vi "BatteryTestParsing.vi"() -> ()   [LabVIEW 2025]
panel:
  in  "Tab Control":enum32{"Page 1", "Page 2"}(tab)
  in  "charging 2":string="b'\\xe4\\xb3#\\xb5r\\x9c' bytearray(b'{\"topic\": \"/battery\", \"value\": 0.0}') {b'\\xe4\\xb3#\\xb5r\\x9c': [-31, 48611074]}\nb'\\xe4\\xb3#\\xb5r\\x9c' bytearray(b'{\"topic\": \"/battery\", \"value\": 0.2}') {b'\\xe4\\xb3#\\xb5r\\x9c': [-28, 48677187]}\nb'\\xe4\\xb3#\\xb5r\\x9c' bytearray(b'{\"topic\": \"/battery\", \"value\": 0.2}') {b'\\xe4\\xb3#\\xb5r\\x9c': [-31, 48743297]}\nb'\\xe4\\xb3#\\xb5r\\x9c' bytearray(b'{\"topic\": \"/battery\", \"value\": 0.7}') {b'\\xe4\\xb3#\\xb5r\\x9c': [-30, 48809408]}\nb'\\xe4\\xb3#\\xb5r\\x9c' bytearray(b'{\"topic\": \"/battery\", \"value\": 1.0}') {b'\\xe4\\xb3#\\xb5r\\x9c': [-40, 48875521]}\nb'\\xe4\\xb3#\\xb5r\\x9c' bytearray(b'{\"topic\": \"/battery\", \"value\": 1.1}') {b'\\xe4\\xb3#\\xb5r\\x9c': [-40, 48941632]}\nb'\\xe4\\xb3#\\xb5r\\x9c' bytearray(b'{\"topic\": \"/battery\", \"value\": 1.2}') {b'\\xe4\\xb3#\\xb5r\\x9c': [-40, 49007743]}\nb'\\xe4\\xb3#\\xb5r\\x9c' bytearray(b'{\"topic\": \"/battery\", \"value\": 1.4}') {b'\\xe4\\xb3#\\xb5r\\x9c': [-40, 49073858]}\nb'\\xe4\\xb3#\\xb5r\\x9c' bytearray(b'{\"topic\": \"/battery\", \"value\": 1.7}') {b'\\xe4\\xb3#\\xb5r\\x9c': [-40, 49139966]}\nb'\\xe4\\xb3#\\xb5r\\x9c' bytearray(b'{\"topic\": \"/battery\", \"value\": 2.0}') {b'\\xe4\\xb3#\\xb5r\\x9c': [-40, 49206079]}\nb'\\xe4\\xb3#\\xb5r\\x9c' bytearray(b'{\"topic\": \"/battery\", \"value\": 2.0}') {b'\\xe4\\xb3#\\xb5r\\x9c': [-40, 49272188]}\nb'\\xe4\\xb3#\\xb5r\\x9c' bytearray(b'{\"topic\": \"/battery\", \"value\": 2.0}') {b'\\xe4\\xb3#\\xb5r\\x9c': [-40, 49338302]}\nb'\\xe4\\xb3#\\xb5r\\x9c' bytearray(b'{\"topic\": \"/battery\", \"value\": 2.0}') {b'\\xe4\\xb3#\\xb5r\\x9c': [-36, 49404411]}\nb'\\xe4\\xb3#\\xb5r\\x9c' bytearray(b'{\"topic\": \"/battery\", \"value\": 2.0}') {b'\\xe4\\xb3#\\xb5r\\x9c': [-40, 49470522]}\nb'\\xe4\\xb3#\\xb5r\\x9c' bytearray(b'{\"topic\": \"/battery\", \"value\": 2.1}') {b'\\xe4\\xb3#\\xb5r\\x9c': [-40, 49536634]}\nb'\\xe4\\xb3#\\xb5r\\x9c' bytearray(b'{\"topic\": \"/battery\", \"value\": 2.1}') {b'\\xe4\\xb3#\\xb5r\\x9c': [-36, 49602745]}\nb'\\xe4\\xb3#\\xb5r\\x9c' bytearray(b'{\"topic\": \"/battery\", \"value\": 2.2}') {b'\\xe4\\xb3#\\xb5r\\x9c': [-36, 49668858]}\nb'\\xe4\\xb3#\\xb5r\\x9c' bytear}') {b'\\xe4\\xb3#\\xb5r\\x9c': [-36, 49734968]}\nb'\\xe4\\xb3#\\xb5r\\x9c' bytearray(b'{\"topic\": \"/battery\", \"value\": 2.3}') {b'\\xe4\\xb3#\\xb5r\\x9c': [-36, 49801080]}\nb'\\xe4\\xb3#\\xb5r\\x9c' bytearray(b'{\"topic\": \"/battery\", \"value\": 2.4}') {b'\\xe4\\xb3#\\xb5r\\x9c': [-39, 49867191]}\nb'\\xe4\\xb3#\\xb5r\\x9c' bytear': [-36, 50065525]}\nb'\\xe4\\xb3#\\xb5r\\x9c' bytearray(b'{\"topic\": \"/battery\", \"value\": 2.8}') {b'\\xe4\\xb3#\\xb5r\\x9c': [-36, 50131636]}\nb'\\xe4\\xb3#\\xb5r\\x9c' bytearray(b'{\"topic\": \"/battery\", \"value\": 2.8}') {b'\\xe4\\xb3#\\xb5r\\x9c': [-38, 50197750]}\nb'\\xe4\\xb3#\\xb5r\\x9c' bytearray(b'{\"topic\": \"/battery\", \"value\": 2.9}') {b'\\xe4\\xb3#\\xb5r\\x9c': [-36, 50263866]}\nb'\\xe4\\xb3#\\xb5r\\x9c' bytearray(b'{\"topic\": \"/battery\", \"value\": 2.9}') {b'\\xe4\\xb3#\\xb5r\\x9c': [-36, 50329983]}\nb'\\xe4\\xb3#\\xb5r\\x9c' bytearray(b'{\"topic\": \"/battery\", \"value\": 2.9}') {b'\\xe4\\xb3#\\xb5r\\x9c': [-36, 50396092]}\nb'\\xe4\\xb3#\\xb5r\\x9c' bytearray(b'{\"topic\": \"/battery\", \"value\": 3.0}') {b'\\xe4\\xb3#\\xb5r\\x9c': [-36, 50462203]}\nb'\\xe4\\xb3#\\xb5r\\x9c' bytearb'\\xe4\\xb3#\\xb5r\\x9c' bytearray(b'{\"topic\": \"/battery\", \"value\": 3.0}') {b'\\xe4\\xb3#\\xb5r\\x9c': [-35, 50792762]}\nb'\\xe4\\xb3#\\xb5r\\x9c' bytearray(b'{\"topic\": \"/battery\", \"value\": 2.9}') {b'\\xe4\\xb3#\\xb5r\\x9c': [-35, 50858871]}\nb'\\xe4\\xb3#\\xb5r\\x9c' bytearray(b'{\"topic\": \"/battery\", \"value\": 3.0}') {b'\\xe4\\xb3#\\xb5r\\x9c': [-35, 50924983]}\nb'\\xe4\\xb3#\\xb5r\\x9c' bytearray(b'{\"topic\": \"/battery\", \"value\": 3.0}') {b'\\xe4\\xb3#\\xb5r\\x9c': [-35, 50991096]}\nb'\\xe4\\xb3#\\xb5r\\x9c' bytearray(b'{\"topic\": \"/battery\", \"value\": 3.0}') {b'\\xe4\\xb3#\\xb5r\\x9c': [-35, 51057206]}\nb'\\xe4\\xb3#\\xb5r\\x9c' bytearray(b'{\"topic\": \"/battery\", \"value\": 3.0}') {b'\\xe4\\xb3#\\xb5r\\x9c': [-31, 51123317]}\nb'\\xe4\\xb3#\\xb5r\\x9c' bytearray(b'{\"topic\": \"/battery\", \"value\": 3.0}') {b'\\xe4\\xb3#\\xb5r\\x9c': [-31, 51189428]}\nb'\\xe4\\xb3#\\xb5r\\x9c' bytearray(b'{\"topic\": \"/battery\", \"value\": 3.0}') {b'\\xe4\\xb3#\\xb5r\\x9c': [-31, 51255540]}\nb'\\xe4\\xb3#\\xb5r\\x9c' bytearray(b'{\"topic\": \"/battery\", \"value\": 3.0}') {b'\\xe4\\xb3#\\xb5r\\x9c': [-30, 51321651]}\nb'\\xe4\\xb3#\\xb5r\\x9c' bytearray(b'{\"topic\": \"/battery\", \"value\": 3.0}') {b'\\xe4\\xb3#\\xb5r\\x9c': [-30, 51387763]}\nb'\\xe4\\xb3#\\xb5r\\x9c' bytearray(b'{\"topic\": \"/battery\", \"value\": 3.0}') {b'\\xe4\\xb3#\\xb5r\\x9c': [-31, 51453874]}\nb'\\xe4\\xb3#\\xb5r\\x9c' bytearray(b'{\"topic\": \"/battery\", \"value\": 3.0}') {b'\\xe4\\xb3#\\xb5r\\x9c': [-30, 51519986]}\nb'\\xe4\\xb3#\\xb5r\\x9c' bytearray(b'{\"topic\": \"/battery\", \"value\": 3.0}') {b'\\xe4\\xb3#\\xb5r\\x9c': [-30, 51586097]}\nb'\\xe4\\xb3#\\xb5r\\x9c' bytearray(b'{\"topic\": \"/battery\", \"value\": 3.1}') {b'\\xe4\\xb3#\\xb5r\\x9c': [-31, 51652210]}\nb'\\xe4\\xb3#\\xb5r\\x9c' bytearray(b'{\"topic\": \"/battery\", \"value\": 3.1}') {b'\\xe4\\xb3#\\xb5r\\x9c': [-31, 51718320]}\nb'\\xe4\\xb3#\\xb5r\\x9c' bytearray(b'{\"topic\": \"/battery\", \"value\": 3.2}') {b'\\xe4\\xb3#\\xb5r\\x9c': [-27, 51784433]}\nb'\\xe4\\xb3#\\xb5r\\x9c' bytearray(b'{\"topic\": \"/battery\", \"value\": 3.3}') {b'\\xe4\\xb3#\\xb5r\\x9c': [-26, 51850543]}\nb'\\xe4\\xb3#\\xb5r\\x9c' bytearray(b'{\"topic\": \"/battery\", \"value\": 3.5}') {b'\\xe4\\xb3#\\xb5r\\x9c': [-27, 51916654]}\nb'\\xe4\\xb3#\\xb5r\\x9c' bytearray(b'{\"topic\": \"/battery\", \"value\": 3.6}') {b'\\xe4\\xb3#\\xb5r\\x9c': [-25, 51982767]}\nb'\\xe4\\xb3#\\xb5r\\x9c' bytearray(b'{\"topic\": \"/battery\", \"value\": 3.7}') {b'\\xe4\\xb3#\\xb5r\\x9c': [-27, 52048877]}\nb'\\xe4\\xb3#\\xb5r\\x9c' bytearray(b'{\"topic\": \"/battery\", \"value\": 3.9}') {b'\\xe4\\xb3#\\xb5r\\x9c': [-25, 52114990]}\nb'\\xe4\\xb3#\\xb5r\\x9c' bytearray(b'{\"topic\": \"/battery\", \"value\": 4.0}') {b'\\xe4\\xb3#\\xb5r\\x9c': [-26, 52181100]}\nb'\\xe4\\xb3#\\xb5r\\x9c' bytearray(b'{\"topic\": \"/battery\", \"value\": 4.0}') {b'\\xe4\\xb3#\\xb5r\\x9c': [-25, 52247211]}\nb'\\xe4\\xb3#\\xb5r\\x9c' bytearray(b'{\"topic\": \"/battery\", \"value\": 4.0}') {b'\\xe4\\xb3#\\xb5r\\x9c': [-27, 52313322]}\nb'\\xe4\\xb3#\\xb5r\\x9c' bytearray(b'{\"topic\": \"/battery\", \"value\": 4.0}') {b'\\xe4\\xb3#\\xb5r\\x9c': [-27, 52379434]}\nb'\\xe4\\xb3#\\xb5r\\x9c' bytearray(b'{\"topic\": \"/battery\", \"value\": 4.0}') {b'\\xe4\\xb3#\\xb5r\\x9c': [-25, 52445546]}\nb'\\xe4\\xb3#\\xb5r\\x9c' bytearray(b'{\"topic\": \"/battery\", \"value\": 4.0}') {b'\\xe4\\xb3#\\xb5r\\x9c': [-26, 52511660]}\nb'\\xe4\\xb3#\\xb5r\\x9c' bytearray(b'{\"topic\": \"/battery\", \"value\": 4.0}') {b'\\xe4\\xb3#\\xb5r\\x9c': [-27, 52577769]}\nb'\\xe4\\xb3#\\xb5r\\x9c' bytearray(b'{\"topic\": \"/battery\", \"value\": 4.0}') {b'\\xe4\\xb3#\\xb5r\\x9c': [-27, 52643879]}\nb'\\xe4\\xb3#\\xb5r\\x9c' bytearray(b'{\"topic\": \"/battery\", \"value\": 4.0}') {b'\\xe4\\xb3#\\xb5r\\x9c': [-26, 52709991]}\nb'\\xe4\\xb3#\\xb5r\\x9c' bytearray(b'{\"topic\": \"/battery\", \"value\": 4.0}') {b'\\xe4\\xb3#\\xb5r\\x9c': [-25, 52776103]}\nb'\\xe4\\xb3#\\xb5r\\x9c' bytearray(b'{\"topic\": \"/battery\", \"value\": 4.0}') {b'\\xe4\\xb3#\\xb5r\\x9c': [-27, 52842213]}\nb'\\xe4\\xb3#\\xb5r\\x9c' bytearray(b'{\"topic\": \"/battery\", \"value\": 4.0}') {b'\\xe4\\xb3#\\xb5r\\x9c': [-27, 52908325]}\nb'\\xe4\\xb3#\\xb5r\\x9c' bytearray(b'{\"topic\": \"/battery\", \"value\": 4.0}') {b'\\xe4\\xb3#\\xb5r\\x9c': [-25, 52974436]}\nb'\\xe4\\xb3#\\xb5r\\x9c' bytearray(b'{\"topic\": \"/battery\", \"value\": 4.0}') {b'\\xe4\\xb3#\\xb5r\\x9c': [-27, 53040550]}\nb'\\xe4\\xb3#\\xb5r\\x9c' bytearray(b'{\"topic\": \"/battery\", \"value\": 4.0}') {b'\\xe4\\xb3#\\xb5r\\x9c': [-25, 53106660]}\nb'\\xe4\\xb3#\\xb5r\\x9c' bytearb'\\xe4\\xb3#\\xb5r\\x9c' bytearray(b'{\"topic\": \"/battery\", \"value\": 4.2}') {b'\\xe4\\xb3#\\xb5r\\x9c': [-25, 53238882]}\nb'\\xe4\\xb3#\\xb5r\\x9c' bytearray(b'{\"topic\": \"/battery\", \"value\": 4.3}') {b'\\xe4\\xb3#\\xb5r\\x9c': [-25, 53304993]}\nb'\\xe4\\xb3#\\xb5r\\x9c' bytearray(b'{\"topic\": \"/battery\", \"value\": 4.4}') {b'\\xe4\\xb3#\\xb5r\\x9c': [-25, 53371105]}\nb'\\xe4\\xb3#\\xb5r\\x9c' bytearpic\": \"/battery\", \"value\": 4.8}') {b'\\xe4\\xb3#\\xb5r\\x9c': [-27, 53635551]}\nb'\\xe4\\xb3#\\xb5r\\x9c' bytearray(b'{\"topic\": \"/battery\", \"value\": 4.9}') {b'\\xe4\\xb3#\\xb5r\\x9c': [-27, 53701662]}\nb'\\xe4\\xb3#\\xb5r\\x9c' bytearray(b'{\"topic\": \"/battery\", \"value\": 5.0}') {b'\\xe4\\xb3#\\xb5r\\x9c': [-25, 53767776]}\nb'\\xe4\\xb3#\\xb5r\\x9c' bytearray(b'{\"topic\": \"/battery\", \"value\": 5.0}') {b'\\xe4\\xb3#\\xb5r\\x9c': [-26, 53833885]}\nb'\\xe4\\xb3#\\xb5r\\x9c' bytearray(b'{\"topic\": \"/battery\", \"value\": 5.0}') {b'\\xe4\\xb3#\\xb5r\\x9c': [-27, 53899998]}\nb'\\xe4\\xb3#\\xb5r\\x9c' bytearray(b'{\"topic\": \"/battery\", \"value\": 5.0}') {b'\\xe4\\xb3#\\xb5r\\x9c': [-26, 53966107]}\nb'\\xe4\\xb3#\\xb5r\\x9c' bytearray(b'{\"topic\": \"/battery\", \"value\": 5.0}') {b'\\xe4\\xb3#\\xb5r\\x9c': [-25, 54032219]}\nb'\\xe4\\xb3#\\xb5r\\x9c' bytearray(b'{\"topic\": \"/battery\", \"value\": 5.0}') {b'\\xe4\\xb3#\\xb5r\\x9c': [-25, 54098330]}\nb'\\xe4\\xb3#\\xb5r\\x9c' bytearray(b'{\"topic\": \"/battery\", \"value\": 5.0}') {b'\\xe4\\xb3#\\xb5r\\x9c': [-27, 54164443]}\nb'\\xe4\\xb3#\\xb5r\\x9c' bytearray(b'{\"topic\": \"/battery\", \"value\": 5.0}') {b'\\xe4\\xb3#\\xb5r\\x9c': [-27, 54230553]}\nb'\\xe4\\xb3#\\xb5r\\x9c' bytearray(b'{\"topic\": \"/battery\", \"value\": 5.0}') {b'\\xe4\\xb3#\\xb5r\\x9c': [-27, 54296665]}\nb'\\xe4\\xb3#\\xb5r\\x9c' bytearray(b'{\"topic\": \"/battery\", \"value\": 5.0}') {b'\\xe4\\xb3#\\xb5r\\x9c': [-25, 54362776]}\nb'\\xe4\\xb3#\\xb5r\\x9c' bytearray(b'{\"topic\": \"/battery\", \"value\": 5.0}') {b'\\xe4\\xb3#\\xb5r\\x9c': [-27, 54428887]}\nb'\\xe4\\xb3#\\xb5r\\x9c' bytearray(b'{\"topic\": \"/battery\", \"value\": 5.0}') {b'\\xe4\\xb3#\\xb5r\\x9c': [-27, 54495000]}\nb'\\xe4\\xb3#\\xb5r\\x9c' bytearray(b'{\"topic\": \"/battery\", \"value\": 5.0}') {b'\\xe4\\xb3#\\xb5r\\x9c': [-25, 54561112]}\nb'\\xe4\\xb3#\\xb5r\\x9c' bytearray(b'{\"topic\": \"/battery\", \"value\": 5.0}') {b'\\xe4\\xb3#\\xb5r\\x9c': [-27, 54627233]}\nb'\\xe4\\xb3#\\xb5r\\x9c' bytearray(b'{\"topic\": \"/battery\", \"value\": 5.0}') {b'\\xe4\\xb3#\\xb5r\\x9c': [-27, 54693354]}\nb'\\xe4\\xb3#\\xb5r\\x9c' bytearray(b'{\"topic\": \"/battery\", \"value\": 5.0}') {b'\\xe4\\xb3#\\xb5r\\x9c': [-25, 54759468]}\nb'\\xe4\\xb3#\\xb5r\\x9c' bytearray(b'{\"topic\": \"/battery\", \"value\": 5.0}') {b'\\xe4\\xb3#\\xb5r\\x9c': [-25, 54825580]}\nb'\\xe4\\xb3#\\xb5r\\x9c' bytearray(b'{\"topic\": \"/battery\", \"value\": 5.0}') {b'\\xe4\\xb3#\\xb5r\\x9c': [-25, 54891687]}\nb'\\xe4\\xb3#\\xb5r\\x9c' bytearray(b'{\"topic\": \"/battery\", \"value\": 5.0}') {b'\\xe4\\xb3#\\xb5r\\x9c': [-26, 54957798]}\nb'\\xe4\\xb3#\\xb5r\\x9c' bytearray(b'{\"topic\": \"/battery\", \"value\": 5.0}') {b'\\xe4\\xb3#\\xb5r\\x9c': [-25, 55023910]}\nb'\\xe4\\xb3#\\xb5r\\x9c' bytearray(b'{\"topic\": \"/battery\", \"value\": 5.0}') {b'\\xe4\\xb3#\\xb5r\\x9c': [-27, 55090021]}\nb'\\xe4\\xb3#\\xb5r\\x9c' bytearray(b'{\"topic\": \"/battery\", \"value\": 5.0}') {b'\\xe4\\xb3#\\xb5r\\x9c': [-25, 55156133]}\nb'\\xe4\\xb3#\\xb5r\\x9c' bytearray(b'{\"topic\": \"/battery\", \"value\": 5.0}') {b'\\xe4\\xb3#\\xb5r\\x9c': [-27, 55222244]}\nb'\\xe4\\xb3#\\xb5r\\x9c' bytearray(b'{\"topic\": \"/battery\", \"value\": 5.1}') {b'\\xe4\\xb3#\\xb5r\\x9c': [-26, 55288355]}\nb'\\xe4\\xb3#\\xb5r\\x9c' bytearray(b'{\"topic\": \"/battery\", \"value\": 5.2}') {b'\\xe4\\xb3#\\xb5r\\x9c': [-27, 55354468]}\nb'\\xe4\\xb3#\\xb5r\\x9c' bytearray(b'{\"topic\": \"/battery\", \"value\": 5.2}') {b'\\xe4\\xb3#\\xb5r\\x9c': [-25, 55420578]}\nb'\\xe4\\xb3#\\xb5r\\x9c' bytearray(b'{\"topic\": \"/battery\", \"value\": 5.3}') {b'\\xe4\\xb3#\\xb5r\\x9c': [-25, 55486690]}\nb'\\xe4\\xb3#\\xb5r\\x9c' bytearray(b'{\"topic\": \"/battery\", \"value\": 5.4}') {b'\\xe4\\xb3#\\xb5r\\x9c': [-27, 55552801]}\nb'\\xe4\\xb3#\\xb5r\\x9c' bytearray(b'{\"topic\": \"/battery\", \"value\": 5.5}') {b'\\xe4\\xb3#\\xb5r\\x9c': [-25, 55618912]}\nb'\\xe4\\xb3#\\xb5r\\x9c' bytearray(b'{\"topic\": \"/battery\", \"value\": 5.6}') {b'\\xe4\\xb3#\\xb5r\\x9c': [-26, 55685025]}\nb'\\xe4\\xb3#\\xb5r\\x9c' bytearray(b'{\"topic\": \"/battery\", \"value\": 5.8}') {b'\\xe4\\xb3#\\xb5r\\x9c': [-25, 55751135]}\nb'\\xe4\\xb3#\\xb5r\\x9c' bytearray(b'{\"topic\": \"/battery\", \"value\": 5.9}') {b'\\xe4\\xb3#\\xb5r\\x9c': [-25, 55817246]}\nb'\\xe4\\xb3#\\xb5r\\x9c' bytearray(b'{\"topic\": \"/battery\", \"value\": 6.0}') {b'\\xe4\\xb3#\\xb5r\\x9c': [-27, 55883358]}\nb'\\xe4\\xb3#\\xb5r\\x9c' bytearray(b'{\"topic\": \"/battery\", \"value\": 6.0}') {b'\\xe4\\xb3#\\xb5r\\x9c': [-26, 55949470]}\nb'\\xe4\\xb3#\\xb5r\\x9c' bytearray(b'{\"topic\": \"/battery\", \"value\": 6.0}') {b'\\xe4\\xb3#\\xb5r\\x9c': [-27, 56015581]}\nb'\\xe4\\xb3#\\xb5r\\x9c' bytearray(b'{\"topic\": \"/battery\", \"value\": 6.1}') {b'\\xe4\\xb3#\\xb5r\\x9c': [-27, 56081693]}\nb'\\xe4\\xb3#\\xb5r\\x9c' bytearray(b'{\"topic\": \"/battery\", \"value\": 6.2}') {b'\\xe4\\xb3#\\xb5r\\x9c': [-25, 56147805]}\nb'\\xe4\\xb3#\\xb5r\\x9c' bytearray(b'{\"topic\": \"/battery\", \"value\": 6.3}') {b'\\xe4\\xb3#\\xb5r\\x9c': [-27, 56213915]}\nb'\\xe4\\xb3#\\xb5r\\x9c' bytearray(b'{\"topic\": \"/battery\", \"value\": 6.4}') {b'\\xe4\\xb3#\\xb5r\\x9c': [-28, 56280026]}\nb'\\xe4\\xb3#\\xb5r\\x9c' bytearray(b'{\"topic\": \"/battery\", \"value\": 6.5}') {b'\\xe4\\xb3#\\xb5r\\x9c': [-27, 56346138]}\nb'\\xe4\\xb3#\\xb5r\\x9c' bytearray(b'{\"topic\": \"/battery\", \"value\": 6.6}') {b'\\xe4\\xb3#\\xb5r\\x9c': [-26, 56412252]}\nb'\\xe4\\xb3#\\xb5r\\x9c' bytearray(b'{\"topic\": \"/battery\", \"value\": 6.7}') {b'\\xe4\\xb3#\\xb5r\\x9c': [-27, 56478360]}\nb'\\xe4\\xb3#\\xb5r\\x9c' bytearray(b'{\"topic\": \"/battery\", \"value\": 6.9}') {b'\\xe4\\xb3#\\xb5r\\x9c': [-27, 56544472]}\nb'\\xe4\\xb3#\\xb5r\\x9c' bytearray(b'{\"topic\": \"/battery\", \"value\": 7.0}') {b'\\xe4\\xb3#\\xb5r\\x9c': [-27, 56610583]}\nb'\\xe4\\xb3#\\xb5r\\x9c' bytearray(b'{\"topic\": \"/battery\", \"value\": 7.2}') {b'\\xe4\\xb3#\\xb5r\\x9c': [-25, 56676696]}\nb'\\xe4\\xb3#\\xb5r\\x9c' bytearray(b'{\"topic\": \"/battery\", \"value\": 7.3}') {b'\\xe4\\xb3#\\xb5r\\x9c': [-27, 56742810]}\nb'\\xe4\\xb3#\\xb5r\\x9c' bytearray(b'{\"topic\": \"/battery\", \"value\": 7.4}') {b'\\xe4\\xb3#\\xb5r\\x9c': [-25, 56808917]}\nb'\\xe4\\xb3#\\xb5r\\x9c' bytearray(b'{\"topic\": \"/battery\", \"value\": 7.6}') {b'\\xe4\\xb3#\\xb5r\\x9c': [-25, 56875029]}\nb'\\xe4\\xb3#\\xb5r\\x9c' bytearray(b'{\"topic\": \"/battery\", \"value\": 7.8}') {b'\\xe4\\xb3#\\xb5r\\x9c': [-25, 56941140]}\nb'\\xe4\\xb3#\\xb5r\\x9c' bytearray(b'{\"topic\": \"/battery\", \"value\": 8.0}') {b'\\xe4\\xb3#\\xb5r\\x9c': [-27, 57007252]}\nb'\\xe4\\xb3#\\xb5r\\x9c' bytearray(b'{\"topic\": \"/battery\", \"value\": 8.2}') {b'\\xe4\\xb3#\\xb5r\\x9c': [-26, 57073364]}\nb'\\xe4\\xb3#\\xb5r\\x9c' bytearray(b'{\"topic\": \"/battery\", \"value\": 8.4}') {b'\\xe4\\xb3#\\xb5r\\x9c': [-26, 57139474]}\nb'\\xe4\\xb3#\\xb5r\\x9c' bytearray(b'{\"topic\": \"/battery\", \"value\": 8.6}') {b'\\xe4\\xb3#\\xb5r\\x9c': [-25, 57205586]}\nb'\\xe4\\xb3#\\xb5r\\x9c' bytearray(b'{\"topic\": \"/battery\", \"value\": 8.9}') {b'\\xe4\\xb3#\\xb5r\\x9c': [-26, 57271697]}\nb'\\xe4\\xb3#\\xb5r\\x9c' bytearray(b'{\"topic\": \"/battery\", \"value\": 9.1}') {b'\\xe4\\xb3#\\xb5r\\x9c': [-25, 57337809]}\nb'\\xe4\\xb3#\\xb5r\\x9c' bytearray(b'{\"topic\": \"/battery\", \"value\": 9.3}') {b'\\xe4\\xb3#\\xb5r\\x9c': [-25, 57403920]}\nb'\\xe4\\xb3#\\xb5r\\x9c' bytearray(b'{\"topic\": \"/battery\", \"value\": 9.6}') {b'\\xe4\\xb3#\\xb5r\\x9c': [-26, 57470032]}\nb'\\xe4\\xb3#\\xb5r\\x9c' bytearray(b'{\"topic\": \"/battery\", \"value\": 9.8}') {b'\\xe4\\xb3#\\xb5r\\x9c': [-25, 57536143]}\nb'\\xe4\\xb3#\\xb5r\\x9c' bytearray(b'{\"topic\": \"/battery\", \"value\": 10.1}') {b'\\xe4\\xb3#\\xb5r\\x9c': [-27, 57602254]}\nb'\\xe4\\xb3#\\xb5r\\x9c' bytearray(b'{\"topic\": \"/battery\", \"value\": 10.4}') {b'\\xe4\\xb3#\\xb5r\\x9c': [-26, 57668366]}\nb'\\xe4\\xb3#\\xb5r\\x9c' bytearray(b'{\"topic\": \"/battery\", \"value\": 10.7}') {b'\\xe4\\xb3#\\xb5r\\x9c': [-26, 57734478]}\nb'\\xe4\\xb3#\\xb5r\\x9c' bytearray(b'{\"topic\": \"/battery\", \"value\": 11.0}') {b'\\xe4\\xb3#\\xb5r\\x9c': [-27, 57800590]}\nb'\\xe4\\xb3#\\xb5r\\x9c' byteb'\\xe4\\xb3#\\xb5r\\x9c' bytearray(b'{\"topic\": \"/battery\", \"value\": 13.0}') {b'\\xe4\\xb3#\\xb5r\\x9c': [-26, 58197260]}\nb'\\xe4\\xb3#\\xb5r\\x9c' bytearray(b'{\"topic\": \"/battery\", \"value\": 13.4}') {b'\\xe4\\xb3#\\xb5r\\x9c': [-25, 58263372]}\nb'\\xe4\\xb3#\\xb5r\\x9c' bytearray(b'{\"topic\": \"/battery\", \"value\": 13.7}') {b'\\xe4\\xb3#\\xb5r\\x9c': [-26, 58329480]}\nb'\\xe4\\xb3#\\xb5r\\x9c' bytearray(b'{\"topic\": \"/battery\", \"value\": 14.1}') {b'\\xe4\\xb3#\\xb5r\\x9c': [-26, 58395591]}\nb'\\xe4\\xb3#\\xb5r\\x9c' bytearray(b'{\"topic\": \"/battery\", \"value\": 14.5}') {b'\\xe4\\xb3#\\xb5r\\x9c': [-26, 58461702]}\nb'\\xe4\\xb3#\\xb5r\\x9c' byteb'\\xe4\\xb3#\\xb5r\\x9c' bytearray(b'{\"topic\": \"/battery\", \"value\": 15.3}') {b'\\xe4\\xb3#\\xb5r\\x9c': [-26, 58593925]}\nb'\\xe4\\xb3#\\xb5r\\x9c' bytearray(b'{\"topic\": \"/battery\", \"value\": 15.7}') {b'\\xe4\\xb3#\\xb5r\\x9c': [-26, 58660043]}\nb'\\xe4\\xb3#\\xb5r\\x9c' bytearray(b'{\"topic\": \"/battery\", \"value\": 16.1}') {b'\\xe4\\xb3#\\xb5r\\x9c': [-26, 58726158]}\nb'\\xe4\\xb3#\\xb5r\\x9c' bytearray(b'{\"topic\": \"/battery\", \"value\": 16.5}') {b'\\xe4\\xb3#\\xb5r\\x9c': [-26, 58792269]}\nb'\\xe4\\xb3#\\xb5r\\x9c' bytearray(b'{\"topic\": \"/battery\", \"value\": 17.0}') {b'\\xe4\\xb3#\\xb5r\\x9c': [-25, 58858382]}\nb'\\xe4\\xb3#\\xb5r\\x9c' bytearray(b'{\"topic\": \"/battery\", \"value\": 17.4}') {b'\\xe4\\xb3#\\xb5r\\x9c': [-25, 58924492]}\nb'\\xe4\\xb3#\\xb5r\\x9c' bytearray(b'{\"topic\": \"/battery\", \"value\": 17.8}') {b'\\xe4\\xb3#\\xb5r\\x9c': [-25, 58990604]}\nb'\\xe4\\xb3#\\xb5r\\x9c' bytearray(b'{\"topic\": \"/battery\", \"value\": 18.3}') {b'\\xe4\\xb3#\\xb5r\\x9c': [-25, 59056715]}\nb'\\xe4\\xb3#\\xb5r\\x9c' bytearray(b'{\"topic\": \"/battery\", \"value\": 18.7}') {b'\\xe4\\xb3#\\xb5r\\x9c': [-24, 59122826]}\nb'\\xe4\\xb3#\\xb5r\\x9c' bytearray(b'{\"topic\": \"/battery\", \"value\": 19.2}') {b'\\xe4\\xb3#\\xb5r\\x9c': [-25, 59188939]}\nb'\\xe4\\xb3#\\xb5r\\x9c' bytearray(b'{\"topic\": \"/battery\", \"value\": 19.6}') {b'\\xe4\\xb3#\\xb5r\\x9c': [-26, 59255051]}\nb'\\xe4\\xb3#\\xb5r\\x9c' bytearray(b'{\"topic\": \"/battery\", \"value\": 20.1}') {b'\\xe4\\xb3#\\xb5r\\x9c': [-26, 59321161]}\nb'\\xe4\\xb3#\\xb5r\\x9c' bytearray(b'{\"topic\": \"/battery\", \"value\": 20.6}') {b'\\xe4\\xb3#\\xb5r\\x9c': [-25, 59387272]}\nb'\\xe4\\xb3#\\xb5r\\x9c' bytearray(b'{\"topic\": \"/battery\", \"value\": 21.0}') {b'\\xe4\\xb3#\\xb5r\\x9c': [-25, 59453383]}\nb'\\xe4\\xb3#\\xb5r\\x9c' bytearray(b'{\"topic\": \"/battery\", \"value\": 21.5}') {b'\\xe4\\xb3#\\xb5r\\x9c': [-26, 59519495]}\nb'\\xe4\\xb3#\\xb5r\\x9c' bytearray(b'{\"topic\": \"/battery\", \"value\": 22.0}') {b'\\xe4\\xb3#\\xb5r\\x9c': [-25, 59585608]}\nb'\\xe4\\xb3#\\xb5r\\x9c' bytearray(b'{\"topic\": \"/battery\", \"value\": 22.5}') {b'\\xe4\\xb3#\\xb5r\\x9c': [-26, 59651718]}\nb'\\xe4\\xb3#\\xb5r\\x9c' bytearray(b'{\"topic\": \"/battery\", \"value\": 23.0}') {b'\\xe4\\xb3#\\xb5r\\x9c': [-26, 59717829]}\nb'\\xe4\\xb3#\\xb5r\\x9c' bytearray(b'{\"topic\": \"/battery\", \"value\": 23.5}') {b'\\xe4\\xb3#\\xb5r\\x9c': [-26, 59783941]}\nb'\\xe4\\xb3#\\xb5r\\x9c' bytearray(b'{\"topic\": \"/battery\", \"value\": 24.1}') {b'\\xe4\\xb3#\\xb5r\\x9c': [-25, 59850052]}\nb'\\xe4\\xb3#\\xb5r\\x9c' bytearray(b'{\"topic\": \"/battery\", \"value\": 24.6}') {b'\\xe4\\xb3#\\xb5r\\x9c': [-26, 59916164]}\nb'\\xe4\\xb3#\\xb5r\\x9c' bytearray(b'{\"topic\": \"/battery\", \"value\": 25.2}') {b'\\xe4\\xb3#\\xb5r\\x9c': [-25, 59982275]}\nb'\\xe4\\xb3#\\xb5r\\x9c' bytearray(b'{\"topic\": \"/battery\", \"value\": 25.7}') {b'\\xe4\\xb3#\\xb5r\\x9c': [-26, 60048387]}\nb'\\xe4\\xb3#\\xb5r\\x9c' bytearray(b'{\"topic\": \"/battery\", \"value\": 26.3}') {b'\\xe4\\xb3#\\xb5r\\x9c': [-25, 60114498]}\nb'\\xe4\\xb3#\\xb5r\\x9c' bytearray(b'{\"topic\": \"/battery\", \"value\": 26.8}') {b'\\xe4\\xb3#\\xb5r\\x9c': [-25, 60180609]}\nb'\\xe4\\xb3#\\xb5r\\x9c' bytearray(b'{\"topic\": \"/battery\", \"value\": 27.4}') {b'\\xe4\\xb3#\\xb5r\\x9c': [-26, 60246720]}\nb'\\xe4\\xb3#\\xb5r\\x9c' bytearray(b'{\"topic\": \"/battery\", \"value\": 28.0}') {b'\\xe4\\xb3#\\xb5r\\x9c': [-25, 60312838]}\nb'\\xe4\\xb3#\\xb5r\\x9c' bytearray(b'{\"topic\": \"/battery\", \"value\": 28.6}') {b'\\xe4\\xb3#\\xb5r\\x9c': [-24, 60378954]}\nb'\\xe4\\xb3#\\xb5r\\x9c' bytearray(b'{\"topic\": \"/battery\", \"value\": 29.2}') {b'\\xe4\\xb3#\\xb5r\\x9c': [-25, 60445064]}\nb'\\xe4\\xb3#\\xb5r\\x9c' bytearray(b'{\"topic\": \"/battery\", \"value\": 29.8}') {b'\\xe4\\xb3#\\xb5r\\x9c': [-26, 60511176]}\nb'\\xe4\\xb3#\\xb5r\\x9c' bytearray(b'{\"topic\": \"/battery\", \"value\": 30.4}') {b'\\xe4\\xb3#\\xb5r\\x9c': [-25, 60577287]}\nb'\\xe4\\xb3#\\xb5r\\x9c' bytearray(b'{\"topic\": \"/battery\", \"value\": 31.0}') {b'\\xe4\\xb3#\\xb5r\\x9c': [-26, 60643399]}\nb'\\xe4\\xb3#\\xb5r\\x9c' bytearray(b'{\"topic\": \"/battery\", \"value\": 31.7}') {b'\\xe4\\xb3#\\xb5r\\x9c': [-25, 60709515]}\nb'\\xe4\\xb3#\\xb5r\\x9c' bytearray(b'{\"topic\": \"/battery\", \"value\": 32.3}') {b'\\xe4\\xb3#\\xb5r\\x9c': [-24, 60775621]}\nb'\\xe4\\xb3#\\xb5r\\x9c' bytearray(b'{\"topic\": \"/battery\", \"value\": 33.0}') {b'\\xe4\\xb3#\\xb5r\\x9c': [-26, 60841734]}\nb'\\xe4\\xb3#\\xb5r\\x9c' bytearray(b'{\"topic\": \"/battery\", \"value\": 33.6}') {b'\\xe4\\xb3#\\xb5r\\x9c': [-26, 60907845]}\nb'\\xe4\\xb3#\\xb5r\\x9c' bytearray(b'{\"topic\": \"/battery\", \"value\": 34.3}') {b'\\xe4\\xb3#\\xb5r\\x9c': [-25, 60973957]}\nb'\\xe4\\xb3#\\xb5r\\x9c' bytearray(b'{\"topic\": \"/battery\", \"value\": 35.0}') {b'\\xe4\\xb3#\\xb5r\\x9c': [-26, 61040068]}\nb'\\xe4\\xb3#\\xb5r\\x9c' bytearray(b'{\"topic\": \"/battery\", \"value\": 35.6}') {b'\\xe4\\xb3#\\xb5r\\x9c': [-26, 61106181]}\nb'\\xe4\\xb3#\\xb5r\\x9c' bytearray(b'{\"topic\": \"/battery\", \"value\": 36.3}') {b'\\xe4\\xb3#\\xb5r\\x9c': [-25, 61172295]}\nb'\\xe4\\xb3#\\xb5r\\x9c' bytearray(b'{\"topic\": \"/battery\", \"value\": 37.0}') {b'\\xe4\\xb3#\\xb5r\\x9c': [-26, 61238408]}\nb'\\xe4\\xb3#\\xb5r\\x9c' bytearray(b'{\"topic\": \"/battery\", \"value\": 37.7}') {b'\\xe4\\xb3#\\xb5r\\x9c': [-25, 61304522]}\nb'\\xe4\\xb3#\\xb5r\\x9c' bytearray(b'{\"topic\": \"/battery\", \"value\": 38.4}') {b'\\xe4\\xb3#\\xb5r\\x9c': [-26, 61370635]}\nb'\\xe4\\xb3#\\xb5r\\x9c' bytearray(b'{\"topic\": \"/battery\", \"value\": 39.1}') {b'\\xe4\\xb3#\\xb5r\\x9c': [-26, 61436745]}\nb'\\xe4\\xb3#\\xb5r\\x9c' bytearray(b'{\"topic\": \"/battery\", \"value\": 39.8}') {b'\\xe4\\xb3#\\xb5r\\x9c': [-25, 61502857]}\nb'\\xe4\\xb3#\\xb5r\\x9c' bytearray(b'{\"topic\": \"/battery\", \"value\": 40.5}') {b'\\xe4\\xb3#\\xb5r\\x9c': [-26, 61568968]}\nb'\\xe4\\xb3#\\xb5r\\x9c' bytearray(b'{\"topic\": \"/battery\", \"value\": 41.3}') {b'\\xe4\\xb3#\\xb5r\\x9c': [-24, 61635079]}\nb'\\xe4\\xb3#\\xb5r\\x9c' bytearray(b'{\"topic\": \"/battery\", \"value\": 42.0}') {b'\\xe4\\xb3#\\xb5r\\x9c': [-26, 61701191]}\nb'\\xe4\\xb3#\\xb5r\\x9c' bytearray(b'{\"topic\": \"/battery\", \"value\": 42.7}') {b'\\xe4\\xb3#\\xb5r\\x9c': [-26, 61767302]}\nb'\\xe4\\xb3#\\xb5r\\x9c' bytearray(b'{\"topic\": \"/battery\", \"value\": 43.4}') {b'\\xe4\\xb3#\\xb5r\\x9c': [-25, 61833414]}\nb'\\xe4\\xb3#\\xb5r\\x9c' bytearray(b'{\"topic\": \"/battery\", \"value\": 44.2}') {b'\\xe4\\xb3#\\xb5r\\x9c': [-26, 61899525]}\nb'\\xe4\\xb3#\\xb5r\\x9c' bytearray(b'{\"topic\": \"/battery\", \"value\": 44.9}') {b'\\xe4\\xb3#\\xb5r\\x9c': [-25, 61965638]}\nb'\\xe4\\xb3#\\xb5r\\x9c' bytearray(b'{\"topic\": \"/battery\", \"value\": 45.6}') {b'\\xe4\\xb3#\\xb5r\\x9c': [-26, 62031748]}\nb'\\xe4\\xb3#\\xb5r\\x9c' bytearray(b'{\"topic\": \"/battery\", \"value\": 46.3}') {b'\\xe4\\xb3#\\xb5r\\x9c': [-26, 62097859]}\nb'\\xe4\\xb3#\\xb5r\\x9c' bytearray(b'{\"topic\": \"/battery\", \"value\": 47.0}') {b'\\xe4\\xb3#\\xb5r\\x9c': [-26, 62163971]}\nb'\\xe4\\xb3#\\xb5r\\x9c' bytearray(b'{\"topic\": \"/battery\", \"value\": 47.7}') {b'\\xe4\\xb3#\\xb5r\\x9c': [-25, 62230082]}\nb'\\xe4\\xb3#\\xb5r\\x9c' bytearray(b'{\"topic\": \"/battery\", \"value\": 48.5}') {b'\\xe4\\xb3#\\xb5r\\x9c': [-24, 62296194]}\nb'\\xe4\\xb3#\\xb5r\\x9c' bytearray(b'{\"topic\": \"/battery\", \"value\": 49.2}') {b'\\xe4\\xb3#\\xb5r\\x9c': [-26, 62362305]}\nb'\\xe4\\xb3#\\xb5r\\x9c' bytearray(b'{\"topic\": \"/battery\", \"value\": 49.9}') {b'\\xe4\\xb3#\\xb5r\\x9c': [-26, 62428416]}\nb'\\xe4\\xb3#\\xb5r\\x9c' bytearray(b'{\"topic\": \"/battery\", \"value\": 50.6}') {b'\\xe4\\xb3#\\xb5r\\x9c': [-25, 62494528]}\nb'\\xe4\\xb3#\\xb5r\\x9c' bytearray(b'{\"topic\": \"/battery\", \"value\": 51.3}') {b'\\xe4\\xb3#\\xb5r\\x9c': [-25, 62560640]}\nb'\\xe4\\xb3#\\xb5r\\x9c' bytearray(b'{\"topic\": \"/battery\", \"value\": 52.0}') {b'\\xe4\\xb3#\\xb5r\\x9c': [-26, 62626751]}\nb'\\xe4\\xb3#\\xb5r\\x9c' bytearray(b'{\"topic\": \"/battery\", \"value\": 52.7}') {b'\\xe4\\xb3#\\xb5r\\x9c': [-25, 62692862]}\nb'\\xe4\\xb3#\\xb5r\\x9c' bytearray(b'{\"topic\": \"/battery\", \"value\": 53.4}') {b'\\xe4\\xb3#\\xb5r\\x9c': [-25, 62758973]}\nb'\\xe4\\xb3#\\xb5r\\x9c' bytearray(b'{\"topic\": \"/battery\", \"value\": 54.1}') {b'\\xe4\\xb3#\\xb5r\\x9c': [-26, 62825085]}\nb'\\xe4\\xb3#\\xb5r\\x9c' bytearray(b'{\"topic\": \"/battery\", \"value\": 54.8}') {b'\\xe4\\xb3#\\xb5r\\x9c': [-26, 62891196]}\nb'\\xe4\\xb3#\\xb5r\\x9c' bytearray(b'{\"topic\": \"/battery\", \"value\": 55.5}') {b'\\xe4\\xb3#\\xb5r\\x9c': [-26, 62957312]}\nb'\\xe4\\xb3#\\xb5r\\x9c' bytearray(b'{\"topic\": \"/battery\", \"value\": 56.2}') {b'\\xe4\\xb3#\\xb5r\\x9c': [-19, 63023419]}\nb'\\xe4\\xb3#\\xb5r\\x9c' bytearray(b'{\"topic\": \"/battery\", \"value\": 56.9}') {b'\\xe4\\xb3#\\xb5r\\x9c': [-20, 63089530]}\nb'\\xe4\\xb3#\\xb5r\\x9c' bytearray(b'{\"topic\": \"/battery\", \"value\": 57.6}') {b'\\xe4\\xb3#\\xb5r\\x9c': [-20, 63155642]}\nb'\\xe4\\xb3#\\xb5r\\x9c' bytearray(b'{\"topic\": \"/battery\", \"value\": 58.3}') {b'\\xe4\\xb3#\\xb5r\\x9c': [-20, 63221755]}\nb'\\xe4\\xb3#\\xb5r\\x9c' bytearray(b'{\"topic\": \"/battery\", \"value\": 59.0}') {b'\\xe4\\xb3#\\xb5r\\x9c': [-20, 63287867]}\nb'\\xe4\\xb3#\\xb5r\\x9c' bytearray(b'{\"topic\": \"/battery\", \"value\": 59.6}') {b'\\xe4\\xb3#\\xb5r\\x9c': [-18, 63353976]}\nb'\\xe4\\xb3#\\xb5r\\x9c' bytearray(b'{\"topic\": \"/battery\", \"value\": 60.3}') {b'\\xe4\\xb3#\\xb5r\\x9c': [-18, 63420088]}\nb'\\xe4\\xb3#\\xb5r\\x9c' bytearray(b'{\"topic\": \"/battery\", \"value\": 61.0}') {b'\\xe4\\xb3#\\xb5r\\x9c': [-19, 63486199]}\nb'\\xe4\\xb3#\\xb5r\\x9c' bytearray(b'{\"topic\": \"/battery\", \"value\": 61.7}') {b'\\xe4\\xb3#\\xb5r\\x9c': [-18, 63552311]}\nb'\\xe4\\xb3#\\xb5r\\x9c' bytearray(b'{\"topic\": \"/battery\", \"value\": 62.4}') {b'\\xe4\\xb3#\\xb5r\\x9c': [-18, 63618422]}\nb'\\xe4\\xb3#\\xb5r\\x9c' bytearray(b'{\"topic\": \"/battery\", \"value\": 63.1}') {b'\\xe4\\xb3#\\xb5r\\x9c': [-19, 63684533]}\nb'\\xe4\\xb3#\\xb5r\\x9c' bytearray(b'{\"topic\": \"/battery\", \"value\": 63.8}') {b'\\xe4\\xb3#\\xb5r\\x9c': [-19, 63750646]}\nb'\\xe4\\xb3#\\xb5r\\x9c' bytearray(b'{\"topic\": \"/battery\", \"value\": 64.5}') {b'\\xe4\\xb3#\\xb5r\\x9c': [-18, 63816756]}\nb'\\xe4\\xb3#\\xb5r\\x9c' bytearray(b'{\"topic\": \"/battery\", \"value\": 65.2}') {b'\\xe4\\xb3#\\xb5r\\x9c': [-19, 63882867]}\nb'\\xe4\\xb3#\\xb5r\\x9c' bytearray(b'{\"topic\": \"/battery\", \"value\": 65.9}') {b'\\xe4\\xb3#\\xb5r\\x9c': [-22, 63948978]}\nb'\\xe4\\xb3#\\xb5r\\x9c' bytearray(b'{\"topic\": \"/battery\", \"value\": 66.5}') {b'\\xe4\\xb3#\\xb5r\\x9c': [-21, 64015090]}\nb'\\xe4\\xb3#\\xb5r\\x9c' bytearray(b'{\"topic\": \"/battery\", \"value\": 67.2}') {b'\\xe4\\xb3#\\xb5r\\x9c': [-21, 64081205]}\nb'\\xe4\\xb3#\\xb5r\\x9c' bytearray(b'{\"topic\": \"/battery\", \"value\": 67.9}') {b'\\xe4\\xb3#\\xb5r\\x9c': [-20, 64147314]}\nb'\\xe4\\xb3#\\xb5r\\x9c' bytearray(b'{\"topic\": \"/battery\", \"value\": 68.6}') {b'\\xe4\\xb3#\\xb5r\\x9c': [-20, 64213424]}\nb'\\xe4\\xb3#\\xb5r\\x9c' bytearray(b'{\"topic\": \"/battery\", \"value\": 69.3}') {b'\\xe4\\xb3#\\xb5r\\x9c': [-20, 64279536]}\nb'\\xe4\\xb3#\\xb5r\\x9c' bytearray(b'{\"topic\": \"/battery\", \"value\": 70.0}') {b'\\xe4\\xb3#\\xb5r\\x9c': [-20, 64345648]}\nb'\\xe4\\xb3#\\xb5r\\x9c' bytearray(b'{\"topic\": \"/battery\", \"value\": 70.7}') {b'\\xe4\\xb3#\\xb5r\\x9c': [-20, 64411762]}\nb'\\xe4\\xb3#\\xb5r\\x9c' bytearray(b'{\"topic\": \"/battery\", \"value\": 71.4}') {b'\\xe4\\xb3#\\xb5r\\x9c': [-20, 64477871]}\nb'\\xe4\\xb3#\\xb5r\\x9c' bytearray(b'{\"topic\": \"/battery\", \"value\": 72.0}') {b'\\xe4\\xb3#\\xb5r\\x9c': [-20, 64543981]}\nb'\\xe4\\xb3#\\xb5r\\x9c' bytearray(b'{\"topic\": \"/battery\", \"value\": 72.7}') {b'\\xe4\\xb3#\\xb5r\\x9c': [-20, 64610093]}\nb'\\xe4\\xb3#\\xb5r\\x9c' bytearray(b'{\"topic\": \"/battery\", \"value\": 73.3}') {b'\\xe4\\xb3#\\xb5r\\x9c': [-20, 64676204]}\nb'\\xe4\\xb3#\\xb5r\\x9c' bytearray(b'{\"topic\": \"/battery\", \"value\": 74.0}') {b'\\xe4\\xb3#\\xb5r\\x9c': [-20, 64742316]}\nb'\\xe4\\xb3#\\xb5r\\x9c' bytearray(b'{\"topic\": \"/battery\", \"value\": 74.6}') {b'\\xe4\\xb3#\\xb5r\\x9c': [-20, 64808430]}\nb'\\xe4\\xb3#\\xb5r\\x9c' bytearray(b'{\"topic\": \"/battery\", \"value\": 75.2}') {b'\\xe4\\xb3#\\xb5r\\x9c': [-20, 64874538]}\nb'\\xe4\\xb3#\\xb5r\\x9c' byteb3#\\xb5r\\x9c' bytearray(b'{\"topic\": \"/battery\", \"value\": 79.9}') {b'\\xe4\\xb3#\\xb5r\\x9c': [-20, 65403429]}\nb'\\xe4\\xb3#\\xb5r\\x9c' bytearray(b'{\"topic\": \"/battery\", \"value\": 80.4}') {b'\\xe4\\xb3#\\xb5r\\x9c': [-20, 65469541]}\nb'\\xe4\\xb3#\\xb5r\\x9c' bytearray(b'{\"topic\": \"/battery\", \"value\": 81.0}') {b'\\xe4\\xb3#\\xb5r\\x9c': [-20, 65535653]}\nb'\\xe4\\xb3#\\xb5r\\x9c' byte\", \"value\": 81.5}') {b'\\xe4\\xb3#\\xb5r\\x9c': [-20, 65601763]}\nb'\\xe4\\xb3#\\xb5r\\x9c' bytearray(b'{\"topic\": \"/battery\", \"value\": 82.1}') {b'\\xe4\\xb3#\\xb5r\\x9c': [-20, 65667875]}\nb'\\xe4\\xb3#\\xb5r\\x9c' bytearray(b'{\"topic\": \"/battery\", \"value\": 82.6}') {b'\\xe4\\xb3#\\xb5r\\x9c': [-20, 65733988]}\nb'\\xe4\\xb3#\\xb5r\\x9c' bytearray(b'{\"topic\": \"/battery\", \"value\": 83.1}') {b'\\xe4\\xb3#\\xb5r\\x9c': [-20, 65800098]}\nb'\\xe4\\xb3#\\xb5r\\x9c' bytearray(b'{\"topic\": \"/battery\", \"value\": 83.7}') {b'\\xe4\\xb3#\\xb5r\\x9c': [-20, 65866209]}\nb'\\xe4\\xb3#\\xb5r\\x9c' bytearray(b'{\"topic\": \"/battery\", \"value\": 84.2}') {b'\\xe4\\xb3#\\xb5r\\x9c': [-20, 65932321]}\nb'\\xe4\\xb3#\\xb5r\\x9c' bytearray(b'{\"topic\": \"/battery\", \"value\": 84.7}') {b'\\xe4\\xb3#\\xb5r\\x9c': [-20, 65998434]}\nb'\\xe4\\xb3#\\xb5r\\x9c' bytearray(b'{\"topic\": \"/battery\", \"value\": 85.2}') {b'\\xe4\\xb3#\\xb5r\\x9c': [-20, 66064543]}\nb'\\xe4\\xb3#\\xb5r\\x9c' bytearray(b'{\"topic\": \"/battery\", \"value\": 85.8}') {b'\\xe4\\xb3#\\xb5r\\x9c': [-20, 66130655]}\nb'\\xe4\\xb3#\\xb5r\\x9c' bytearray(b'{\"topic\": \"/battery\", \"value\": 86.3}') {b'\\xe4\\xb3#\\xb5r\\x9c': [-20, 66196766]}\nb'\\xe4\\xb3#\\xb5r\\x9c' bytearray(b'{\"topic\": \"/battery\", \"value\": 86.8}') {b'\\xe4\\xb3#\\xb5r\\x9c': [-20, 66262877]}\nb'\\xe4\\xb3#\\xb5r\\x9c' bytearray(b'{\"topic\": \"/battery\", \"value\": 87.3}') {b'\\xe4\\xb3#\\xb5r\\x9c': [-20, 66328990]}\nb'\\xe4\\xb3#\\xb5r\\x9c' bytearray(b'{\"topic\": \"/battery\", \"value\": 87.9}') {b'\\xe4\\xb3#\\xb5r\\x9c': [-20, 66395100]}\nb'\\xe4\\xb3#\\xb5r\\x9c' bytearray(b'{\"topic\": \"/battery\", \"value\": 88.4}') {b'\\xe4\\xb3#\\xb5r\\x9c': [-20, 66461212]}\nb'\\xe4\\xb3#\\xb5r\\x9c' bytearray(b'{\"topic\": \"/battery\", \"value\": 88.9}') {b'\\xe4\\xb3#\\xb5r\\x9c': [-20, 66527323]}\nb'\\xe4\\xb3#\\xb5r\\x9c' bytearray(b'{\"topic\": \"/battery\", \"value\": 89.5}') {b'\\xe4\\xb3#\\xb5r\\x9c': [-20, 66593434]}\nb'\\xe4\\xb3#\\xb5r\\x9c' bytearray(b'{\"topic\": \"/battery\", \"value\": 90.0}') {b'\\xe4\\xb3#\\xb5r\\x9c': [-20, 66659546]}\nb'\\xe4\\xb3#\\xb5r\\x9c' bytearray(b'{\"topic\": \"/battery\", \"value\": 90.5}') {b'\\xe4\\xb3#\\xb5r\\x9c': [-20, 66725657]}\nb'\\xe4\\xb3#\\xb5r\\x9c' bytearray(b'{\"topic\": \"/battery\", \"value\": 91.0}') {b'\\xe4\\xb3#\\xb5r\\x9c': [-20, 66791769]}\nb'\\xe4\\xb3#\\xb5r\\x9c' bytearray(b'{\"topic\": \"/battery\", \"value\": 91.4}') {b'\\xe4\\xb3#\\xb5r\\x9c': [-20, 66857880]}\nb'\\xe4\\xb3#\\xb5r\\x9c' bytearray(b'{\"topic\": \"/battery\", \"value\": 91.9}') {b'\\xe4\\xb3#\\xb5r\\x9c': [-20, 66923991]}\nb'\\xe4\\xb3#\\xb5r\\x9c' bytearray(b'{\"topic\": \"/battery\", \"value\": 92.3}') {b'\\xe4\\xb3#\\xb5r\\x9c': [-20, 66990107]}\nb'\\xe4\\xb3#\\xb5r\\x9c' bytearray(b'{\"topic\": \"/battery\", \"value\": 92.8}') {b'\\xe4\\xb3#\\xb5r\\x9c': [-20, 67056214]}\nb'\\xe4\\xb3#\\xb5r\\x9c' bytearray(b'{\"topic\": \"/battery\", \"value\": 93.2}') {b'\\xe4\\xb3#\\xb5r\\x9c': [-20, 67122326]}\nb'\\xe4\\xb3#\\xb5r\\x9c' bytearray(b'{\"topic\": \"/battery\", \"value\": 93.5}') {b'\\xe4\\xb3#\\xb5r\\x9c': [-20, 67188437]}\nb'\\xe4\\xb3#\\xb5r\\x9c' bytearray(b'{\"topic\": \"/battery\", \"value\": 93.9}') {b'\\xe4\\xb3#\\xb5r\\x9c': [-20, 67254548]}\nb'\\xe4\\xb3#\\xb5r\\x9c' bytearray(b'{\"topic\": \"/battery\", \"value\": 94.3}') {b'\\xe4\\xb3#\\xb5r\\x9c': [-20, 67320660]}\nb'\\xe4\\xb3#\\xb5r\\x9c' bytearray(b'{\"topic\": \"/battery\", \"value\": 94.6}') {b'\\xe4\\xb3#\\xb5r\\x9c': [-20, 67386771]}\nb'\\xe4\\xb3#\\xb5r\\x9c' bytearray(b'{\"topic\": \"/battery\", \"value\": 94.9}') {b'\\xe4\\xb3#\\xb5r\\x9c': [-20, 67452885]}\nb'\\xe4\\xb3#\\xb5r\\x9c' bytearray(b'{\"topic\": \"/battery\", \"value\": 95.3}') {b'\\xe4\\xb3#\\xb5r\\x9c': [-20, 67518994]}\nb'\\xe4\\xb3#\\xb5r\\x9c' bytearray(b'{\"topic\": \"/battery\", \"value\": 95.6}') {b'\\xe4\\xb3#\\xb5r\\x9c': [-20, 67585105]}\nb'\\xe4\\xb3#\\xb5r\\x9c' bytearray(b'{\"topic\": \"/battery\", \"value\": 95.9}') {b'\\xe4\\xb3#\\xb5r\\x9c': [-20, 67651217]}\nb'\\xe4\\xb3#\\xb5r\\x9c' bytearray(b'{\"topic\": \"/battery\", \"value\": 96.1}') {b'\\xe4\\xb3#\\xb5r\\x9c': [-20, 67717328]}\nb'\\xe4\\xb3#\\xb5r\\x9c' bytearray(b'{\"topic\": \"/battery\", \"value\": 96.3}') {b'\\xe4\\xb3#\\xb5r\\x9c': [-20, 67783439]}\nb'\\xe4\\xb3#\\xb5r\\x9c' bytearray(b'{\"topic\": \"/battery\", \"value\": 96.5}') {b'\\xe4\\xb3#\\xb5r\\x9c': [-20, 67849551]}\nb'\\xe4\\xb3#\\xb5r\\x9c' bytearray(b'{\"topic\": \"/battery\", \"value\": 96.7}') {b'\\xe4\\xb3#\\xb5r\\x9c': [-20, 67915662]}\nb'\\xe4\\xb3#\\xb5r\\x9c' bytearray(b'{\"topic\": \"/battery\", \"value\": 96.9}') {b'\\xe4\\xb3#\\xb5r\\x9c': [-20, 67981774]}\nb'\\xe4\\xb3#\\xb5r\\x9c' bytearray(b'{\"topic\": \"/battery\", \"value\": 97.0}') {b'\\xe4\\xb3#\\xb5r\\x9c': [-20, 68047885]}\nb'\\xe4\\xb3#\\xb5r\\x9c' bytearray(b'{\"topic\": \"/battery\", \"value\": 97.1}') {b'\\xe4\\xb3#\\xb5r\\x9c': [-20, 68113997]}\nb'\\xe4\\xb3#\\xb5r\\x9c' bytearray(b'{\"topic\": \"/battery\", \"value\": 97.3}') {b'\\xe4\\xb3#\\xb5r\\x9c': [-20, 68180108]}\nb'\\xe4\\xb3#\\xb5r\\x9c' bytearray(b'{\"topic\": \"/battery\", \"value\": 97.4}') {b'\\xe4\\xb3#\\xb5r\\x9c': [-20, 68246221]}\nb'\\xe4\\xb3#\\xb5r\\x9c' bytearray(b'{\"topic\": \"/battery\", \"value\": 97.5}') {b'\\xe4\\xb3#\\xb5r\\x9c': [-20, 68312331]}\nb'\\xe4\\xb3#\\xb5r\\x9c' bytearray(b'{\"topic\": \"/battery\", \"value\": 97.6}') {b'\\xe4\\xb3#\\xb5r\\x9c': [-20, 68378442]}\nb'\\xe4\\xb3#\\xb5r\\x9c' bytearray(b'{\"topic\": \"/battery\", \"value\": 97.7}') {b'\\xe4\\xb3#\\xb5r\\x9c': [-20, 68444553]}\nb'\\xe4\\xb3#\\xb5r\\x9c' bytearray(b'{\"topic\": \"/battery\", \"value\": 97.8}') {b'\\xe4\\xb3#\\xb5r\\x9c': [-20, 68510665]}\nb'\\xe4\\xb3#\\xb5r\\x9c' bytearray(b'{\"topic\": \"/battery\", \"value\": 98.0}') {b'\\xe4\\xb3#\\xb5r\\x9c': [-20, 68576776]}\nb'\\xe4\\xb3#\\xb5r\\x9c' bytearray(b'{\"topic\": \"/battery\", \"value\": 98.0}') {b'\\xe4\\xb3#\\xb5r\\x9c': [-20, 68642887]}\nb'\\xe4\\xb3#\\xb5r\\x9c' bytearray(b'{\"topic\": \"/battery\", \"value\": 98.0}') {b'\\xe4\\xb3#\\xb5r\\x9c': [-20, 68709000]}\nb'\\xe4\\xb3#\\xb5r\\x9c' bytearray(b'{\"topic\": \"/battery\", \"value\": 98.0}') {b'\\xe4\\xb3#\\xb5r\\x9c': [-20, 68775110]}\nb'\\xe4\\xb3#\\xb5r\\x9c' bytearray(b'{\"topic\": \"/battery\", \"value\": 98.0}') {b'\\xe4\\xb3#\\xb5r\\x9c': [-20, 68841222]}\nb'\\xe4\\xb3#\\xb5r\\x9c' bytearray(b'{\"topic\": \"/battery\", \"value\": 98.0}') {b'\\xe4\\xb3#\\xb5r\\x9c': [-20, 68907333]}\nb'\\xe4\\xb3#\\xb5r\\x9c' bytearray(b'{\"topic\": \"/battery\", \"value\": 98.0}') {b'\\xe4\\xb3#\\xb5r\\x9c': [-20, 68973445]}\nb'\\xe4\\xb3#\\xb5r\\x9c' bytearray(b'{\"topic\": \"/battery\", \"value\": 98.0}') {b'\\xe4\\xb3#\\xb5r\\x9c': [-20, 69039556]}\nb'\\xe4\\xb3#\\xb5r\\x9c' bytearray(b'{\"topic\": \"/battery\", \"value\": 98.0}') {b'\\xe4\\xb3#\\xb5r\\x9c': [-20, 69105671]}\nb'\\xe4\\xb3#\\xb5r\\x9c' bytearray(b'{\"topic\": \"/battery\", \"value\": 98.0}') {b'\\xe4\\xb3#\\xb5r\\x9c': [-20, 69171781]}\nb'\\xe4\\xb3#\\xb5r\\x9c' bytearray(b'{\"topic\": \"/battery\", \"value\": 98.0}') {b'\\xe4\\xb3#\\xb5r\\x9c': [-20, 69237890]}\nb'\\xe4\\xb3#\\xb5r\\x9c' bytearray(b'{\"topic\": \"/battery\", \"value\": 98.0}') {b'\\xe4\\xb3#\\xb5r\\x9c': [-20, 69304001]}\nb'\\xe4\\xb3#\\xb5r\\x9c' bytearray(b'{\"topic\": \"/battery\", \"value\": 98.0}') {b'\\xe4\\xb3#\\xb5r\\x9c': [-21, 69370115]}\nb'\\xe4\\xb3#\\xb5r\\x9c' bytearray(b'{\"topic\": \"/battery\", \"value\": 98.0}') {b'\\xe4\\xb3#\\xb5r\\x9c': [-20, 69436224]}\nb'\\xe4\\xb3#\\xb5r\\x9c' bytearray(b'{\"topic\": \"/battery\", \"value\": 98.0}') {b'\\xe4\\xb3#\\xb5r\\x9c': [-20, 69502335]}\nb'\\xe4\\xb3#\\xb5r\\x9c' bytearray(b'{\"topic\": \"/battery\", \"value\": 98.0}') {b'\\xe4\\xb3#\\xb5r\\x9c': [-20, 69568447]}\nb'\\xe4\\xb3#\\xb5r\\x9c' bytearray(b'{\"topic\": \"/battery\", \"value\": 98.0}') {b'\\xe4\\xb3#\\xb5r\\x9c': [-20, 69634559]}\nb'\\xe4\\xb3#\\xb5r\\x9c' bytearray(b'{\"topic\": \"/battery\", \"value\": 98.0}') {b'\\xe4\\xb3#\\xb5r\\x9c': [-20, 69700672]}\nb'\\xe4\\xb3#\\xb5r\\x9c' bytearray(b'{\"topic\": \"/battery\", \"value\": 98.0}') {b'\\xe4\\xb3#\\xb5r\\x9c': [-20, 69766781]}\nb'\\xe4\\xb3#\\xb5r\\x9c' bytearray(b'{\"topic\": \"/battery\", \"value\": 98.0}') {b'\\xe4\\xb3#\\xb5r\\x9c': [-20, 69832892]}\nb'\\xe4\\xb3#\\xb5r\\x9c' bytearray(b'{\"topic\": \"/battery\", \"value\": 98.0}') {b'\\xe4\\xb3#\\xb5r\\x9c': [-20, 69899004]}\nb'\\xe4\\xb3#\\xb5r\\x9c' bytearray(b'{\"topic\": \"/battery\", \"value\": 98.0}') {b'\\xe4\\xb3#\\xb5r\\x9c': [-21, 69965115]}\n"
  out "XY Graph 2":T1(graph)=[{"XY Graph"=[{"X"=1.0816326530612244, "Y"=3.7}, {"X"=1.13708320861678, "Y"=3.9}, {"X"=1.1554470975056688, "Y"=4.0}, {"X"=1.1738112641723355, "Y"=4.0}, {"X"=1.19217570861678, "Y"=4.0}, {"X"=1.2105398752834466, "Y"=4.0}, {"X"=1.228904319727891, "Y"=4.0}, {"X"=1.2472684863945578, "Y"=4.0}, {"X"=1.2656326530612243, "Y"=4.0}, {"X"=1.2839970975056687, "Y"=4.0}, {"X"=1.3023612641723354, "Y"=4.0}, {"X"=1.3207257086167798, "Y"=4.0}, {"X"=1.3390898752834466, "Y"=4.0}, {"X"=1.3574540419501133, "Y"=4.1}, {"X"=1.3758184863945577, "Y"=4.2}, {"X"=1.3941826530612245, "Y"=4.3}, {"X"=1.4125470975056689, "Y"=4.4}, {"X"=1.4309112641723356, "Y"=4.5}, {"X"=1.44927570861678, "Y"=4.6}, {"X"=1.4676398752834465, "Y"=4.7}, {"X"=1.4860040419501133, "Y"=4.8}, {"X"=1.5043684863945577, "Y"=5.0}, {"X"=1.5227329308390023, "Y"=5.0}, {"X"=1.5410970975056688, "Y"=5.0}, {"X"=1.5594612641723353, "Y"=5.0}, {"X"=1.57782570861678, "Y"=5.0}, {"X"=1.5961898752834465, "Y"=5.0}, {"X"=1.614554597505669, "Y"=5.0}, {"X"=1.63291820861678, "Y"=5.0}, {"X"=1.6512834863945578, "Y"=5.0}, {"X"=1.6696473752834466, "Y"=5.0}, {"X"=1.6880112641723355, "Y"=5.0}, {"X"=1.7063754308390022, "Y"=5.0}, {"X"=1.7247395975056687, "Y"=5.0}, {"X"=1.7431040419501134, "Y"=5.0}, {"X"=1.7614682086167799, "Y"=5.0}, {"X"=1.8165612641723357, "Y"=5.0}, {"X"=1.8621659863945577, "Y"=5.0}, {"X"=1.880529319727891, "Y"=5.0}, {"X"=1.8988934863945577, "Y"=5.1}, {"X"=1.9172576530612244, "Y"=5.2}, {"X"=1.935621819727891, "Y"=5.3}, {"X"=1.9539876530612243, "Y"=5.4}, {"X"=1.9723504308390023, "Y"=5.5}, {"X"=1.990714597505669, "Y"=5.6}, {"X"=2.0090790419501134, "Y"=5.7}, {"X"=2.0274432086167797, "Y"=5.8}, {"X"=2.04580820861678, "Y"=6.0}, {"X"=2.064174041950113, "Y"=6.0}, {"X"=2.082539319727891, "Y"=6.0}, {"X"=2.1009032086167796, "Y"=6.0}, {"X"=2.1192673752834468, "Y"=6.1}, {"X"=2.137632375283447, "Y"=6.2}, {"X"=2.155995986394558, "Y"=6.3}, {"X"=2.174360153061224, "Y"=6.4}, {"X"=2.1927245975056686, "Y"=6.6}, {"X"=2.2110887641723354, "Y"=6.7}, {"X"=2.22945320861678, "Y"=6.8}, {"X"=2.2478187641723357, "Y"=7.0}, {"X"=2.2661848752834466, "Y"=7.1}, {"X"=2.2845515419501132, "Y"=7.3}, {"X"=2.3029184863945575, "Y"=7.4}, {"X"=2.3212826530612243, "Y"=7.6}, {"X"=2.3396470975056687, "Y"=7.8}, {"X"=2.358011264172335, "Y"=7.9}, {"X"=2.3763765419501133, "Y"=8.2}, {"X"=2.3947398752834466, "Y"=8.4}, {"X"=2.4131040419501133, "Y"=8.6}, {"X"=2.4314684863945577, "Y"=8.8}, {"X"=2.449832930839002, "Y"=9.1}, {"X"=2.468197097505669, "Y"=9.3}, {"X"=2.4865612641723356, "Y"=9.6}, {"X"=2.5049273752834464, "Y"=9.8}, {"X"=2.5232926530612243, "Y"=10.1}, {"X"=2.5416568197278915, "Y"=10.4}, {"X"=2.560021541950113, "Y"=10.7}, {"X"=2.5783854308390026, "Y"=11.0}, {"X"=2.5967498752834466, "Y"=11.4}, {"X"=2.6151140419501133, "Y"=11.7}, {"X"=2.63347820861678, "Y"=12.0}, {"X"=2.6518426530612245, "Y"=12.4}, {"X"=2.670206819727891, "Y"=12.7}, {"X"=2.6885709863945575, "Y"=13.1}, {"X"=2.7069354308390023, "Y"=13.5}, {"X"=2.7252995975056686, "Y"=13.9}, {"X"=2.7436640419501135, "Y"=14.2}, {"X"=2.7803923752834465, "Y"=14.6}, {"X"=2.798756819727891, "Y"=15.5}, {"X"=2.8722137641723355, "Y"=15.9}, {"X"=2.89057820861678, "Y"=17.6}, {"X"=2.9089423752834467, "Y"=18.1}, {"X"=2.9273068197278906, "Y"=18.6}, {"X"=2.9456712641723355, "Y"=19.0}, {"X"=2.9640351530612246, "Y"=19.5}, {"X"=2.982399597505669, "Y"=20.0}, {"X"=3.0007637641723353, "Y"=20.4}, {"X"=3.0191279308390024, "Y"=20.9}, {"X"=3.037493486394558, "Y"=21.4}, {"X"=3.0558565419501136, "Y"=21.9}, {"X"=3.0742209863945575, "Y"=22.4}, {"X"=3.0925854308390024, "Y"=22.9}, {"X"=3.1109498752834464, "Y"=23.5}, {"X"=3.129313764172336, "Y"=24.0}, {"X"=3.1476826530612243, "Y"=24.5}, {"X"=3.1660476530612245, "Y"=25.1}, {"X"=3.1844120975056693, "Y"=25.7}, {"X"=3.2027765419501133, "Y"=26.2}, {"X"=3.2211407086167796, "Y"=26.8}, {"X"=3.2395048752834468, "Y"=27.4}, {"X"=3.257869041950113, "Y"=28.0}, {"X"=3.276233486394558, "Y"=28.6}, {"X"=3.294597653061224, "Y"=29.2}, {"X"=3.312962097505668, "Y"=29.8}, {"X"=3.3313262641723353, "Y"=30.4}, {"X"=3.3496904308390016, "Y"=31.1}, {"X"=3.368055153061224, "Y"=31.7}, {"X"=3.386419041950113, "Y"=32.3}, {"X"=3.4047834863945585, "Y"=33.0}, {"X"=3.423147653061224, "Y"=33.7}, {"X"=3.441511819727891, "Y"=34.3}, {"X"=3.459876264172335, "Y"=35.0}, {"X"=3.47824070861678, "Y"=35.7}, {"X"=3.496604875283447, "Y"=36.4}, {"X"=3.5149690419501134, "Y"=37.1}, {"X"=3.5333334863945574, "Y"=37.8}, {"X"=3.5516976530612245, "Y"=38.5}, {"X"=3.570061819727891, "Y"=39.2}, {"X"=3.5884262641723357, "Y"=39.9}, {"X"=3.606790430839002, "Y"=40.6}, {"X"=3.625155430839002, "Y"=41.4}, {"X"=3.643519041950113, "Y"=42.1}, {"X"=3.6618840419501133, "Y"=42.8}, {"X"=3.955711541950113, "Y"=54.4}, {"X"=3.974075986394558, "Y"=55.1}, {"X"=3.992440430839002, "Y"=55.8}, {"X"=4.010804597505668, "Y"=56.5}, {"X"=4.0291687641723355, "Y"=57.2}, {"X"=4.047532930839002, "Y"=57.9}, {"X"=4.065897375283447, "Y"=58.6}, {"X"=4.084261541950113, "Y"=59.3}, {"X"=4.10262570861678, "Y"=60.0}, {"X"=4.120990153061224, "Y"=60.7}, {"X"=4.139355153061224, "Y"=61.3}, {"X"=4.157719597505669, "Y"=62.0}, {"X"=4.176082930839002, "Y"=62.8}, {"X"=4.194447097505669, "Y"=63.5}, {"X"=4.2128115419501135, "Y"=64.2}, {"X"=4.23117570861678, "Y"=64.9}, {"X"=4.249540430839002, "Y"=65.6}, {"X"=4.267904319727891, "Y"=66.3}, {"X"=4.286268764172336, "Y"=67.0}, {"X"=4.30463320861678, "Y"=67.7}, {"X"=4.322997097505668, "Y"=68.4}, {"X"=4.341361541950113, "Y"=69.1}, {"X"=4.35972570861678, "Y"=69.8}, {"X"=4.378089875283447, "Y"=70.5}, {"X"=4.396454319727891, "Y"=71.1}, {"X"=4.414818486394557, "Y"=71.8}, {"X"=4.433182930839002, "Y"=72.5}, {"X"=4.451547653061224, "Y"=73.1}, {"X"=4.469911264172335, "Y"=73.8}, {"X"=4.48827570861678, "Y"=74.4}, {"X"=4.506640153061224, "Y"=75.0}, {"X"=4.525004319727891, "Y"=75.6}, {"X"=4.543369041950113, "Y"=76.2}, {"X"=4.561732653061225, "Y"=76.8}, {"X"=4.580097653061225, "Y"=77.4}, {"X"=4.598461264172335, "Y"=78.0}, {"X"=4.61682570861678, "Y"=78.6}, {"X"=4.635189875283447, "Y"=79.1}, {"X"=4.653554041950113, "Y"=79.7}, {"X"=4.671918486394558, "Y"=80.3}, {"X"=4.6902834863945575, "Y"=80.8}, {"X"=4.708647375283447, "Y"=81.4}, {"X"=4.727011819727891, "Y"=81.9}, {"X"=4.745375430839002, "Y"=82.5}, {"X"=4.763739875283447, "Y"=83.0}, {"X"=4.782104597505669, "Y"=83.6}, {"X"=4.800468486394557, "Y"=84.1}, {"X"=4.8188332086167796, "Y"=84.6}, {"X"=4.837196819727891, "Y"=85.2}, {"X"=4.855561264172335, "Y"=85.7}, {"X"=4.873925708616779, "Y"=86.2}, {"X"=4.892289597505669, "Y"=86.7}, {"X"=4.910655986394557, "Y"=87.3}, {"X"=4.929021541950113, "Y"=87.8}, {"X"=4.947385430839002, "Y"=88.3}, {"X"=4.965749875283446, "Y"=88.9}, {"X"=4.984113764172336, "Y"=89.4}, {"X"=5.002478764172335, "Y"=90.0}, {"X"=5.020842375283447, "Y"=90.5}, {"X"=5.039206819727891, "Y"=91.0}, {"X"=5.057570986394558, "Y"=91.4}, {"X"=5.075935430839002, "Y"=91.9}, {"X"=5.094300153061225, "Y"=92.3}, {"X"=5.112664319727891, "Y"=92.7}, {"X"=5.13102820861678, "Y"=93.1}, {"X"=5.149392375283447, "Y"=93.5}, {"X"=5.167756541950114, "Y"=93.9}, {"X"=5.186121541950113, "Y"=94.3}, {"X"=5.204485430839003, "Y"=94.6}, {"X"=5.222849319727891, "Y"=94.9}, {"X"=5.241213764172336, "Y"=95.2}, {"X"=5.2595779308390025, "Y"=95.5}, {"X"=5.2779423752834465, "Y"=95.8}, {"X"=5.296316819727891, "Y"=96.1}, {"X"=5.314682930839002, "Y"=96.3}, {"X"=5.351410430839002, "Y"=96.5}, {"X"=5.369774875283446, "Y"=96.9}, {"X"=5.38813959750567, "Y"=97.0}, {"X"=5.406503764172336, "Y"=97.1}, {"X"=5.424867653061225, "Y"=97.3}, {"X"=5.443231819727891, "Y"=97.4}, {"X"=5.461595986394558, "Y"=97.5}, {"X"=5.479960430839002, "Y"=97.6}, {"X"=5.498324875283447, "Y"=97.8}, {"X"=5.516689041950114, "Y"=97.9}, {"X"=5.53505320861678, "Y"=98.0}, {"X"=5.553417375283447, "Y"=98.0}, {"X"=5.571781819727891, "Y"=98.0}, {"X"=5.590145986394557, "Y"=98.0}, {"X"=5.608510153061224, "Y"=98.0}, {"X"=5.626874597505669, "Y"=98.0}, {"X"=5.645239319727891, "Y"=98.0}, {"X"=5.663603208616781, "Y"=98.0}, {"X"=5.681967375283448, "Y"=98.0}, {"X"=5.700331819727891, "Y"=98.0}, {"X"=5.7186959863945575, "Y"=98.0}, {"X"=5.737060153061225, "Y"=98.0}, {"X"=5.755424319727892, "Y"=98.0}, {"X"=5.773788764172336, "Y"=98.0}, {"X"=5.792152930839002, "Y"=98.0}, {"X"=5.810517375283447, "Y"=98.0}, {"X"=5.828881541950114, "Y"=98.0}, {"X"=5.84724570861678, "Y"=98.0}, {"X"=5.865610430839002, "Y"=98.0}, {"X"=5.8839743197278915, "Y"=98.0}, {"X"=5.902338486394559, "Y"=98.0}, {"X"=5.920702930839002, "Y"=98.0}, {"X"=5.939067097505669, "Y"=98.0}, {"X"=5.957431541950114, "Y"=98.0}, {"X"=5.975795986394559, "Y"=98.0}]}, {"XY Graph"=[{"X"=0.018364722222222223, "Y"=0.2}, {"X"=0.036728611111111115, "Y"=0.2}, {"X"=0.055092777777777775, "Y"=0.7}, {"X"=0.0734575, "Y"=1.0}, {"X"=0.09182166666666666, "Y"=1.1}, {"X"=0.11018583333333333, "Y"=1.2}, {"X"=0.12855111111111112, "Y"=1.4}, {"X"=0.14691444444444446, "Y"=1.7}, {"X"=0.16527916666666667, "Y"=2.0}, {"X"=0.18364277777777777, "Y"=2.0}, {"X"=0.20200777777777776, "Y"=2.0}, {"X"=0.22037138888888888, "Y"=2.0}, {"X"=0.23873555555555553, "Y"=2.0}, {"X"=0.2571, "Y"=2.1}, {"X"=0.2754641666666667, "Y"=2.1}, {"X"=0.2938288888888889, "Y"=2.2}, {"X"=0.3305572222222223, "Y"=2.3}, {"X"=0.3489213888888889, "Y"=2.4}, {"X"=0.4223783333333333, "Y"=2.8}, {"X"=0.4407433333333333, "Y"=2.8}, {"X"=0.4591088888888889, "Y"=2.9}, {"X"=0.47747472222222226, "Y"=2.9}, {"X"=0.4958383333333333, "Y"=2.9}, {"X"=0.5142025, "Y"=3.0}, {"X"=0.6060244444444444, "Y"=3.0}, {"X"=0.6243880555555557, "Y"=2.9}, {"X"=0.6427525000000001, "Y"=3.0}, {"X"=0.6611172222222221, "Y"=3.0}, {"X"=0.6794811111111111, "Y"=3.0}, {"X"=0.6978452777777778, "Y"=3.0}, {"X"=0.7162094444444445, "Y"=3.0}, {"X"=0.7345738888888889, "Y"=3.0}, {"X"=0.7529380555555556, "Y"=3.0}, {"X"=0.7713024999999999, "Y"=3.0}, {"X"=0.7896666666666667, "Y"=3.0}, {"X"=0.808031111111111, "Y"=3.0}, {"X"=0.8263952777777778, "Y"=3.0}, {"X"=0.8447600000000001, "Y"=3.1}, {"X"=0.8631238888888889, "Y"=3.1}, {"X"=0.8814886111111111, "Y"=3.2}, {"X"=0.8998524999999999, "Y"=3.3}, {"X"=0.9182166666666666, "Y"=3.5}, {"X"=0.936581388888889, "Y"=3.6}, {"X"=0.9549452777777777, "Y"=3.7}, {"X"=0.97331, "Y"=3.9}, {"X"=0.9916738888888889, "Y"=4.0}, {"X"=1.0100380555555557, "Y"=4.0}, {"X"=1.0284022222222222, "Y"=4.0}, {"X"=1.0467666666666668, "Y"=4.0}, {"X"=1.0651311111111113, "Y"=4.0}, {"X"=1.083496111111111, "Y"=4.0}, {"X"=1.1018597222222224, "Y"=4.0}, {"X"=1.120223611111111, "Y"=4.0}, {"X"=1.1385880555555556, "Y"=4.0}, {"X"=1.1569525, "Y"=4.0}, {"X"=1.175316388888889, "Y"=4.0}, {"X"=1.1936808333333333, "Y"=4.0}, {"X"=1.212045, "Y"=4.0}, {"X"=1.2304099999999998, "Y"=4.0}, {"X"=1.2487738888888888, "Y"=4.0}, {"X"=1.2855022222222223, "Y"=4.2}, {"X"=1.3038663888888888, "Y"=4.3}, {"X"=1.3222308333333332, "Y"=4.4}, {"X"=1.3956880555555555, "Y"=4.8}, {"X"=1.414052222222222, "Y"=4.9}, {"X"=1.4324172222222225, "Y"=5.0}, {"X"=1.4507808333333332, "Y"=5.0}, {"X"=1.4691455555555557, "Y"=5.0}, {"X"=1.4875091666666667, "Y"=5.0}, {"X"=1.505873611111111, "Y"=5.0}, {"X"=1.5242377777777778, "Y"=5.0}, {"X"=1.5426024999999999, "Y"=5.0}, {"X"=1.560966388888889, "Y"=5.0}, {"X"=1.5793308333333334, "Y"=5.0}, {"X"=1.597695, "Y"=5.0}, {"X"=1.6160591666666666, "Y"=5.0}, {"X"=1.6344238888888891, "Y"=5.0}, {"X"=1.6527883333333333, "Y"=5.0}, {"X"=1.6711552777777776, "Y"=5.0}, {"X"=1.6895222222222221, "Y"=5.0}, {"X"=1.7078872222222223, "Y"=5.0}, {"X"=1.7262516666666667, "Y"=5.0}, {"X"=1.7446147222222224, "Y"=5.0}, {"X"=1.7629788888888889, "Y"=5.0}, {"X"=1.7813433333333333, "Y"=5.0}, {"X"=1.7997075, "Y"=5.0}, {"X"=1.8180719444444444, "Y"=5.0}, {"X"=1.8364361111111112, "Y"=5.0}, {"X"=1.8548002777777777, "Y"=5.1}, {"X"=1.873165, "Y"=5.2}, {"X"=1.8915288888888888, "Y"=5.2}, {"X"=1.9098933333333332, "Y"=5.3}, {"X"=1.9282575, "Y"=5.4}, {"X"=1.9466216666666665, "Y"=5.5}, {"X"=1.964986388888889, "Y"=5.6}, {"X"=1.9833502777777776, "Y"=5.8}, {"X"=2.001714444444444, "Y"=5.9}, {"X"=2.0200788888888885, "Y"=6.0}, {"X"=2.038443333333333, "Y"=6.0}, {"X"=2.0568074999999997, "Y"=6.0}, {"X"=2.0751719444444445, "Y"=6.1}, {"X"=2.093536388888889, "Y"=6.2}, {"X"=2.1119002777777776, "Y"=6.3}, {"X"=2.1302644444444443, "Y"=6.4}, {"X"=2.1486288888888887, "Y"=6.5}, {"X"=2.166993888888889, "Y"=6.6}, {"X"=2.185357222222222, "Y"=6.7}, {"X"=2.2037216666666666, "Y"=6.9}, {"X"=2.2220858333333333, "Y"=7.0}, {"X"=2.2404505555555554, "Y"=7.2}, {"X"=2.2588155555555556, "Y"=7.3}, {"X"=2.277178611111111, "Y"=7.4}, {"X"=2.2955430555555556, "Y"=7.6}, {"X"=2.3139072222222223, "Y"=7.8}, {"X"=2.3322716666666663, "Y"=8.0}, {"X"=2.3506361111111116, "Y"=8.2}, {"X"=2.3689999999999998, "Y"=8.4}, {"X"=2.3873644444444446, "Y"=8.6}, {"X"=2.405728611111111, "Y"=8.9}, {"X"=2.4240930555555553, "Y"=9.1}, {"X"=2.442457222222222, "Y"=9.3}, {"X"=2.460821666666667, "Y"=9.6}, {"X"=2.479185833333333, "Y"=9.8}, {"X"=2.49755, "Y"=10.1}, {"X"=2.515914444444444, "Y"=10.4}, {"X"=2.534278888888889, "Y"=10.7}, {"X"=2.5526433333333336, "Y"=11.0}, {"X"=2.6628294444444447, "Y"=13.0}, {"X"=2.681193888888889, "Y"=13.4}, {"X"=2.699557222222223, "Y"=13.7}, {"X"=2.7179213888888887, "Y"=14.1}, {"X"=2.7362855555555554, "Y"=14.5}, {"X"=2.773014166666667, "Y"=15.3}, {"X"=2.7913802777777774, "Y"=15.7}, {"X"=2.8097455555555557, "Y"=16.1}, {"X"=2.828109722222222, "Y"=16.5}, {"X"=2.846474444444445, "Y"=17.0}, {"X"=2.864838333333333, "Y"=17.4}, {"X"=2.883202777777778, "Y"=17.8}, {"X"=2.9015669444444443, "Y"=18.3}, {"X"=2.919931111111111, "Y"=18.7}, {"X"=2.9382958333333336, "Y"=19.2}, {"X"=2.956660277777778, "Y"=19.6}, {"X"=2.9750241666666666, "Y"=20.1}, {"X"=2.9933883333333338, "Y"=20.6}, {"X"=3.0117524999999996, "Y"=21.0}, {"X"=3.0301169444444445, "Y"=21.5}, {"X"=3.0484816666666665, "Y"=22.0}, {"X"=3.0668455555555556, "Y"=22.5}, {"X"=3.0852097222222223, "Y"=23.0}, {"X"=3.1035741666666667, "Y"=23.5}, {"X"=3.121938333333333, "Y"=24.1}, {"X"=3.140302777777778, "Y"=24.6}, {"X"=3.158666944444444, "Y"=25.2}, {"X"=3.177031388888889, "Y"=25.7}, {"X"=3.1953955555555558, "Y"=26.3}, {"X"=3.213759722222222, "Y"=26.8}, {"X"=3.232123888888889, "Y"=27.4}, {"X"=3.2504899999999997, "Y"=28.0}, {"X"=3.268855555555555, "Y"=28.6}, {"X"=3.2872194444444447, "Y"=29.2}, {"X"=3.305583888888889, "Y"=29.8}, {"X"=3.3239480555555554, "Y"=30.4}, {"X"=3.3423125000000002, "Y"=31.0}, {"X"=3.3606780555555558, "Y"=31.7}, {"X"=3.3790408333333337, "Y"=32.3}, {"X"=3.397405555555556, "Y"=33.0}, {"X"=3.4157697222222225, "Y"=33.6}, {"X"=3.4341341666666665, "Y"=34.3}, {"X"=3.4524983333333332, "Y"=35.0}, {"X"=3.4708630555555553, "Y"=35.6}, {"X"=3.4892280555555555, "Y"=36.3}, {"X"=3.507592777777778, "Y"=37.0}, {"X"=3.5259577777777777, "Y"=37.7}, {"X"=3.5443225, "Y"=38.4}, {"X"=3.5626863888888893, "Y"=39.1}, {"X"=3.5810508333333333, "Y"=39.8}, {"X"=3.599415, "Y"=40.5}, {"X"=3.6177791666666663, "Y"=41.3}, {"X"=3.636143611111111, "Y"=42.0}, {"X"=3.654507777777778, "Y"=42.7}, {"X"=3.6728722222222223, "Y"=43.4}, {"X"=3.6912363888888886, "Y"=44.2}, {"X"=3.709601111111111, "Y"=44.9}, {"X"=3.727965, "Y"=45.6}, {"X"=3.746329166666667, "Y"=46.3}, {"X"=3.7646936111111113, "Y"=47.0}, {"X"=3.7830577777777776, "Y"=47.7}, {"X"=3.8014222222222225, "Y"=48.5}, {"X"=3.8197863888888888, "Y"=49.2}, {"X"=3.838150555555556, "Y"=49.9}, {"X"=3.856515, "Y"=50.6}, {"X"=3.8748794444444448, "Y"=51.3}, {"X"=3.893243611111111, "Y"=52.0}, {"X"=3.911607777777778, "Y"=52.7}, {"X"=3.9299719444444445, "Y"=53.4}, {"X"=3.948336388888889, "Y"=54.1}, {"X"=3.9667005555555552, "Y"=54.8}, {"X"=3.9850661111111108, "Y"=55.5}, {"X"=4.003429166666667, "Y"=56.2}, {"X"=4.021793333333333, "Y"=56.9}, {"X"=4.040157777777777, "Y"=57.6}, {"X"=4.0585225000000005, "Y"=58.3}, {"X"=4.076886944444444, "Y"=59.0}, {"X"=4.095250555555555, "Y"=59.6}, {"X"=4.113614999999999, "Y"=60.3}, {"X"=4.1319791666666665, "Y"=61.0}, {"X"=4.1503436111111105, "Y"=61.7}, {"X"=4.168707777777778, "Y"=62.4}, {"X"=4.187071944444445, "Y"=63.1}, {"X"=4.2054366666666665, "Y"=63.8}, {"X"=4.223800555555555, "Y"=64.5}, {"X"=4.242164722222222, "Y"=65.2}, {"X"=4.260528888888889, "Y"=65.9}, {"X"=4.2788933333333325, "Y"=66.5}, {"X"=4.29725861111111, "Y"=67.2}, {"X"=4.315622222222222, "Y"=67.9}, {"X"=4.333986111111112, "Y"=68.6}, {"X"=4.370715000000001, "Y"=70.0}, {"X"=4.389080000000001, "Y"=70.7}, {"X"=4.407443611111111, "Y"=71.4}, {"X"=4.4258075, "Y"=72.0}, {"X"=4.444171944444445, "Y"=72.7}, {"X"=4.462536111111111, "Y"=73.3}, {"X"=4.480900555555555, "Y"=74.0}, {"X"=4.499265555555556, "Y"=74.6}, {"X"=4.517628888888889, "Y"=75.2}, {"X"=4.664543055555556, "Y"=79.9}, {"X"=4.6829075, "Y"=80.4}, {"X"=4.701271944444445, "Y"=81.0}, {"X"=4.738000277777777, "Y"=82.1}, {"X"=4.756365000000001, "Y"=82.6}, {"X"=4.774728888888889, "Y"=83.1}, {"X"=4.7930930555555555, "Y"=83.7}, {"X"=4.8114575, "Y"=84.2}, {"X"=4.829822222222222, "Y"=84.7}, {"X"=4.848185833333334, "Y"=85.2}, {"X"=4.866550277777777, "Y"=85.8}, {"X"=4.884914444444444, "Y"=86.3}, {"X"=4.90327861111111, "Y"=86.8}, {"X"=4.921643333333334, "Y"=87.3}, {"X"=4.940007222222222, "Y"=87.9}, {"X"=4.958371666666666, "Y"=88.4}, {"X"=4.976735833333334, "Y"=88.9}, {"X"=4.9951, "Y"=89.5}, {"X"=5.013464444444446, "Y"=90.0}, {"X"=5.031828611111111, "Y"=90.5}, {"X"=5.050193055555555, "Y"=91.0}, {"X"=5.068557222222222, "Y"=91.4}, {"X"=5.0869213888888885, "Y"=91.9}, {"X"=5.105286944444444, "Y"=92.3}, {"X"=5.12365, "Y"=92.8}, {"X"=5.142014444444444, "Y"=93.2}, {"X"=5.160378611111112, "Y"=93.5}, {"X"=5.178742777777777, "Y"=93.9}, {"X"=5.197107222222223, "Y"=94.3}, {"X"=5.215471388888889, "Y"=94.6}, {"X"=5.233836388888889, "Y"=94.9}, {"X"=5.252199999999999, "Y"=95.3}, {"X"=5.270564166666666, "Y"=95.6}, {"X"=5.288928611111111, "Y"=95.9}, {"X"=5.307292777777778, "Y"=96.1}, {"X"=5.325656944444445, "Y"=96.3}, {"X"=5.344021388888889, "Y"=96.5}, {"X"=5.362385555555556, "Y"=96.7}, {"X"=5.380750000000001, "Y"=96.9}, {"X"=5.399114166666667, "Y"=97.0}, {"X"=5.41747861111111, "Y"=97.1}, {"X"=5.435842777777777, "Y"=97.3}, {"X"=5.4542075, "Y"=97.4}, {"X"=5.472571388888889, "Y"=97.5}, {"X"=5.490935555555555, "Y"=97.6}, {"X"=5.509299722222222, "Y"=97.7}, {"X"=5.527664166666667, "Y"=97.8}, {"X"=5.546028333333334, "Y"=98.0}, {"X"=5.564392499999999, "Y"=98.0}, {"X"=5.582757222222223, "Y"=98.0}, {"X"=5.601121111111111, "Y"=98.0}, {"X"=5.619485555555556, "Y"=98.0}, {"X"=5.637849722222222, "Y"=98.0}, {"X"=5.6562141666666665, "Y"=98.0}, {"X"=5.674578333333333, "Y"=98.0}, {"X"=5.692943611111111, "Y"=98.0}, {"X"=5.7113075, "Y"=98.0}, {"X"=5.729671111111111, "Y"=98.0}, {"X"=5.7480352777777775, "Y"=98.0}, {"X"=5.766400277777778, "Y"=98.0}, {"X"=5.7847638888888895, "Y"=98.0}, {"X"=5.803128055555556, "Y"=98.0}, {"X"=5.821492500000001, "Y"=98.0}, {"X"=5.839856944444445, "Y"=98.0}, {"X"=5.858221666666667, "Y"=98.0}, {"X"=5.876585277777777, "Y"=98.0}, {"X"=5.894949444444444, "Y"=98.0}, {"X"=5.913313888888889, "Y"=98.0}]}]
  in  "charging 1":string="1  b'\\xe4\\xb3#\\xb5r\\x9c' bytearray(b'{\"topic\": \"/battery\", \"value\": 3.7}') {b'\\xe4\\xb3#\\xb5r\\x9c': [-19, 133509]}\n1  b'\\xe4\\xb3#\\xb5r\\x9c' bytearray(b'{\"topic\": \"/battery\", \"value\": 3.9}') {b'\\xe4\\xb3#\\xb5r\\x9c': [-19, 199622]}\n1  b'\\xe4\\xb3#\\xb5r\\x9c' bytearray(b'{\"topic\": \"/battery\", \"value\": 4.0}') {b'\\xe4\\xb3#\\xb5r\\x9c': [-21, 265732]}\n1  b'\\xe4\\xb3#\\xb5r\\x9c' bytearray(b'{\"topic\": \"/battery\", \"value\": 4.0}') {b'\\xe4\\xb3#\\xb5r\\x9c': [-20, 331843]}\n1  b'\\xe4\\xb3#\\xb5r\\x9c' bytearray(b'{\"topic\": \"/battery\", \"value\": 4.0}') {b'\\xe4\\xb3#\\xb5r\\x9c': [-21, 397955]}\n1  b'\\xe4\\xb3#\\xb5r\\x9c' bytearray(b'{\"topic\": \"/battery\", \"value\": 4.0}') {b'\\xe4\\xb3#\\xb5r\\x9c': [-23, 464066]}\n1  b'\\xe4\\xb3#\\xb5r\\x9c' bytearray(b'{\"topic\": \"/battery\", \"value\": 4.0}') {b'\\xe4\\xb3#\\xb5r\\x9c': [-21, 530178]}\n1  b'\\xe4\\xb3#\\xb5r\\x9c' bytearray(b'{\"topic\": \"/battery\", \"value\": 4.0}') {b'\\xe4\\xb3#\\xb5r\\x9c': [-21, 596289]}\n1  b'\\xe4\\xb3#\\xb5r\\x9c' bytearray(b'{\"topic\": \"/battery\", \"value\": 4.0}') {b'\\xe4\\xb3#\\xb5r\\x9c': [-22, 662400]}\n1  b'\\xe4\\xb3#\\xb5r\\x9c' bytearray(b'{\"topic\": \"/battery\", \"value\": 4.0}') {b'\\xe4\\xb3#\\xb5r\\x9c': [-22, 728512]}\n1  b'\\xe4\\xb3#\\xb5r\\x9c' bytearray(b'{\"topic\": \"/battery\", \"value\": 4.0}') {b'\\xe4\\xb3#\\xb5r\\x9c': [-24, 794623]}\n1  b'\\xe4\\xb3#\\xb5r\\x9c' bytearray(b'{\"topic\": \"/battery\", \"value\": 4.0}') {b'\\xe4\\xb3#\\xb5r\\x9c': [-19, 860735]}\n1  b'\\xe4\\xb3#\\xb5r\\x9c' bytearray(b'{\"topic\": \"/battery\", \"value\": 4.0}') {b'\\xe4\\xb3#\\xb5r\\x9c': [-28, 926846]}\n1  b'\\xe4\\xb3#\\xb5r\\x9c' bytearray(b'{\"topic\": \"/battery\", \"value\": 4.1}') {b'\\xe4\\xb3#\\xb5r\\x9c': [-26, 992957]}\n1  b'\\xe4\\xb3#\\xb5r\\x9c' bytearray(b'{\"topic\": \"/battery\", \"value\": 4.2}') {b'\\xe4\\xb3#\\xb5r\\x9c': [-23, 1059069]}\n1  b'\\xe4\\xb3#\\xb5r\\x9c' bytearray(b'{\"topic\": \"/battery\", \"value\": 4.3}') {b'\\xe4\\xb3#\\xb5r\\x9c': [-27, 1125180]}\n1  b'\\xe4\\xb3#\\xb5r\\x9c' bytearray(b'{\"topic\": \"/battery\", \"value\": 4.4}') {b'\\xe4\\xb3#\\xb5r\\x9c': [-24, 1191292]}\n1  b'\\xe4\\xb3#\\xb5r\\x9c' bytearray(b'{\"topic\": \"/battery\", \"value\": 4.5}') {b'\\xe4\\xb3#\\xb5r\\x9c': [-26, 1257403]}\n1  b'\\xe4\\xb3#\\xb5r\\x9c' bytearray(b'{\"topic\": \"/battery\", \"value\": 4.6}') {b'\\xe4\\xb3#\\xb5r\\x9c': [-29, 1323515]}\n1  b'\\xe4\\xb3#\\xb5r\\x9c' bytearray(b'{\"topic\": \"/battery\", \"value\": 4.7}') {b'\\xe4\\xb3#\\xb5r\\x9c': [-23, 1389626]}\n1  b'\\xe4\\xb3#\\xb5r\\x9c' bytearray(b'{\"topic\": \"/battery\", \"value\": 4.8}') {b'\\xe4\\xb3#\\xb5r\\x9c': [-24, 1455737]}\n1  b'\\xe4\\xb3#\\xb5r\\x9c' bytearray(b'{\"topic\": \"/battery\", \"value\": 5.0}') {b'\\xe4\\xb3#\\xb5r\\x9c': [-24, 1521849]}\n1  b'\\xe4\\xb3#\\xb5r\\x9c' bytearray(b'{\"topic\": \"/battery\", \"value\": 5.0}') {b'\\xe4\\xb3#\\xb5r\\x9c': [-27, 1587961]}\n1  b'\\xe4\\xb3#\\xb5r\\x9c' bytearray(b'{\"topic\": \"/battery\", \"value\": 5.0}') {b'\\xe4\\xb3#\\xb5r\\x9c': [-23, 1654072]}\n1  b'\\xe4\\xb3#\\xb5r\\x9c' bytearray(b'{\"topic\": \"/battery\", \"value\": 5.0}') {b'\\xe4\\xb3#\\xb5r\\x9c': [-24, 1720183]}\n1  b'\\xe4\\xb3#\\xb5r\\x9c' bytearray(b'{\"topic\": \"/battery\", \"value\": 5.0}') {b'\\xe4\\xb3#\\xb5r\\x9c': [-23, 1786295]}\n1  b'\\xe4\\xb3#\\xb5r\\x9c' bytearray(b'{\"topic\": \"/battery\", \"value\": 5.0}') {b'\\xe4\\xb3#\\xb5r\\x9c': [-25, 1852406]}\n1  b'\\xe4\\xb3#\\xb5r\\x9c' bytearray(b'{\"topic\": \"/battery\", \"value\": 5.0}') {b'\\xe4\\xb3#\\xb5r\\x9c': [-25, 1918519]}\n1  b'\\xe4\\xb3#\\xb5r\\x9c' bytearray(b'{\"topic\": \"/battery\", \"value\": 5.0}') {b'\\xe4\\xb3#\\xb5r\\x9c': [-31, 1984628]}\n1  b'\\xe4\\xb3#\\xb5r\\x9c' bytearray(b'{\"topic\": \"/battery\", \"value\": 5.0}') {b'\\xe4\\xb3#\\xb5r\\x9c': [-27, 2050743]}\n1  b'\\xe4\\xb3#\\xb5r\\x9c' bytearray(b'{\"topic\": \"/battery\", \"value\": 5.0}') {b'\\xe4\\xb3#\\xb5r\\x9c': [-28, 2116853]}\n1  b'\\xe4\\xb3#\\xb5r\\x9c' bytearray(b'{\"topic\": \"/battery\", \"value\": 5.0}') {b'\\xe4\\xb3#\\xb5r\\x9c': [-29, 2182963]}\n1  b'\\xe4\\xb3#\\xb5r\\x9c' bytearray(b'{\"topic\": \"/battery\", \"value\": 5.0}') {b'\\xe4\\xb3#\\xb5r\\x9c': [-29, 2249074]}\n1  b'\\xe4\\xb3#\\xb5r\\x9c' bytearray(b'{\"topic\": \"/battery\", \"value\": 5.0}') {b'\\xe4\\xb3#\\xb5r\\x9c': [-21, 2315185]}\n1  b'\\xe4\\xb3#\\xb5r\\x9c' bytearray(b'{\"topic\": \"/battery\", \"value\": 5.0}') {b'\\xe4\\xb3#\\xb5r\\x9c': [-14, 2381297]}\n1  b'\\xe4\\xb3#\\xb5r\\x9c' bytearray(b'{\"topic\": \"/battery\", \"value\": 5.0}') {b'\\xe4\\xb3#\\xb5r\\x9c': [-14, 2447408]}\n1  b’\\xe4\\xb3#\\xb\n b'\\xe4\\xb3#\\xb5r\\x9c' bytearray(b'{\"topic\": \"/battery\", \"value\": 5.0}') {b'\\xe4\\xb3#\\xb5r\\x9c': [-15, 2645743]}\nb'\\xe4\\xb3#\\xb5r\\x9c' bytearray(b'{\"topic\": \"/battery\", \"value\": 5.0}') {b'\\xe4\\xb3#\\xb5r\\x9c': [-22, 2809920], b'd\\xe83\\x86\\x8e\\xc8': [-30, 2747079]}\n1  b'\\xe4\\xb3#\\xb5r\\x9c' bytearray(b'{\"topic\": \"/battery\", \"value\": 5.0}') {b'\\xe4\\xb3#\\xb5r\\x9c': [-23, 2876028], b'd\\xe83\\x86\\x8e\\xc8': [-30, 2747079]}\n1  b'\\xe4\\xb3#\\xb5r\\x9c' bytearray(b'{\"topic\": \"/battery\", \"value\": 5.1}') {b'\\xe4\\xb3#\\xb5r\\x9c': [-26, 2942139], b'd\\xe83\\x86\\x8e\\xc8': [-30, 2747079]}\n1  b'\\xe4\\xb3#\\xb5r\\x9c' bytearray(b'{\"topic\": \"/battery\", \"value\": 5.2}') {b'\\xe4\\xb3#\\xb5r\\x9c': [-23, 3008250], b'd\\xe83\\x86\\x8e\\xc8': [-30, 2747079]}\n1  b'\\xe4\\xb3#\\xb5r\\x9c' bytearray(b'{\"topic\": \"/battery\", \"value\": 5.3}') {b'\\xe4\\xb3#\\xb5r\\x9c': [-24, 3074361], b'd\\xe83\\x86\\x8e\\xc8': [-30, 2747079]}\n1  b'\\xe4\\xb3#\\xb5r\\x9c' bytearray(b'{\"topic\": \"/battery\", \"value\": 5.4}') {b'\\xe4\\xb3#\\xb5r\\x9c': [-25, 3140478], b'd\\xe83\\x86\\x8e\\xc8': [-30, 2747079]}\n1  b'\\xe4\\xb3#\\xb5r\\x9c' bytearray(b'{\"topic\": \"/battery\", \"value\": 5.5}') {b'\\xe4\\xb3#\\xb5r\\x9c': [-23, 3206584], b'd\\xe83\\x86\\x8e\\xc8': [-30, 2747079]}\n1  b'\\xe4\\xb3#\\xb5r\\x9c' bytearray(b'{\"topic\": \"/battery\", \"value\": 5.6}') {b'\\xe4\\xb3#\\xb5r\\x9c': [-24, 3272695], b'd\\xe83\\x86\\x8e\\xc8': [-30, 2747079]}\n1  b'\\xe4\\xb3#\\xb5r\\x9c' bytearray(b'{\"topic\": \"/battery\", \"value\": 5.7}') {b'\\xe4\\xb3#\\xb5r\\x9c': [-23, 3338807], b'd\\xe83\\x86\\x8e\\xc8': [-30, 2747079]}\n1  b'\\xe4\\xb3#\\xb5r\\x9c' bytearray(b'{\"topic\": \"/battery\", \"value\": 5.8}') {b'\\xe4\\xb3#\\xb5r\\x9c': [-25, 3404918], b'd\\xe83\\x86\\x8e\\xc8': [-30, 2747079]}\n1  b'\\xe4\\xb3#\\xb5r\\x9c' bytearray(b'{\"topic\": \"/battery\", \"value\": 6.0}') {b'\\xe4\\xb3#\\xb5r\\x9c': [-26, 3471032], b'd\\xe83\\x86\\x8e\\xc8': [-30, 2747079]}\n1  b'\\xe4\\xb3#\\xb5r\\x9c' bytearray(b'{\"topic\": \"/battery\", \"value\": 6.0}') {b'\\xe4\\xb3#\\xb5r\\x9c': [-24, 3537149], b'd\\xe83\\x86\\x8e\\xc8': [-30, 2747079]}\n1  b'\\xe4\\xb3#\\xb5r\\x9c' bytearray(b'{\"topic\": \"/battery\", \"value\": 6.0}') {b'\\xe4\\xb3#\\xb5r\\x9c': [-25, 3603264], b'd\\xe83\\x86\\x8e\\xc8': [-30, 2747079]}\n1  b'\\xe4\\xb3#\\xb5r\\x9c' bytearray(b'{\"topic\": \"/battery\", \"value\": 6.0}') {b'\\xe4\\xb3#\\xb5r\\x9c': [-25, 3669374], b'd\\xe83\\x86\\x8e\\xc8': [-30, 2747079]}\n1  b'\\xe4\\xb3#\\xb5r\\x9c' bytearray(b'{\"topic\": \"/battery\", \"value\": 6.1}') {b'\\xe4\\xb3#\\xb5r\\x9c': [-22, 3735485], b'd\\xe83\\x86\\x8e\\xc8': [-30, 2747079]}\n1  b'\\xe4\\xb3#\\xb5r\\x9c' bytearray(b'{\"topic\": \"/battery\", \"value\": 6.2}') {b'\\xe4\\xb3#\\xb5r\\x9c': [-24, 3801599], b'd\\xe83\\x86\\x8e\\xc8': [-30, 2747079]}\n1  b'\\xe4\\xb3#\\xb5r\\x9c' bytearray(b'{\"topic\": \"/battery\", \"value\": 6.3}') {b'\\xe4\\xb3#\\xb5r\\x9c': [-28, 3867708], b'd\\xe83\\x86\\x8e\\xc8': [-30, 2747079]}\n1  b'\\xe4\\xb3#\\xb5r\\x9c' bytearray(b'{\"topic\": \"/battery\", \"value\": 6.4}') {b'\\xe4\\xb3#\\xb5r\\x9c': [-23, 3933819], b'd\\xe83\\x86\\x8e\\xc8': [-30, 2747079]}\n1  b'\\xe4\\xb3#\\xb5r\\x9c' bytearray(b'{\"topic\": \"/battery\", \"value\": 6.6}') {b'\\xe4\\xb3#\\xb5r\\x9c': [-23, 3999931], b'd\\xe83\\x86\\x8e\\xc8': [-30, 2747079]}\n1  b'\\xe4\\xb3#\\xb5r\\x9c' bytearray(b'{\"topic\": \"/battery\", \"value\": 6.7}') {b'\\xe4\\xb3#\\xb5r\\x9c': [-24, 4066042], b'd\\xe83\\x86\\x8e\\xc8': [-30, 2747079]}\n1  b'\\xe4\\xb3#\\xb5r\\x9c' bytearray(b'{\"topic\": \"/battery\", \"value\": 6.8}') {b'\\xe4\\xb3#\\xb5r\\x9c': [-25, 4132154], b'd\\xe83\\x86\\x8e\\xc8': [-30, 2747079]}\n1  b'\\xe4\\xb3#\\xb5r\\x9c' bytearray(b'{\"topic\": \"/battery\", \"value\": 7.0}') {b'\\xe4\\xb3#\\xb5r\\x9c': [-25, 4198270], b'd\\xe83\\x86\\x8e\\xc8': [-30, 2747079]}\n1  b'\\xe4\\xb3#\\xb5r\\x9c' bytearray(b'{\"topic\": \"/battery\", \"value\": 7.1}') {b'\\xe4\\xb3#\\xb5r\\x9c': [-25, 4264388], b'd\\xe83\\x86\\x8e\\xc8': [-30, 2747079]}\n1  b'\\xe4\\xb3#\\xb5r\\x9c' bytearray(b'{\"topic\": \"/battery\", \"value\": 7.3}') {b'\\xe4\\xb3#\\xb5r\\x9c': [-25, 4330508], b'd\\xe83\\x86\\x8e\\xc8': [-30, 2747079]}\n1  b'\\xe4\\xb3#\\xb5r\\x9c' bytearray(b'{\"topic\": \"/battery\", \"value\": 7.4}') {b'\\xe4\\xb3#\\xb5r\\x9c': [-25, 4396629], b'd\\xe83\\x86\\x8e\\xc8': [-30, 2747079]}\n1  b'\\xe4\\xb3#\\xb5r\\x9c' bytearray(b'{\"topic\": \"/battery\", \"value\": 7.6}') {b'\\xe4\\xb3#\\xb5r\\x9c': [-16, 4462740], b'd\\xe83\\x86\\x8e\\xc8': [-30, 2747079]}\n1  b'\\xe4\\xb3#\\xb5r\\x9c' bytearray(b'{\"topic\": \"/battery\", \"value\": 7.8}') {b'\\xe4\\xb3#\\xb5r\\x9c': [-19, 4528852], b'd\\xe83\\x86\\x8e\\xc8': [-30, 2747079]}\n1  b'\\xe4\\xb3#\\xb5r\\x9c' bytearray(b'{\"topic\": \"/battery\", \"value\": 7.9}') {b'\\xe4\\xb3#\\xb5r\\x9c': [-18, 4594963], b'd\\xe83\\x86\\x8e\\xc8': [-30, 2747079]}\n1  b'\\xe4\\xb3#\\xb5r\\x9c' bytearray(b'{\"topic\": \"/battery\", \"value\": 8.2}') {b'\\xe4\\xb3#\\xb5r\\x9c': [-16, 4661078], b'd\\xe83\\x86\\x8e\\xc8': [-30, 2747079]}\n1  b'\\xe4\\xb3#\\xb5r\\x9c' bytearray(b'{\"topic\": \"/battery\", \"value\": 8.4}') {b'\\xe4\\xb3#\\xb5r\\x9c': [-15, 4727186], b'd\\xe83\\x86\\x8e\\xc8': [-30, 2747079]}\n1  b'\\xe4\\xb3#\\xb5r\\x9c' bytearray(b'{\"topic\": \"/battery\", \"value\": 8.6}') {b'\\xe4\\xb3#\\xb5r\\x9c': [-16, 4793297], b'd\\xe83\\x86\\x8e\\xc8': [-30, 2747079]}\n1  b'\\xe4\\xb3#\\xb5r\\x9c' bytearray(b'{\"topic\": \"/battery\", \"value\": 8.8}') {b'\\xe4\\xb3#\\xb5r\\x9c': [-16, 4859409], b'd\\xe83\\x86\\x8e\\xc8': [-30, 2747079]}\n1  b'\\xe4\\xb3#\\xb5r\\x9c' bytearray(b'{\"topic\": \"/battery\", \"value\": 9.1}') {b'\\xe4\\xb3#\\xb5r\\x9c': [-19, 4925521], b'd\\xe83\\x86\\x8e\\xc8': [-30, 2747079]}\n1  b'\\xe4\\xb3#\\xb5r\\x9c' bytearray(b'{\"topic\": \"/battery\", \"value\": 9.3}') {b'\\xe4\\xb3#\\xb5r\\x9c': [-18, 4991632], b'd\\xe83\\x86\\x8e\\xc8': [-30, 2747079]}\n1  b'\\xe4\\xb3#\\xb5r\\x9c' bytearray(b'{\"topic\": \"/battery\", \"value\": 9.6}') {b'\\xe4\\xb3#\\xb5r\\x9c': [-17, 5057743], b'd\\xe83\\x86\\x8e\\xc8': [-30, 2747079]}\n1  b'\\xe4\\xb3#\\xb5r\\x9c' bytearray(b'{\"topic\": \"/battery\", \"value\": 9.8}') {b'\\xe4\\xb3#\\xb5r\\x9c': [-17, 5123861], b'd\\xe83\\x86\\x8e\\xc8': [-30, 2747079]}\n1  b'\\xe4\\xb3#\\xb5r\\x9c' bytearray(b'{\"topic\": \"/battery\", \"value\": 10.1}') {b'\\xe4\\xb3#\\xb5r\\x9c': [-16, 5189976], b'd\\xe83\\x86\\x8e\\xc8': [-30, 2747079]}\n1  b'\\xe4\\xb3#\\xb5r\\x9c' bytearray(b'{\"topic\": \"/battery\", \"value\": 10.4}') {b'\\xe4\\xb3#\\xb5r\\x9c': [-16, 5256087], b'd\\xe83\\x86\\x8e\\xc8': [-30, 2747079]}\n1  b'\\xe4\\xb3#\\xb5r\\x9c' bytearray(b'{\"topic\": \"/battery\", \"value\": 10.7}') {b'\\xe4\\xb3#\\xb5r\\x9c': [-18, 5322200], b'd\\xe83\\x86\\x8e\\xc8': [-30, 2747079]}\n1  b'\\xe4\\xb3#\\xb5r\\x9c' bytearray(b'{\"topic\": \"/battery\", \"value\": 11.0}') {b'\\xe4\\xb3#\\xb5r\\x9c': [-17, 5388310], b'd\\xe83\\x86\\x8e\\xc8': [-30, 2747079]}\n1  b'\\xe4\\xb3#\\xb5r\\x9c' bytearray(b'{\"topic\": \"/battery\", \"value\": 11.4}') {b'\\xe4\\xb3#\\xb5r\\x9c': [-17, 5454422], b'd\\xe83\\x86\\x8e\\xc8': [-30, 2747079]}\n1  b'\\xe4\\xb3#\\xb5r\\x9c' bytearray(b'{\"topic\": \"/battery\", \"value\": 11.7}') {b'\\xe4\\xb3#\\xb5r\\x9c': [-18, 5520533], b'd\\xe83\\x86\\x8e\\xc8': [-30, 2747079]}\n1  b'\\xe4\\xb3#\\xb5r\\x9c' bytearray(b'{\"topic\": \"/battery\", \"value\": 12.0}') {b'\\xe4\\xb3#\\xb5r\\x9c': [-17, 5586644], b'd\\xe83\\x86\\x8e\\xc8': [-30, 2747079]}\n1  b'\\xe4\\xb3#\\xb5r\\x9c' bytearray(b'{\"topic\": \"/battery\", \"value\": 12.4}') {b'\\xe4\\xb3#\\xb5r\\x9c': [-17, 5652756], b'd\\xe83\\x86\\x8e\\xc8': [-30, 2747079]}\n1  b'\\xe4\\xb3#\\xb5r\\x9c' bytearray(b'{\"topic\": \"/battery\", \"value\": 12.7}') {b'\\xe4\\xb3#\\xb5r\\x9c': [-18, 5718867], b'd\\xe83\\x86\\x8e\\xc8': [-30, 2747079]}\n1  b'\\xe4\\xb3#\\xb5r\\x9c' bytearray(b'{\"topic\": \"/battery\", \"value\": 13.1}') {b'\\xe4\\xb3#\\xb5r\\x9c': [-17, 5784978], b'd\\xe83\\x86\\x8e\\xc8': [-30, 2747079]}\n1  b'\\xe4\\xb3#\\xb5r\\x9c' bytearray(b'{\"topic\": \"/battery\", \"value\": 13.5}') {b'\\xe4\\xb3#\\xb5r\\x9c': [-18, 5851090], b'd\\xe83\\x86\\x8e\\xc8': [-30, 2747079]}\n1  b'\\xe4\\xb3#\\xb5r\\x9c' bytearray(b'{\"topic\": \"/battery\", \"value\": 13.9}') {b'\\xe4\\xb3#\\xb5r\\x9c': [-17, 5917201], b'd\\xe83\\x86\\x8e\\xc8': [-30, 2747079]}\n1  b'\\xe4\\xb3#\\xb5r\\x9c' bytearray(b'{\"topic\": \"/battery\", \"value\": 14.2}') {b'\\xe4\\xb3#\\xb5r\\x9c': [-17, 5983313], b'd\\xe83\\x86\\x8e\\xc8': [-30, 2747079]}\n1  b'\\xe4\\xb3#\\xb5r\\x9c' bytearray(b'{\"topic\": \"/battery\", \"value\": 14.6}') {b'\\xe4\\xb3#\\xb5r\\x9c': 1  b'\\xe4\\xb3#\\xb5r\\x9c' bytearray(b'{\"topic\": \"/battery\", \"value\": 15.1}') {b'\\xe4\\xb3#\\xb5r\\x9c': [-17, 6115535], b'd\\xe83\\x86\\x8e\\xc8': [-30, 2747079]}\n1  b'\\xe4\\xb3#\\xb5r\\x9c' bytearray(b'{\"topic\": \"/battery\", \"value\": 15.5}') {b'\\xe4\\xb3#\\xb5r\\x9c': [-18, 6181647], b'd\\xe83\\x86\\x8e\\xc8': [-30, 2747079]}\n1  b'\\xe4\\xb3#\\xb5r\\x9c' bytearray(b'{\"topic\": \"/battery\", \"value\": 15.9}') {b'\\xe4\\xb3#\\xb5r\\x9c': ue\": 17.2}') {b'\\xe4\\xb3#\\xb5r\\x9c': [-18, 6446092], b'd\\xe83\\x86\\x8e\\xc8': [-30, 2747079]}\n1  b'\\xe4\\xb3#\\xb5r\\x9c' bytearray(b'{\"topic\": \"/battery\", \"value\": 17.6}') {b'\\xe4\\xb3#\\xb5r\\x9c': [-24, 6512204], b'd\\xe83\\x86\\x8e\\xc8': [-30, 2747079]}\n1  b'\\xe4\\xb3#\\xb5r\\x9c' bytearray(b'{\"topic\": \"/battery\", \"value\": 18.1}') {b'\\xe4\\xb3#\\xb5r\\x9c': [-24, 6578315], b'd\\xe83\\x86\\x8e\\xc8': [-30, 2747079]}\n1  b'\\xe4\\xb3#\\xb5r\\x9c' bytearray(b'{\"topic\": \"/battery\", \"value\": 18.6}') {b'\\xe4\\xb3#\\xb5r\\x9c': [-23, 6644427], b'd\\xe83\\x86\\x8e\\xc8': [-30, 2747079]}\n1  b'\\xe4\\xb3#\\xb5r\\x9c' bytearray(b'{\"topic\": \"/battery\", \"value\": 19.0}') {b'\\xe4\\xb3#\\xb5r\\x9c': [-21, 6710539], b'd\\xe83\\x86\\x8e\\xc8': [-30, 2747079]}\n1  b'\\xe4\\xb3#\\xb5r\\x9c' bytearray(b'{\"topic\": \"/battery\", \"value\": 19.5}') {b'\\xe4\\xb3#\\xb5r\\x9c': [-21, 6776649], b'd\\xe83\\x86\\x8e\\xc8': [-30, 2747079]}\n1  b'\\xe4\\xb3#\\xb5r\\x9c' bytearray(b'{\"topic\": \"/battery\", \"value\": 20.0}') {b'\\xe4\\xb3#\\xb5r\\x9c': [-22, 6842761], b'd\\xe83\\x86\\x8e\\xc8': [-30, 2747079]}\n1  b'\\xe4\\xb3#\\xb5r\\x9c' bytearray(b'{\"topic\": \"/battery\", \"value\": 20.4}') {b'\\xe4\\xb3#\\xb5r\\x9c': [-22, 6908872], b'd\\xe83\\x86\\x8e\\xc8': [-30, 2747079]}\n1  b'\\xe4\\xb3#\\xb5r\\x9c' bytearray(b'{\"topic\": \"/battery\", \"value\": 20.9}') {b'\\xe4\\xb3#\\xb5r\\x9c': [-21, 6974983], b'd\\xe83\\x86\\x8e\\xc8': [-30, 2747079]}\n1  b'\\xe4\\xb3#\\xb5r\\x9c' bytearray(b'{\"topic\": \"/battery\", \"value\": 21.4}') {b'\\xe4\\xb3#\\xb5r\\x9c': [-21, 7041099], b'd\\xe83\\x86\\x8e\\xc8': [-30, 2747079]}\n1  b'\\xe4\\xb3#\\xb5r\\x9c' bytearray(b'{\"topic\": \"/battery\", \"value\": 21.9}') {b'\\xe4\\xb3#\\xb5r\\x9c': [-21, 7107206], b'd\\xe83\\x86\\x8e\\xc8': [-30, 2747079]}\n1  b'\\xe4\\xb3#\\xb5r\\x9c' bytearray(b'{\"topic\": \"/battery\", \"value\": 22.4}') {b'\\xe4\\xb3#\\xb5r\\x9c': [-21, 7173318], b'd\\xe83\\x86\\x8e\\xc8': [-30, 2747079]}\n1  b'\\xe4\\xb3#\\xb5r\\x9c' bytearray(b'{\"topic\": \"/battery\", \"value\": 22.9}') {b'\\xe4\\xb3#\\xb5r\\x9c': [-22, 7239430], b'd\\xe83\\x86\\x8e\\xc8': [-30, 2747079]}\n1  b'\\xe4\\xb3#\\xb5r\\x9c' bytearray(b'{\"topic\": \"/battery\", \"value\": 23.5}') {b'\\xe4\\xb3#\\xb5r\\x9c': [-22, 7305542], b'd\\xe83\\x86\\x8e\\xc8': [-30, 2747079]}\n1  b'\\xe4\\xb3#\\xb5r\\x9c' bytearray(b'{\"topic\": \"/battery\", \"value\": 24.0}') {b'\\xe4\\xb3#\\xb5r\\x9c': [-23, 7371652], b'd\\xe83\\x86\\x8e\\xc8': [-30, 2747079]}\n1  b'\\xe4\\xb3#\\xb5r\\x9c' bytearray(b'{\"topic\": \"/battery\", \"value\": 24.5}') {b'\\xe4\\xb3#\\xb5r\\x9c': [-22, 7437780], b'd\\xe83\\x86\\x8e\\xc8': [-30, 2747079]}\n1  b'\\xe4\\xb3#\\xb5r\\x9c' bytearray(b'{\"topic\": \"/battery\", \"value\": 25.1}') {b'\\xe4\\xb3#\\xb5r\\x9c': [-24, 7503894], b'd\\xe83\\x86\\x8e\\xc8': [-30, 2747079]}\n1  b'\\xe4\\xb3#\\xb5r\\x9c' bytearray(b'{\"topic\": \"/battery\", \"value\": 25.7}') {b'\\xe4\\xb3#\\xb5r\\x9c': [-22, 7570006], b'd\\xe83\\x86\\x8e\\xc8': [-30, 2747079]}\n1  b'\\xe4\\xb3#\\xb5r\\x9c' bytearray(b'{\"topic\": \"/battery\", \"value\": 26.2}') {b'\\xe4\\xb3#\\xb5r\\x9c': [-23, 7636118], b'd\\xe83\\x86\\x8e\\xc8': [-30, 2747079]}\n1  b'\\xe4\\xb3#\\xb5r\\x9c' bytearray(b'{\"topic\": \"/battery\", \"value\": 26.8}') {b'\\xe4\\xb3#\\xb5r\\x9c': [-22, 7702229], b'd\\xe83\\x86\\x8e\\xc8': [-30, 2747079]}\n1  b'\\xe4\\xb3#\\xb5r\\x9c' bytearray(b'{\"topic\": \"/battery\", \"value\": 27.4}') {b'\\xe4\\xb3#\\xb5r\\x9c': [-25, 7768340], b'd\\xe83\\x86\\x8e\\xc8': [-30, 2747079]}\n1  b'\\xe4\\xb3#\\xb5r\\x9c' bytearray(b'{\"topic\": \"/battery\", \"value\": 28.0}') {b'\\xe4\\xb3#\\xb5r\\x9c': [-23, 7834451], b'd\\xe83\\x86\\x8e\\xc8': [-30, 2747079]}\n1  b'\\xe4\\xb3#\\xb5r\\x9c' bytearray(b'{\"topic\": \"/battery\", \"value\": 28.6}') {b'\\xe4\\xb3#\\xb5r\\x9c': [-23, 7900563], b'd\\xe83\\x86\\x8e\\xc8': [-30, 2747079]}\n1  b'\\xe4\\xb3#\\xb5r\\x9c' bytearray(b'{\"topic\": \"/battery\", \"value\": 29.2}') {b'\\xe4\\xb3#\\xb5r\\x9c': [-22, 7966674], b'd\\xe83\\x86\\x8e\\xc8': [-30, 2747079]}\n1  b'\\xe4\\xb3#\\xb5r\\x9c' bytearray(b'{\"topic\": \"/battery\", \"value\": 29.8}') {b'\\xe4\\xb3#\\xb5r\\x9c': [-24, 8032786], b'd\\xe83\\x86\\x8e\\xc8': [-30, 2747079]}\n1  b'\\xe4\\xb3#\\xb5r\\x9c' bytearray(b'{\"topic\": \"/battery\", \"value\": 30.4}') {b'\\xe4\\xb3#\\xb5r\\x9c': [-23, 8098897], b'd\\xe83\\x86\\x8e\\xc8': [-30, 2747079]}\n1  b'\\xe4\\xb3#\\xb5r\\x9c' bytearray(b'{\"topic\": \"/battery\", \"value\": 31.1}') {b'\\xe4\\xb3#\\xb5r\\x9c': [-26, 8165008], b'd\\xe83\\x86\\x8e\\xc8': [-30, 2747079]}\n1  b'\\xe4\\xb3#\\xb5r\\x9c' bytearray(b'{\"topic\": \"/battery\", \"value\": 31.7}') {b'\\xe4\\xb3#\\xb5r\\x9c': [-24, 8231121], b'd\\xe83\\x86\\x8e\\xc8': [-30, 2747079]}\n1  b'\\xe4\\xb3#\\xb5r\\x9c' bytearray(b'{\"topic\": \"/battery\", \"value\": 32.3}') {b'\\xe4\\xb3#\\xb5r\\x9c': [-23, 8297231], b'd\\xe83\\x86\\x8e\\xc8': [-30, 2747079]}\n1  b'\\xe4\\xb3#\\xb5r\\x9c' bytearray(b'{\"topic\": \"/battery\", \"value\": 33.0}') {b'\\xe4\\xb3#\\xb5r\\x9c': [-22, 8363343], b'd\\xe83\\x86\\x8e\\xc8': [-30, 2747079]}\n1  b'\\xe4\\xb3#\\xb5r\\x9c' bytearray(b'{\"topic\": \"/battery\", \"value\": 33.7}') {b'\\xe4\\xb3#\\xb5r\\x9c': [-23, 8429454], b'd\\xe83\\x86\\x8e\\xc8': [-30, 2747079]}\n1  b'\\xe4\\xb3#\\xb5r\\x9c' bytearray(b'{\"topic\": \"/battery\", \"value\": 34.3}') {b'\\xe4\\xb3#\\xb5r\\x9c': [-22, 8495565], b'd\\xe83\\x86\\x8e\\xc8': [-30, 2747079]}\n1  b'\\xe4\\xb3#\\xb5r\\x9c' bytearray(b'{\"topic\": \"/battery\", \"value\": 35.0}') {b'\\xe4\\xb3#\\xb5r\\x9c': [-22, 8561677], b'd\\xe83\\x86\\x8e\\xc8': [-30, 2747079]}\n1  b'\\xe4\\xb3#\\xb5r\\x9c' bytearray(b'{\"topic\": \"/battery\", \"value\": 35.7}') {b'\\xe4\\xb3#\\xb5r\\x9c': [-24, 8627789], b'd\\xe83\\x86\\x8e\\xc8': [-30, 2747079]}\n1  b'\\xe4\\xb3#\\xb5r\\x9c' bytearray(b'{\"topic\": \"/battery\", \"value\": 36.4}') {b'\\xe4\\xb3#\\xb5r\\x9c': [-23, 8693900], b'd\\xe83\\x86\\x8e\\xc8': [-30, 2747079]}\n1  b'\\xe4\\xb3#\\xb5r\\x9c' bytearray(b'{\"topic\": \"/battery\", \"value\": 37.1}') {b'\\xe4\\xb3#\\xb5r\\x9c': [-23, 8760011], b'd\\xe83\\x86\\x8e\\xc8': [-30, 2747079]}\n1  b'\\xe4\\xb3#\\xb5r\\x9c' bytearray(b'{\"topic\": \"/battery\", \"value\": 37.8}') {b'\\xe4\\xb3#\\xb5r\\x9c': [-23, 8826123], b'd\\xe83\\x86\\x8e\\xc8': [-30, 2747079]}\n1  b'\\xe4\\xb3#\\xb5r\\x9c' bytearray(b'{\"topic\": \"/battery\", \"value\": 38.5}') {b'\\xe4\\xb3#\\xb5r\\x9c': [-23, 8892234], b'd\\xe83\\x86\\x8e\\xc8': [-30, 2747079]}\n1  b'\\xe4\\xb3#\\xb5r\\x9c' bytearray(b'{\"topic\": \"/battery\", \"value\": 39.2}') {b'\\xe4\\xb3#\\xb5r\\x9c': [-23, 8958345], b'd\\xe83\\x86\\x8e\\xc8': [-30, 2747079]}\n1  b'\\xe4\\xb3#\\xb5r\\x9c' bytearray(b'{\"topic\": \"/battery\", \"value\": 39.9}') {b'\\xe4\\xb3#\\xb5r\\x9c': [-23, 9024457], b'd\\xe83\\x86\\x8e\\xc8': [-30, 2747079]}\n1  b'\\xe4\\xb3#\\xb5r\\x9c' bytearray(b'{\"topic\": \"/battery\", \"value\": 40.6}') {b'\\xe4\\xb3#\\xb5r\\x9c': [-23, 9090568], b'd\\xe83\\x86\\x8e\\xc8': [-30, 2747079]}\n1  b'\\xe4\\xb3#\\xb5r\\x9c' bytearray(b'{\"topic\": \"/battery\", \"value\": 41.4}') {b'\\xe4\\xb3#\\xb5r\\x9c': [-23, 9156682], b'd\\xe83\\x86\\x8e\\xc8': [-30, 2747079]}\n1  b'\\xe4\\xb3#\\xb5r\\x9c' bytearray(b'{\"topic\": \"/battery\", \"value\": 42.1}') {b'\\xe4\\xb3#\\xb5r\\x9c': [-23, 9222791], b'd\\xe83\\x86\\x8e\\xc8': [-30, 2747079]}\n1  b'\\xe4\\xb3#\\xb5r\\x9c' bytearray(b'{\"topic\": \"/battery\", \"value\": 42.8}') {b'\\xe4\\xb3#\\xb5r\\x9c': [-23, 9288905], b'd\\xe83\\x86\\x8e\\xc8': [-30, 2747079]}\n1  b'\\xe4\\xb3#\\xb5r\\x9c' bytearray(b'{\"topic\": \"/battery\", \"value\": 43.6}') {b'\\xe4\\xb3#\\xb5r\\x9c': \\xb5r\\x9c' bytearray(b'{\"topic\": \"/battery\", \"value\": 53.7}') {b'\\xe4\\xb3#\\xb5r\\x9c': [-23, 10280573], b'd\\xe83\\x86\\x8e\\xc8': [-30, 2747079]}\n1  b'\\xe4\\xb3#\\xb5r\\x9c' bytearray(b'{\"topic\": \"/battery\", \"value\": 54.4}') {b'\\xe4\\xb3#\\xb5r\\x9c': [-23, 10346684], b'd\\xe83\\x86\\x8e\\xc8': [-30, 2747079]}\n1  b'\\xe4\\xb3#\\xb5r\\x9c' bytearray(b'{\"topic\": \"/battery\", \"value\": 55.1}') {b'\\xe4\\xb3#\\xb5r\\x9c': [-23, 10412796], b'd\\xe83\\x86\\x8e\\xc8': [-30, 2747079]}\n1  b'\\xe4\\xb3#\\xb5r\\x9c' bytearray(b'{\"topic\": \"/battery\", \"value\": 55.8}') {b'\\xe4\\xb3#\\xb5r\\x9c': [-22, 10478908], b'd\\xe83\\x86\\x8e\\xc8': [-30, 2747079]}\n1  b'\\xe4\\xb3#\\xb5r\\x9c' bytearray(b'{\"topic\": \"/battery\", \"value\": 56.5}') {b'\\xe4\\xb3#\\xb5r\\x9c': [-23, 10545019], b'd\\xe83\\x86\\x8e\\xc8': [-30, 2747079]}\n1  b'\\xe4\\xb3#\\xb5r\\x9c' bytearray(b'{\"topic\": \"/battery\", \"value\": 57.2}') {b'\\xe4\\xb3#\\xb5r\\x9c': [-23, 10611130], b'd\\xe83\\x86\\x8e\\xc8': [-30, 2747079]}\n1  b'\\xe4\\xb3#\\xb5r\\x9c' bytearray(b'{\"topic\": \"/battery\", \"value\": 57.9}') {b'\\xe4\\xb3#\\xb5r\\x9c': [-23, 10677241], b'd\\xe83\\x86\\x8e\\xc8': [-30, 2747079]}\n1  b'\\xe4\\xb3#\\xb5r\\x9c' bytearray(b'{\"topic\": \"/battery\", \"value\": 58.6}') {b'\\xe4\\xb3#\\xb5r\\x9c': [-23, 10743353], b'd\\xe83\\x86\\x8e\\xc8': [-30, 2747079]}\n1  b'\\xe4\\xb3#\\xb5r\\x9c' bytearray(b'{\"topic\": \"/battery\", \"value\": 59.3}') {b'\\xe4\\xb3#\\xb5r\\x9c': [-23, 10809464], b'd\\xe83\\x86\\x8e\\xc8': [-30, 2747079]}\n1  b'\\xe4\\xb3#\\xb5r\\x9c' bytearray(b'{\"topic\": \"/battery\", \"value\": 60.0}') {b'\\xe4\\xb3#\\xb5r\\x9c': [-23, 10875575], b'd\\xe83\\x86\\x8e\\xc8': [-30, 2747079]}\n1  b'\\xe4\\xb3#\\xb5r\\x9c' bytearray(b'{\"topic\": \"/battery\", \"value\": 60.7}') {b'\\xe4\\xb3#\\xb5r\\x9c': [-23, 10941687], b'd\\xe83\\x86\\x8e\\xc8': [-30, 2747079]}\n1  b'\\xe4\\xb3#\\xb5r\\x9c' bytearray(b'{\"topic\": \"/battery\", \"value\": 61.3}') {b'\\xe4\\xb3#\\xb5r\\x9c': [-22, 11007801], b'd\\xe83\\x86\\x8e\\xc8': [-30, 2747079]}\n1  b'\\xe4\\xb3#\\xb5r\\x9c' bytearray(b'{\"topic\": \"/battery\", \"value\": 62.0}') {b'\\xe4\\xb3#\\xb5r\\x9c': [-23, 11073913], b'd\\xe83\\x86\\x8e\\xc8': [-30, 2747079]}\n1  b'\\xe4\\xb3#\\xb5r\\x9c' bytearray(b'{\"topic\": \"/battery\", \"value\": 62.8}') {b'\\xe4\\xb3#\\xb5r\\x9c': [-23, 11140021], b'd\\xe83\\x86\\x8e\\xc8': [-30, 2747079]}\n1  b'\\xe4\\xb3#\\xb5r\\x9c' bytearray(b'{\"topic\": \"/battery\", \"value\": 63.5}') {b'\\xe4\\xb3#\\xb5r\\x9c': [-22, 11206132], b'd\\xe83\\x86\\x8e\\xc8': [-30, 2747079]}\n1  b'\\xe4\\xb3#\\xb5r\\x9c' bytearray(b'{\"topic\": \"/battery\", \"value\": 64.2}') {b'\\xe4\\xb3#\\xb5r\\x9c': [-23, 11272244], b'd\\xe83\\x86\\x8e\\xc8': [-30, 2747079]}\n1  b'\\xe4\\xb3#\\xb5r\\x9c' bytearray(b'{\"topic\": \"/battery\", \"value\": 64.9}') {b'\\xe4\\xb3#\\xb5r\\x9c': [-23, 11338355], b'd\\xe83\\x86\\x8e\\xc8': [-30, 2747079]}\n1  b'\\xe4\\xb3#\\xb5r\\x9c' bytearray(b'{\"topic\": \"/battery\", \"value\": 65.6}') {b'\\xe4\\xb3#\\xb5r\\x9c': [-23, 11404468], b'd\\xe83\\x86\\x8e\\xc8': [-30, 2747079]}\n1  b'\\xe4\\xb3#\\xb5r\\x9c' bytearray(b'{\"topic\": \"/battery\", \"value\": 66.3}') {b'\\xe4\\xb3#\\xb5r\\x9c': [-23, 11470578], b'd\\xe83\\x86\\x8e\\xc8': [-30, 2747079]}\n1  b'\\xe4\\xb3#\\xb5r\\x9c' bytearray(b'{\"topic\": \"/battery\", \"value\": 67.0}') {b'\\xe4\\xb3#\\xb5r\\x9c': [-23, 11536690], b'd\\xe83\\x86\\x8e\\xc8': [-30, 2747079]}\n1  b'\\xe4\\xb3#\\xb5r\\x9c' bytearray(b'{\"topic\": \"/battery\", \"value\": 67.7}') {b'\\xe4\\xb3#\\xb5r\\x9c': [-23, 11602802], b'd\\xe83\\x86\\x8e\\xc8': [-30, 2747079]}\n1  b'\\xe4\\xb3#\\xb5r\\x9c' bytearray(b'{\"topic\": \"/battery\", \"value\": 68.4}') {b'\\xe4\\xb3#\\xb5r\\x9c': [-23, 11668912], b'd\\xe83\\x86\\x8e\\xc8': [-30, 2747079]}\n1  b'\\xe4\\xb3#\\xb5r\\x9c' bytearray(b'{\"topic\": \"/battery\", \"value\": 69.1}') {b'\\xe4\\xb3#\\xb5r\\x9c': [-23, 11735024], b'd\\xe83\\x86\\x8e\\xc8': [-30, 2747079]}\n1  b'\\xe4\\xb3#\\xb5r\\x9c' bytearray(b'{\"topic\": \"/battery\", \"value\": 69.8}') {b'\\xe4\\xb3#\\xb5r\\x9c': [-23, 11801135], b'd\\xe83\\x86\\x8e\\xc8': [-30, 2747079]}\n1  b'\\xe4\\xb3#\\xb5r\\x9c' bytearray(b'{\"topic\": \"/battery\", \"value\": 70.5}') {b'\\xe4\\xb3#\\xb5r\\x9c': [-23, 11867246], b'd\\xe83\\x86\\x8e\\xc8': [-30, 2747079]}\n1  b'\\xe4\\xb3#\\xb5r\\x9c' bytearray(b'{\"topic\": \"/battery\", \"value\": 71.1}') {b'\\xe4\\xb3#\\xb5r\\x9c': [-23, 11933358], b'd\\xe83\\x86\\x8e\\xc8': [-30, 2747079]}\n1  b'\\xe4\\xb3#\\xb5r\\x9c' bytearray(b'{\"topic\": \"/battery\", \"value\": 71.8}') {b'\\xe4\\xb3#\\xb5r\\x9c': [-23, 11999469], b'd\\xe83\\x86\\x8e\\xc8': [-30, 2747079]}\n1  b'\\xe4\\xb3#\\xb5r\\x9c' bytearray(b'{\"topic\": \"/battery\", \"value\": 72.5}') {b'\\xe4\\xb3#\\xb5r\\x9c': [-22, 12065581], b'd\\xe83\\x86\\x8e\\xc8': [-30, 2747079]}\n1  b'\\xe4\\xb3#\\xb5r\\x9c' bytearray(b'{\"topic\": \"/battery\", \"value\": 73.1}') {b'\\xe4\\xb3#\\xb5r\\x9c': [-23, 12131694], b'd\\xe83\\x86\\x8e\\xc8': [-30, 2747079]}\n1  b'\\xe4\\xb3#\\xb5r\\x9c' bytearray(b'{\"topic\": \"/battery\", \"value\": 73.8}') {b'\\xe4\\xb3#\\xb5r\\x9c': [-23, 12197803], b'd\\xe83\\x86\\x8e\\xc8': [-30, 2747079]}\n1  b'\\xe4\\xb3#\\xb5r\\x9c' bytearray(b'{\"topic\": \"/battery\", \"value\": 74.4}') {b'\\xe4\\xb3#\\xb5r\\x9c': [-23, 12263915], b'd\\xe83\\x86\\x8e\\xc8': [-30, 2747079]}\n1  b'\\xe4\\xb3#\\xb5r\\x9c' bytearray(b'{\"topic\": \"/battery\", \"value\": 75.0}') {b'\\xe4\\xb3#\\xb5r\\x9c': [-23, 12330027], b'd\\xe83\\x86\\x8e\\xc8': [-30, 2747079]}\n1  b'\\xe4\\xb3#\\xb5r\\x9c' bytearray(b'{\"topic\": \"/battery\", \"value\": 75.6}') {b'\\xe4\\xb3#\\xb5r\\x9c': [-22, 12396138], b'd\\xe83\\x86\\x8e\\xc8': [-30, 2747079]}\n1  b'\\xe4\\xb3#\\xb5r\\x9c' bytearray(b'{\"topic\": \"/battery\", \"value\": 76.2}') {b'\\xe4\\xb3#\\xb5r\\x9c': [-22, 12462251], b'd\\xe83\\x86\\x8e\\xc8': [-30, 2747079]}\n1  b'\\xe4\\xb3#\\xb5r\\x9c' bytearray(b'{\"topic\": \"/battery\", \"value\": 76.8}') {b'\\xe4\\xb3#\\xb5r\\x9c': [-23, 12528360], b'd\\xe83\\x86\\x8e\\xc8': [-30, 2747079]}\n1  b'\\xe4\\xb3#\\xb5r\\x9c' bytearray(b'{\"topic\": \"/battery\", \"value\": 77.4}') {b'\\xe4\\xb3#\\xb5r\\x9c': [-23, 12594474], b'd\\xe83\\x86\\x8e\\xc8': [-30, 2747079]}\n1  b'\\xe4\\xb3#\\xb5r\\x9c' bytearray(b'{\"topic\": \"/battery\", \"value\": 78.0}') {b'\\xe4\\xb3#\\xb5r\\x9c': [-23, 12660583], b'd\\xe83\\x86\\x8e\\xc8': [-30, 2747079]}\n1  b'\\xe4\\xb3#\\xb5r\\x9c' bytearray(b'{\"topic\": \"/battery\", \"value\": 78.6}') {b'\\xe4\\xb3#\\xb5r\\x9c': [-23, 12726695], b'd\\xe83\\x86\\x8e\\xc8': [-30, 2747079]}\n1  b'\\xe4\\xb3#\\xb5r\\x9c' bytearray(b'{\"topic\": \"/battery\", \"value\": 79.1}') {b'\\xe4\\xb3#\\xb5r\\x9c': [-23, 12792806], b'd\\xe83\\x86\\x8e\\xc8': [-30, 2747079]}\n1  b'\\xe4\\xb3#\\xb5r\\x9c' bytearray(b'{\"topic\": \"/battery\", \"value\": 79.7}') {b'\\xe4\\xb3#\\xb5r\\x9c': [-23, 12858917], b'd\\xe83\\x86\\x8e\\xc8': [-30, 2747079]}\n1  b'\\xe4\\xb3#\\xb5r\\x9c' bytearray(b'{\"topic\": \"/battery\", \"value\": 80.3}') {b'\\xe4\\xb3#\\xb5r\\x9c': [-23, 12925029], b'd\\xe83\\x86\\x8e\\xc8': [-30, 2747079]}\n1  b'\\xe4\\xb3#\\xb5r\\x9c' bytearray(b'{\"topic\": \"/battery\", \"value\": 80.8}') {b'\\xe4\\xb3#\\xb5r\\x9c': [-23, 12991143], b'd\\xe83\\x86\\x8e\\xc8': [-30, 2747079]}\n1  b'\\xe4\\xb3#\\xb5r\\x9c' bytearray(b'{\"topic\": \"/battery\", \"value\": 81.4}') {b'\\xe4\\xb3#\\xb5r\\x9c': [-23, 13057253], b'd\\xe83\\x86\\x8e\\xc8': [-30, 2747079]}\n1  b'\\xe4\\xb3#\\xb5r\\x9c' bytearray(b'{\"topic\": \"/battery\", \"value\": 81.9}') {b'\\xe4\\xb3#\\xb5r\\x9c': [-23, 13123365], b'd\\xe83\\x86\\x8e\\xc8': [-30, 2747079]}\n1  b'\\xe4\\xb3#\\xb5r\\x9c' bytearray(b'{\"topic\": \"/battery\", \"value\": 82.5}') {b'\\xe4\\xb3#\\xb5r\\x9c': [-23, 13189474], b'd\\xe83\\x86\\x8e\\xc8': [-30, 2747079]}\n1  b'\\xe4\\xb3#\\xb5r\\x9c' bytearray(b'{\"topic\": \"/battery\", \"value\": 83.0}') {b'\\xe4\\xb3#\\xb5r\\x9c': [-23, 13255586], b'd\\xe83\\x86\\x8e\\xc8': [-30, 2747079]}\n1  b'\\xe4\\xb3#\\xb5r\\x9c' bytearray(b'{\"topic\": \"/battery\", \"value\": 83.6}') {b'\\xe4\\xb3#\\xb5r\\x9c': [-23, 13321699], b'd\\xe83\\x86\\x8e\\xc8': [-30, 2747079]}\n1  b'\\xe4\\xb3#\\xb5r\\x9c' bytearray(b'{\"topic\": \"/battery\", \"value\": 84.1}') {b'\\xe4\\xb3#\\xb5r\\x9c': [-23, 13387809], b'd\\xe83\\x86\\x8e\\xc8': [-30, 2747079]}\n1  b'\\xe4\\xb3#\\xb5r\\x9c' bytearray(b'{\"topic\": \"/battery\", \"value\": 84.6}') {b'\\xe4\\xb3#\\xb5r\\x9c': [-23, 13453922], b'd\\xe83\\x86\\x8e\\xc8': [-30, 2747079]}\n1  b'\\xe4\\xb3#\\xb5r\\x9c' bytearray(b'{\"topic\": \"/battery\", \"value\": 85.2}') {b'\\xe4\\xb3#\\xb5r\\x9c': [-23, 13520031], b'd\\xe83\\x86\\x8e\\xc8': [-30, 2747079]}\n1  b'\\xe4\\xb3#\\xb5r\\x9c' bytearray(b'{\"topic\": \"/battery\", \"value\": 85.7}') {b'\\xe4\\xb3#\\xb5r\\x9c': [-23, 13586143], b'd\\xe83\\x86\\x8e\\xc8': [-30, 2747079]}\n1  b'\\xe4\\xb3#\\xb5r\\x9c' bytearray(b'{\"topic\": \"/battery\", \"value\": 86.2}') {b'\\xe4\\xb3#\\xb5r\\x9c': [-23, 13652255], b'd\\xe83\\x86\\x8e\\xc8': [-30, 2747079]}\n1  b'\\xe4\\xb3#\\xb5r\\x9c' bytearray(b'{\"topic\": \"/battery\", \"value\": 86.7}') {b'\\xe4\\xb3#\\xb5r\\x9c': [-23, 13718365], b'd\\xe83\\x86\\x8e\\xc8': [-30, 2747079]}\n1  b'\\xe4\\xb3#\\xb5r\\x9c' bytearray(b'{\"topic\": \"/battery\", \"value\": 87.3}') {b'\\xe4\\xb3#\\xb5r\\x9c': [-23, 13784484], b'd\\xe83\\x86\\x8e\\xc8': [-30, 2747079]}\n1  b'\\xe4\\xb3#\\xb5r\\x9c' bytearray(b'{\"topic\": \"/battery\", \"value\": 87.8}') {b'\\xe4\\xb3#\\xb5r\\x9c': [-22, 13850600], b'd\\xe83\\x86\\x8e\\xc8': [-30, 2747079]}\n1  b'\\xe4\\xb3#\\xb5r\\x9c' bytearray(b'{\"topic\": \"/battery\", \"value\": 88.3}') {b'\\xe4\\xb3#\\xb5r\\x9c': [-22, 13916710], b'd\\xe83\\x86\\x8e\\xc8': [-30, 2747079]}\n1  b'\\xe4\\xb3#\\xb5r\\x9c' bytearray(b'{\"topic\": \"/battery\", \"value\": 88.9}') {b'\\xe4\\xb3#\\xb5r\\x9c': [-24, 13982822], b'd\\xe83\\x86\\x8e\\xc8': [-30, 2747079]}\n1  b'\\xe4\\xb3#\\xb5r\\x9c' bytearray(b'{\"topic\": \"/battery\", \"value\": 89.4}') {b'\\xe4\\xb3#\\xb5r\\x9c': [-23, 14048932], b'd\\xe83\\x86\\x8e\\xc8': [-30, 2747079]}\n1  b'\\xe4\\xb3#\\xb5r\\x9c' bytearray(b'{\"topic\": \"/battery\", \"value\": 90.0}') {b'\\xe4\\xb3#\\xb5r\\x9c': [-22, 14115046], b'd\\xe83\\x86\\x8e\\xc8': [-30, 2747079]}\n1  b'\\xe4\\xb3#\\xb5r\\x9c' bytearray(b'{\"topic\": \"/battery\", \"value\": 90.5}') {b'\\xe4\\xb3#\\xb5r\\x9c': [-22, 14181155], b'd\\xe83\\x86\\x8e\\xc8': [-30, 2747079]}\n1  b'\\xe4\\xb3#\\xb5r\\x9c' bytearray(b'{\"topic\": \"/battery\", \"value\": 91.0}') {b'\\xe4\\xb3#\\xb5r\\x9c': [-23, 14247267], b'd\\xe83\\x86\\x8e\\xc8': [-30, 2747079]}\n1  b'\\xe4\\xb3#\\xb5r\\x9c' bytearray(b'{\"topic\": \"/battery\", \"value\": 91.4}') {b'\\xe4\\xb3#\\xb5r\\x9c': [-23, 14313378], b'd\\xe83\\x86\\x8e\\xc8': [-30, 2747079]}\n1  b'\\xe4\\xb3#\\xb5r\\x9c' bytearray(b'{\"topic\": \"/battery\", \"value\": 91.9}') {b'\\xe4\\xb3#\\xb5r\\x9c': [-23, 14379490], b'd\\xe83\\x86\\x8e\\xc8': [-30, 2747079]}\n1  b'\\xe4\\xb3#\\xb5r\\x9c' bytearray(b'{\"topic\": \"/battery\", \"value\": 92.3}') {b'\\xe4\\xb3#\\xb5r\\x9c': [-22, 14445603], b'd\\xe83\\x86\\x8e\\xc8': [-30, 2747079]}\n1  b'\\xe4\\xb3#\\xb5r\\x9c' bytearray(b'{\"topic\": \"/battery\", \"value\": 92.7}') {b'\\xe4\\xb3#\\xb5r\\x9c': [-22, 14511714], b'd\\xe83\\x86\\x8e\\xc8': [-30, 2747079]}\n1  b'\\xe4\\xb3#\\xb5r\\x9c' bytearray(b'{\"topic\": \"/battery\", \"value\": 93.1}') {b'\\xe4\\xb3#\\xb5r\\x9c': [-22, 14577824], b'd\\xe83\\x86\\x8e\\xc8': [-30, 2747079]}\n1  b'\\xe4\\xb3#\\xb5r\\x9c' bytearray(b'{\"topic\": \"/battery\", \"value\": 93.5}') {b'\\xe4\\xb3#\\xb5r\\x9c': [-23, 14643935], b'd\\xe83\\x86\\x8e\\xc8': [-30, 2747079]}\n1  b'\\xe4\\xb3#\\xb5r\\x9c' bytearray(b'{\"topic\": \"/battery\", \"value\": 93.9}') {b'\\xe4\\xb3#\\xb5r\\x9c': [-22, 14710046], b'd\\xe83\\x86\\x8e\\xc8': [-30, 2747079]}\n1  b'\\xe4\\xb3#\\xb5r\\x9c' bytearray(b'{\"topic\": \"/battery\", \"value\": 94.3}') {b'\\xe4\\xb3#\\xb5r\\x9c': [-23, 14776160], b'd\\xe83\\x86\\x8e\\xc8': [-30, 2747079]}\n1  b'\\xe4\\xb3#\\xb5r\\x9c' bytearray(b'{\"topic\": \"/battery\", \"value\": 94.6}') {b'\\xe4\\xb3#\\xb5r\\x9c': [-22, 14842270], b'd\\xe83\\x86\\x8e\\xc8': [-30, 2747079]}\n1  b'\\xe4\\xb3#\\xb5r\\x9c' bytearray(b'{\"topic\": \"/battery\", \"value\": 94.9}') {b'\\xe4\\xb3#\\xb5r\\x9c': [-23, 14908380], b'd\\xe83\\x86\\x8e\\xc8': [-30, 2747079]}\n1  b'\\xe4\\xb3#\\xb5r\\x9c' bytearray(b'{\"topic\": \"/battery\", \"value\": 95.2}') {b'\\xe4\\xb3#\\xb5r\\x9c': [-22, 14974492], b'd\\xe83\\x86\\x8e\\xc8': [-30, 2747079]}\n1  b'\\xe4\\xb3#\\xb5r\\x9c' bytearray(b'{\"topic\": \"/battery\", \"value\": 95.5}') {b'\\xe4\\xb3#\\xb5r\\x9c': [-23, 15040603], b'd\\xe83\\x86\\x8e\\xc8': [-30, 2747079]}\n1  b'\\xe4\\xb3#\\xb5r\\x9c' bytearray(b'{\"topic\": \"/battery\", \"value\": 95.8}') {b'\\xe4\\xb3#\\xb5r\\x9c': [-23, 15106715], b'd\\xe83\\x86\\x8e\\xc8': [-30, 2747079]}\n1  b'\\xe4\\xb3#\\xb5r\\x9c' bytearray(b'{\"topic\": \"/battery\", \"value\": 96.1}') {b'\\xe4\\xb3#\\xb5r\\x9c': [-23, 15172863], b'd\\xe83\\x86\\x8e\\xc8': [-30, 2747079]}\n1  b'\\xe4\\xb3#\\xb5r\\x9c' bytearray(b'{\"topic\": \"/battery\", \"value\": 96.3}') {b'\\xe4\\xb3#\\xb5r\\x9c': [-23, 15238981], b'd\\xe83\\x86\\x8e\\xc8': [-30, 2747079]}\n1  b'\\xe4\\xb3#\\xb5r\\x9c' bytearray(b'{\"topic\": \"/battery\", \"value\": 96.5}') {b'\\xe4\\xb3#\\xb5r\\x9c':1  b'\\xe4\\xb3#\\xb5r\\x9c' bytearray(b'{\"topic\": \"/battery\", \"value\": 96.7}') {b'\\xe4\\xb3#\\xb5r\\x9c': [-23, 15371200], b'd\\xe83\\x86\\x8e\\xc8': [-30, 2747079]}\n1  b'\\xe4\\xb3#\\xb5r\\x9c' bytearray(b'{\"topic\": \"/battery\", \"value\": 96.9}') {b'\\xe4\\xb3#\\xb5r\\x9c': [-22, 15437312], b'd\\xe83\\x86\\x8e\\xc8': [-30, 2747079]}\n1  b'\\xe4\\xb3#\\xb5r\\x9c' bytearray(b'{\"topic\": \"/battery\", \"value\": 97.0}') {b'\\xe4\\xb3#\\xb5r\\x9c': [-23, 15503425], b'd\\xe83\\x86\\x8e\\xc8': [-30, 2747079]}\n1  b'\\xe4\\xb3#\\xb5r\\x9c' bytearray(b'{\"topic\": \"/battery\", \"value\": 97.1}') {b'\\xe4\\xb3#\\xb5r\\x9c': [-23, 15569536], b'd\\xe83\\x86\\x8e\\xc8': [-30, 2747079]}\n1  b'\\xe4\\xb3#\\xb5r\\x9c' bytearray(b'{\"topic\": \"/battery\", \"value\": 97.3}') {b'\\xe4\\xb3#\\xb5r\\x9c': [-23, 15635646], b'd\\xe83\\x86\\x8e\\xc8': [-30, 2747079]}\n1  b'\\xe4\\xb3#\\xb5r\\x9c' bytearray(b'{\"topic\": \"/battery\", \"value\": 97.4}') {b'\\xe4\\xb3#\\xb5r\\x9c': [-23, 15701757], b'd\\xe83\\x86\\x8e\\xc8': [-30, 2747079]}\n1  b'\\xe4\\xb3#\\xb5r\\x9c' bytearray(b'{\"topic\": \"/battery\", \"value\": 97.5}') {b'\\xe4\\xb3#\\xb5r\\x9c': [-23, 15767868], b'd\\xe83\\x86\\x8e\\xc8': [-30, 2747079]}\n1  b'\\xe4\\xb3#\\xb5r\\x9c' bytearray(b'{\"topic\": \"/battery\", \"value\": 97.6}') {b'\\xe4\\xb3#\\xb5r\\x9c': [-22, 15833980], b'd\\xe83\\x86\\x8e\\xc8': [-30, 2747079]}\n1  b'\\xe4\\xb3#\\xb5r\\x9c' bytearray(b'{\"topic\": \"/battery\", \"value\": 97.8}') {b'\\xe4\\xb3#\\xb5r\\x9c': [-23, 15900092], b'd\\xe83\\x86\\x8e\\xc8': [-30, 2747079]}\n1  b'\\xe4\\xb3#\\xb5r\\x9c' bytearray(b'{\"topic\": \"/battery\", \"value\": 97.9}') {b'\\xe4\\xb3#\\xb5r\\x9c': [-23, 15966203], b'd\\xe83\\x86\\x8e\\xc8': [-30, 2747079]}\n1  b'\\xe4\\xb3#\\xb5r\\x9c' bytearray(b'{\"topic\": \"/battery\", \"value\": 98.0}') {b'\\xe4\\xb3#\\xb5r\\x9c': [-23, 16032314], b'd\\xe83\\x86\\x8e\\xc8': [-30, 2747079]}\n1  b'\\xe4\\xb3#\\xb5r\\x9c' bytearray(b'{\"topic\": \"/battery\", \"value\": 98.0}') {b'\\xe4\\xb3#\\xb5r\\x9c': [-23, 16098425], b'd\\xe83\\x86\\x8e\\xc8': [-30, 2747079]}\n1  b'\\xe4\\xb3#\\xb5r\\x9c' bytearray(b'{\"topic\": \"/battery\", \"value\": 98.0}') {b'\\xe4\\xb3#\\xb5r\\x9c': [-23, 16164537], b'd\\xe83\\x86\\x8e\\xc8': [-30, 2747079]}\n1  b'\\xe4\\xb3#\\xb5r\\x9c' bytearray(b'{\"topic\": \"/battery\", \"value\": 98.0}') {b'\\xe4\\xb3#\\xb5r\\x9c': [-23, 16230648], b'd\\xe83\\x86\\x8e\\xc8': [-30, 2747079]}\n1  b'\\xe4\\xb3#\\xb5r\\x9c' bytearray(b'{\"topic\": \"/battery\", \"value\": 98.0}') {b'\\xe4\\xb3#\\xb5r\\x9c': [-23, 16296759], b'd\\xe83\\x86\\x8e\\xc8': [-30, 2747079]}\n1  b'\\xe4\\xb3#\\xb5r\\x9c' bytearray(b'{\"topic\": \"/battery\", \"value\": 98.0}') {b'\\xe4\\xb3#\\xb5r\\x9c': [-23, 16362871], b'd\\xe83\\x86\\x8e\\xc8': [-30, 2747079]}\n1  b'\\xe4\\xb3#\\xb5r\\x9c' bytearray(b'{\"topic\": \"/battery\", \"value\": 98.0}') {b'\\xe4\\xb3#\\xb5r\\x9c': [-22, 16428984], b'd\\xe83\\x86\\x8e\\xc8': [-30, 2747079]}\n1  b'\\xe4\\xb3#\\xb5r\\x9c' bytearray(b'{\"topic\": \"/battery\", \"value\": 98.0}') {b'\\xe4\\xb3#\\xb5r\\x9c': [-23, 16495094], b'd\\xe83\\x86\\x8e\\xc8': [-30, 2747079]}\n1  b'\\xe4\\xb3#\\xb5r\\x9c' bytearray(b'{\"topic\": \"/battery\", \"value\": 98.0}') {b'\\xe4\\xb3#\\xb5r\\x9c': [-23, 16561205], b'd\\xe83\\x86\\x8e\\xc8': [-30, 2747079]}\n1  b'\\xe4\\xb3#\\xb5r\\x9c' bytearray(b'{\"topic\": \"/battery\", \"value\": 98.0}') {b'\\xe4\\xb3#\\xb5r\\x9c': [-23, 16627317], b'd\\xe83\\x86\\x8e\\xc8': [-30, 2747079]}\n1  b'\\xe4\\xb3#\\xb5r\\x9c' bytearray(b'{\"topic\": \"/battery\", \"value\": 98.0}') {b'\\xe4\\xb3#\\xb5r\\x9c': [-22, 16693428], b'd\\xe83\\x86\\x8e\\xc8': [-30, 2747079]}\n1  b'\\xe4\\xb3#\\xb5r\\x9c' bytearray(b'{\"topic\": \"/battery\", \"value\": 98.0}') {b'\\xe4\\xb3#\\xb5r\\x9c': [-23, 16759539], b'd\\xe83\\x86\\x8e\\xc8': [-30, 2747079]}\n1  b'\\xe4\\xb3#\\xb5r\\x9c' bytearray(b'{\"topic\": \"/battery\", \"value\": 98.0}') {b'\\xe4\\xb3#\\xb5r\\x9c': [-23, 16825650], b'd\\xe83\\x86\\x8e\\xc8': [-30, 2747079]}\n1  b'\\xe4\\xb3#\\xb5r\\x9c' bytearray(b'{\"topic\": \"/battery\", \"value\": 98.0}') {b'\\xe4\\xb3#\\xb5r\\x9c': [-22, 16891762], b'd\\xe83\\x86\\x8e\\xc8': [-30, 2747079]}\n1  b'\\xe4\\xb3#\\xb5r\\x9c' bytearray(b'{\"topic\": \"/battery\", \"value\": 98.0}') {b'\\xe4\\xb3#\\xb5r\\x9c': [-22, 16957873], b'd\\xe83\\x86\\x8e\\xc8': [-30, 2747079]}\n1  b'\\xe4\\xb3#\\xb5r\\x9c' bytearray(b'{\"topic\": \"/battery\", \"value\": 98.0}') {b'\\xe4\\xb3#\\xb5r\\x9c': [-22, 17023985], b'd\\xe83\\x86\\x8e\\xc8': [-30, 2747079]}\n1  b'\\xe4\\xb3#\\xb5r\\x9c' bytearray(b'{\"topic\": \"/battery\", \"value\": 98.0}') {b'\\xe4\\xb3#\\xb5r\\x9c': [-23, 17090096], b'd\\xe83\\x86\\x8e\\xc8': [-30, 2747079]}\n1  b'\\xe4\\xb3#\\xb5r\\x9c' bytearray(b'{\"topic\": \"/battery\", \"value\": 98.0}') {b'\\xe4\\xb3#\\xb5r\\x9c': [-23, 17156207], b'd\\xe83\\x86\\x8e\\xc8': [-30, 2747079]}\n1  b'\\xe4\\xb3#\\xb5r\\x9c' bytearray(b'{\"topic\": \"/battery\", \"value\": 98.0}') {b'\\xe4\\xb3#\\xb5r\\x9c': [-22, 17222320], b'd\\xe83\\x86\\x8e\\xc8': [-30, 2747079]}\n1  b'\\xe4\\xb3#\\xb5r\\x9c' bytearray(b'{\"topic\": \"/battery\", \"value\": 98.0}') {b'\\xe4\\xb3#\\xb5r\\x9c': [-23, 17288430], b'd\\xe83\\x86\\x8e\\xc8': [-30, 2747079]}\n1  b'\\xe4\\xb3#\\xb5r\\x9c' bytearray(b'{\"topic\": \"/battery\", \"value\": 98.0}') {b'\\xe4\\xb3#\\xb5r\\x9c': [-22, 17354541], b'd\\xe83\\x86\\x8e\\xc8': [-30, 2747079]}\n1  b'\\xe4\\xb3#\\xb5r\\x9c' bytearray(b'{\"topic\": \"/battery\", \"value\": 98.0}') {b'\\xe4\\xb3#\\xb5r\\x9c': [-23, 17420653], b'd\\xe83\\x86\\x8e\\xc8': [-30, 2747079]}\n1  b'\\xe4\\xb3#\\xb5r\\x9c' bytearray(b'{\"topic\": \"/battery\", \"value\": 98.0}') {b'\\xe4\\xb3#\\xb5r\\x9c': [-23, 17486764], b'd\\xe83\\x86\\x8e\\xc8': [-30, 2747079]}\n1  b'\\xe4\\xb3#\\xb5r\\x9c' bytearray(b'{\"topic\": \"/battery\", \"value\": 98.0}') {b'\\xe4\\xb3#\\xb5r\\x9c': [-23, 17552876], b'd\\xe83\\x86\\x8e\\xc8': [-30, 2747079]}\n1  b'\\xe4\\xb3#\\xb5r\\x9c' bytearray(b'{\"topic\": \"/battery\", \"value\": 98.0}') {b'\\xe4\\xb3#\\xb5r\\x9c': [-22, 17618988], b'd\\xe83\\x86\\x8e\\xc8': [-30, 2747079]}"
  out "XY Graph 3":cluster{"X":dbl, "Y":dbl}[](graph)=[{"X"=0.0, "Y"=94.5}, {"X"=0.10398083333333334, "Y"=94.5}, {"X"=0.1407091666666667, "Y"=93.9}, {"X"=0.1407091666666667, "Y"=93.9}, {"X"=0.19580222222222224, "Y"=92.8}, {"X"=0.19580222222222224, "Y"=92.8}, {"X"=0.2692627777777778, "Y"=91.4}, {"X"=0.2692627777777778, "Y"=91.4}, {"X"=0.2876261111111111, "Y"=91.1}, {"X"=0.2876261111111111, "Y"=91.1}, {"X"=0.3427222222222222, "Y"=90.0}, {"X"=0.3427222222222222, "Y"=90.0}, {"X"=0.3610888888888889, "Y"=89.7}, {"X"=0.39672972222222225, "Y"=89.7}, {"X"=0.43454666666666664, "Y"=88.4}, {"X"=0.39672972222222225, "Y"=88.0}, {"X"=0.5080036111111111, "Y"=87.1}, {"X"=0.5263672222222222, "Y"=86.8}, {"X"=0.39672972222222225, "Y"=86.5}, {"X"=0.7100141666666667, "Y"=83.8}, {"X"=0.72838, "Y"=83.5}, {"X"=0.7467447222222222, "Y"=83.2}, {"X"=0.7651083333333334, "Y"=82.9}, {"X"=0.7834727777777778, "Y"=82.6}, {"X"=0.8018372222222222, "Y"=82.3}, {"X"=0.8202013888888888, "Y"=82.0}, {"X"=0.8385661111111112, "Y"=81.7}, {"X"=0.8569297222222223, "Y"=81.4}, {"X"=0.8752952777777777, "Y"=81.1}, {"X"=0.8936611111111111, "Y"=80.8}, {"X"=0.9120252777777778, "Y"=80.6}, {"X"=0.930391388888889, "Y"=80.2}, {"X"=0.9487594444444445, "Y"=79.9}, {"X"=0.9671238888888889, "Y"=79.6}, {"X"=0.9854880555555555, "Y"=79.3}, {"X"=1.0038522222222221, "Y"=79.0}, {"X"=1.0222169444444444, "Y"=78.7}, {"X"=1.0405811111111112, "Y"=78.4}, {"X"=1.1324033333333332, "Y"=78.1}, {"X"=1.1507691666666666, "Y"=76.5}, {"X"=1.1691336111111112, "Y"=76.1}, {"X"=1.1874991666666666, "Y"=75.8}, {"X"=1.2058649999999997, "Y"=75.5}, {"X"=1.2242291666666667, "Y"=75.1}, {"X"=1.2425936111111113, "Y"=74.8}, {"X"=1.26096, "Y"=74.4}, {"X"=1.279325277777778, "Y"=74.1}, {"X"=1.2976897222222223, "Y"=73.8}, {"X"=1.3160533333333333, "Y"=73.4}, {"X"=1.3344180555555556, "Y"=73.1}, {"X"=1.3527819444444444, "Y"=72.7}, {"X"=1.3711466666666667, "Y"=72.4}, {"X"=1.3895105555555558, "Y"=72.0}, {"X"=1.407874722222222, "Y"=71.7}, {"X"=1.4262388888888888, "Y"=71.3}, {"X"=1.4446030555555553, "Y"=71.0}, {"X"=1.4629680555555558, "Y"=70.6}, {"X"=1.4813316666666665, "Y"=70.3}, {"X"=1.4996961111111111, "Y"=69.9}, {"X"=1.5180602777777776, "Y"=69.6}, {"X"=1.5731530555555553, "Y"=68.6}, {"X"=1.5915175, "Y"=68.2}, {"X"=1.6098816666666667, "Y"=67.9}, {"X"=1.6282458333333336, "Y"=67.5}, {"X"=1.6466105555555555, "Y"=67.2}, {"X"=1.6649747222222222, "Y"=66.8}, {"X"=1.6833388888888892, "Y"=66.5}, {"X"=1.7017030555555557, "Y"=66.2}, {"X"=1.7200672222222224, "Y"=65.8}, {"X"=1.7384319444444443, "Y"=65.5}, {"X"=1.756796388888889, "Y"=65.1}, {"X"=1.77516, "Y"=64.7}, {"X"=1.7935244444444445, "Y"=64.4}, {"X"=1.8118886111111112, "Y"=64.0}, {"X"=1.8302530555555556, "Y"=63.7}, {"X"=1.8486172222222224, "Y"=63.3}, {"X"=1.8669830555555555, "Y"=63.0}, {"X"=1.8853486111111113, "Y"=62.6}, {"X"=1.9037127777777778, "Y"=62.3}, {"X"=1.9220772222222222, "Y"=61.9}, {"X"=1.9771697222222222, "Y"=60.8}, {"X"=2.013898333333333, "Y"=60.4}, {"X"=2.032262777777778, "Y"=59.7}, {"X"=2.0506269444444443, "Y"=59.3}, {"X"=2.068991666666667, "Y"=58.9}, {"X"=2.0873555555555554, "Y"=58.5}, {"X"=2.1057197222222226, "Y"=58.1}, {"X"=2.124083888888889, "Y"=57.7}, {"X"=2.1424491666666667, "Y"=57.3}, {"X"=2.1791769444444444, "Y"=56.4}, {"X"=2.1791769444444444, "Y"=56.4}, {"X"=2.1975433333333334, "Y"=56.0}, {"X"=2.2342725000000003, "Y"=55.1}, {"X"=2.2342725000000003, "Y"=55.1}, {"X"=2.2526369444444447, "Y"=54.7}, {"X"=2.271001111111111, "Y"=54.2}, {"X"=2.2893652777777778, "Y"=53.7}, {"X"=2.3077294444444445, "Y"=53.3}, {"X"=2.326093888888889, "Y"=52.8}, {"X"=2.3444583333333333, "Y"=52.3}, {"X"=2.3444583333333333, "Y"=52.3}, {"X"=2.3628225, "Y"=51.8}, {"X"=2.3628225, "Y"=51.8}, {"X"=2.381186944444444, "Y"=51.3}, {"X"=2.3995511111111107, "Y"=50.8}, {"X"=2.417915555555555, "Y"=50.3}, {"X"=2.4362802777777777, "Y"=49.8}, {"X"=2.4362802777777777, "Y"=49.8}, {"X"=2.454644722222222, "Y"=49.3}, {"X"=2.4730080555555554, "Y"=48.7}, {"X"=2.4913722222222225, "Y"=48.2}, {"X"=2.509737777777778, "Y"=47.6}, {"X"=2.5281047222222224, "Y"=47.1}, {"X"=2.5281047222222224, "Y"=47.1}, {"X"=2.5648355555555553, "Y"=45.9}, {"X"=2.5648355555555553, "Y"=45.9}, {"X"=2.5831994444444444, "Y"=45.3}, {"X"=2.601563888888889, "Y"=44.7}, {"X"=2.6199280555555555, "Y"=44.1}, {"X"=2.6566566666666662, "Y"=42.9}, {"X"=2.6933849999999997, "Y"=41.7}, {"X"=2.7117491666666664, "Y"=41.0}, {"X"=2.730113611111111, "Y"=40.4}, {"X"=2.748478055555556, "Y"=39.8}, {"X"=2.803571388888889, "Y"=37.8}, {"X"=2.803571388888889, "Y"=37.8}, {"X"=2.8219374999999998, "Y"=37.2}, {"X"=2.8219374999999998, "Y"=37.2}, {"X"=2.8403016666666665, "Y"=36.5}, {"X"=2.8586661111111114, "Y"=35.9}, {"X"=2.8770302777777776, "Y"=35.2}, {"X"=2.8953944444444444, "Y"=34.5}, {"X"=2.8953944444444444, "Y"=34.5}, {"X"=2.9137588888888883, "Y"=33.8}, {"X"=2.9137588888888883, "Y"=33.8}, {"X"=2.9321233333333336, "Y"=33.1}, {"X"=2.9504875, "Y"=32.4}, {"X"=2.9688516666666667, "Y"=31.8}, {"X"=2.9872158333333334, "Y"=31.1}, {"X"=3.0606730555555557, "Y"=28.4}, {"X"=3.0606730555555557, "Y"=28.4}, {"X"=3.0790374999999996, "Y"=27.7}, {"X"=3.0790374999999996, "Y"=27.7}, {"X"=3.097401388888889, "Y"=27.1}, {"X"=3.115765833333333, "Y"=26.4}, {"X"=3.115765833333333, "Y"=26.4}, {"X"=3.134130555555556, "Y"=25.7}, {"X"=3.134130555555556, "Y"=25.7}, {"X"=3.1524947222222224, "Y"=25.1}, {"X"=3.1708586111111114, "Y"=24.5}, {"X"=3.1892230555555554, "Y"=23.8}, {"X"=3.207587777777778, "Y"=23.2}, {"X"=3.2259519444444447, "Y"=22.5}, {"X"=3.2259519444444447, "Y"=22.5}, {"X"=3.2443161111111114, "Y"=21.9}, {"X"=3.26268, "Y"=21.3}, {"X"=3.2810441666666668, "Y"=20.7}, {"X"=3.2810441666666668, "Y"=20.7}, {"X"=3.2994086111111107, "Y"=20.1}, {"X"=3.3177727777777775, "Y"=19.5}, {"X"=3.336137222222222, "Y"=18.8}, {"X"=3.354501388888889, "Y"=18.3}, {"X"=3.354501388888889, "Y"=18.3}, {"X"=3.372865555555556, "Y"=17.7}, {"X"=3.391230277777778, "Y"=17.1}, {"X"=3.409594166666667, "Y"=16.5}, {"X"=3.409594166666667, "Y"=16.5}, {"X"=3.446322777777778, "Y"=15.4}, {"X"=3.446322777777778, "Y"=15.4}, {"X"=3.4646869444444444, "Y"=14.9}, {"X"=3.483051388888889, "Y"=14.3}, {"X"=3.5014161111111113, "Y"=13.8}, {"X"=3.519780277777778, "Y"=13.3}, {"X"=3.5565083333333334, "Y"=12.3}, {"X"=3.593237222222222, "Y"=11.3}, {"X"=3.6116011111111113, "Y"=10.8}, {"X"=3.6299655555555557, "Y"=10.3}, {"X"=3.6483325, "Y"=9.9}, {"X"=3.6483325, "Y"=9.9}, {"X"=3.685061111111111, "Y"=8.9}, {"X"=3.703425277777778, "Y"=8.5}, {"X"=3.721789722222222, "Y"=8.0}, {"X"=3.8136136111111107, "Y"=5.9}, {"X"=3.831978055555555, "Y"=5.6}, {"X"=3.8503422222222223, "Y"=5.3}, {"X"=3.8687066666666667, "Y"=4.9}, {"X"=3.8687066666666667, "Y"=4.9}, {"X"=3.8870708333333335, "Y"=4.8}, {"X"=3.8870708333333335, "Y"=4.8}, {"X"=3.905435, "Y"=4.6}, {"X"=3.905435, "Y"=4.6}, {"X"=3.923799444444444, "Y"=4.4}, {"X"=3.9421636111111114, "Y"=4.2}, {"X"=3.9605280555555558, "Y"=4.0}, {"X"=4.015623611111112, "Y"=3.9}, {"X"=4.033988055555556, "Y"=3.9}, {"X"=4.033988055555556, "Y"=3.9}, {"X"=4.052351944444444, "Y"=3.9}, {"X"=4.052351944444444, "Y"=3.9}, {"X"=4.0707175, "Y"=3.9}, {"X"=4.089083333333333, "Y"=3.9}, {"X"=4.107447777777778, "Y"=3.9}, {"X"=4.125812777777778, "Y"=3.9}, {"X"=4.144176388888889, "Y"=3.9}, {"X"=4.162540555555556, "Y"=3.8}, {"X"=4.162540555555556, "Y"=3.8}, {"X"=4.199269722222222, "Y"=3.7}, {"X"=4.217633333333334, "Y"=3.6}, {"X"=4.2359975, "Y"=3.6}, {"X"=4.254361944444445, "Y"=3.5}, {"X"=4.272726388888889, "Y"=3.4}, {"X"=4.272726388888889, "Y"=3.4}, {"X"=4.291090555555556, "Y"=3.3}, {"X"=4.309455, "Y"=3.2}, {"X"=4.327818888888888, "Y"=3.1}, {"X"=4.3645475, "Y"=2.9}, {"X"=4.3645475, "Y"=2.9}, {"X"=4.382912500000001, "Y"=2.9}, {"X"=4.401276388888888, "Y"=2.9}, {"X"=4.419640277777778, "Y"=3.0}, {"X"=4.438004444444445, "Y"=2.9}, {"X"=4.474733333333334, "Y"=2.9}, {"X"=4.493100277777779, "Y"=2.9}, {"X"=4.511464722222223, "Y"=2.9}, {"X"=4.529828888888889, "Y"=3.0}, {"X"=4.548193055555556, "Y"=2.9}, {"X"=4.5665572222222215, "Y"=3.0}, {"X"=4.603288611111111, "Y"=2.9}, {"X"=4.621653055555556, "Y"=3.0}, {"X"=4.676746111111111, "Y"=2.9}, {"X"=4.695110000000001, "Y"=2.9}, {"X"=4.695110000000001, "Y"=2.9}, {"X"=4.7134744444444445, "Y"=2.9}, {"X"=4.7134744444444445, "Y"=2.9}, {"X"=4.7318388888888885, "Y"=2.9}, {"X"=4.7318388888888885, "Y"=2.9}, {"X"=4.7685699999999995, "Y"=2.8}, {"X"=4.786936944444445, "Y"=2.7}, {"X"=4.786936944444445, "Y"=2.7}, {"X"=4.805301944444444, "Y"=2.7}, {"X"=4.805301944444444, "Y"=2.7}, {"X"=4.823665555555555, "Y"=2.6}, {"X"=5.007289722222222, "Y"=2.6}, {"X"=5.025673333333333, "Y"=1.9}, {"X"=5.227670277777778, "Y"=1.9}, {"X"=5.24604388888889, "Y"=1.9}, {"X"=5.264408055555555, "Y"=1.9}, {"X"=5.282772499999999, "Y"=1.9}, {"X"=5.282772499999999, "Y"=1.9}, {"X"=5.301136666666666, "Y"=1.9}, {"X"=5.319500833333334, "Y"=1.9}, {"X"=5.3378652777777775, "Y"=1.9}, {"X"=5.411322222222222, "Y"=1.1}, {"X"=5.448050833333334, "Y"=0.9}, {"X"=5.448050833333334, "Y"=0.9}, {"X"=5.466415555555556, "Y"=0.8}, {"X"=5.48478, "Y"=0.6}, {"X"=5.503143611111111, "Y"=0.1}]
  in  "String 2":string="b'd\\xe83\\x86\\x8e\\xc8' bytearray(b'{\"topic\": \"/battery\", \"value\": 94.5}') {b'd\\xe83\\x86\\x8e\\xc8': [-42, 374312], b'\\xe4\\xb3#\\xb5r\\x9c': [-9, 374331]}\nb'\\xe4\\xb3#\\xb5r\\x9c' bytearray(b'{\"topic\": \"/battery\", \"value\": 94.5}') {b'd\\xe83\\x86\\x8e\\xc8': [-42, 374312], b'\\xe4\\xb3#\\xb5r\\x9c': [-9, 374331]}\nb'd\\xe83\\x86\\x8e\\xc8' bytearray(b'{\"topic\": \"/battery\", \"value\": 93.9}') {b'd\\xe83\\x86\\x8e\\xc8': [-42, 506477], b'\\xe4\\xb3#\\xb5r\\x9c': [-9, 506553]}\nb'\\xe4\\xb3#\\xb5r\\x9c' bytearray(b'{\"topic\": \"/battery\", \"value\": 93.9}') {b'd\\xe83\\x86\\x8e\\xc8': [-42, 506477], b'\\xe4\\xb3#\\xb5r\\x9c': [-9, 506553]}\nb'd\\xe83\\x86\\x8e\\xc8' bytearray(b'{\"topic\": \"/battery\", \"value\": 92.8}') {b'd\\xe83\\x86\\x8e\\xc8': [-40, 704830], b'\\xe4\\xb3#\\xb5r\\x9c': [-10, 704888]}\nb'\\xe4\\xb3#\\xb5r\\x9c' bytearray(b'{\"topic\": \"/battery\", \"value\": 92.8}') {b'd\\xe83\\x86\\x8e\\xc8': [-40, 704830], b'\\xe4\\xb3#\\xb5r\\x9c': [-10, 704888]}\nb'd\\xe83\\x86\\x8e\\xc8' bytearray(b'{\"topic\": \"/battery\", \"value\": 91.4}') {b'd\\xe83\\x86\\x8e\\xc8': [-40, 969265], b'\\xe4\\xb3#\\xb5r\\x9c': [-10, 969346]}\nb'\\xe4\\xb3#\\xb5r\\x9c' bytearray(b'{\"topic\": \"/battery\", \"value\": 91.4}') {b'd\\xe83\\x86\\x8e\\xc8': [-40, 969265], b'\\xe4\\xb3#\\xb5r\\x9c': [-10, 969346]}\nb'd\\xe83\\x86\\x8e\\xc8' bytearray(b'{\"topic\": \"/battery\", \"value\": 91.1}') {b'd\\xe83\\x86\\x8e\\xc8': [-40, 1035417], b'\\xe4\\xb3#\\xb5r\\x9c': [-10, 1035454]}\nb'\\xe4\\xb3#\\xb5r\\x9c' bytearray(b'{\"topic\": \"/battery\", \"value\": 91.1}') {b'd\\xe83\\x86\\x8e\\xc8': [-40, 1035417], b'\\xe4\\xb3#\\xb5r\\x9c': [-10, 1035454]}\nb'd\\xe83\\x86\\x8e\\xc8' bytearray(b'{\"topic\": \"/battery\", \"value\": 90.0}') {b'd\\xe83\\x86\\x8e\\xc8': [-40, 1233776], b'\\xe4\\xb3#\\xb5r\\x9c': [-10, 1233800]}\nb'\\xe4\\xb3#\\xb5r\\x9c' bytearray(b'{\"topic\": \"/battery\", \"value\": 90.0}') {b'd\\xe83\\x86\\x8e\\xc8': [-40, 1233776], b'\\xe4\\xb3#\\xb5r\\x9c': [-10, 1233800]}\nb'd\\xe83\\x86\\x8e\\xc8' bytearray(b'{\"topic\": \"/battery\", \"value\": 89.7}') {b'd\\xe83\\x86\\x8e\\xc8': [-40, 1299812], b'\\xe4\\xb3#\\xb5r\\x9c': [-10, 1299920]}\nb'\\xe4\\xb3#\\xb5r\\x9c' bytearray(b'{\"topic\": \"/battery\", \"value\": 89.7}') {b'd\\xe83\\x86\\x8e\\xc8': [-40, b'\\xe4\\xb3#\\xb5r\\x9c' bytearray(b'{\"topic\": \"/battery\", \"value\": 88.7}') {b'd\\xe83\\x86\\x8e\\xc8': [-40, 1428227], b'\\xe4\\xb3#\\xb5r\\x9c': [-10, 1498257]}\nb'\\xe4\\xb3#\\xb5r\\x9c' bytearray(b'{\"topic\": \"/battery\", \"value\": 88.4}') {b'd\\xe83\\x86\\x8e\\xc8': [-40, 1428227], b'\\xe4\\xb3#\\xb5r\\x9c': [-10, 1564368]}\nb'\\xe4\\xb3#\\xb5r\\x9c' bytearray(b'{\"topic\": \"/battery\", \"value\": 88.0}') {b'd\\xe83\\x86\\x8e\\xc8': [-40, ') {b'd\\xe83\\x86\\x8e\\xc8': [-40, 1428227], b'\\xe4\\xb3#\\xb5r\\x9c': [-10, 1762700]}\nb'\\xe4\\xb3#\\xb5r\\x9c' bytearray(b'{\"topic\": \"/battery\", \"value\": 87.1}') {b'd\\xe83\\x86\\x8e\\xc8': [-40, 1428227], b'\\xe4\\xb3#\\xb5r\\x9c': [-10, 1828813]}\nb'\\xe4\\xb3#\\xb5r\\x9c' bytearray(b'{\"topic\": \"/battery\", \"value\": 86.8}') {b'd\\xe83\\x86\\x8e\\xc8': [-40, 1428227], b'\\xe4\\xb3#\\xb5r\\x9c': [-10, 1894922]}\nb'\\xe4\\xb3#\\xb5r\\x9c' bytearray(b'{\"topic\": \"/battery\", \"value\": 86.5}') {b'd\\xe83\\x86\\x8e\\xc8': [-40, : 84.1}') {b'd\\xe83\\x86\\x8e\\xc8': [-40, 1428227], b'\\xe4\\xb3#\\xb5r\\x9c': [-10, 2489935]}\nb'\\xe4\\xb3#\\xb5r\\x9c' bytearray(b'{\"topic\": \"/battery\", \"value\": 83.8}') {b'd\\xe83\\x86\\x8e\\xc8': [-40, 1428227], b'\\xe4\\xb3#\\xb5r\\x9c': [-10, 2556051]}\nb'\\xe4\\xb3#\\xb5r\\x9c' bytearray(b'{\"topic\": \"/battery\", \"value\": 83.5}') {b'd\\xe83\\x86\\x8e\\xc8': [-40, 1428227], b'\\xe4\\xb3#\\xb5r\\x9c': [-10, 2622168]}\nb'\\xe4\\xb3#\\xb5r\\x9c' bytearray(b'{\"topic\": \"/battery\", \"value\": 83.2}') {b'd\\xe83\\x86\\x8e\\xc8': [-40, 1428227], b'\\xe4\\xb3#\\xb5r\\x9c': [-10, 2688281]}\nb'\\xe4\\xb3#\\xb5r\\x9c' bytearray(b'{\"topic\": \"/battery\", \"value\": 82.9}') {b'd\\xe83\\x86\\x8e\\xc8': [-40, 1428227], b'\\xe4\\xb3#\\xb5r\\x9c': [-10, 2754390]}\nb'\\xe4\\xb3#\\xb5r\\x9c' bytearray(b'{\"topic\": \"/battery\", \"value\": 82.6}') {b'd\\xe83\\x86\\x8e\\xc8': [-40, 1428227], b'\\xe4\\xb3#\\xb5r\\x9c': [-11, 2820502]}\nb'\\xe4\\xb3#\\xb5r\\x9c' bytearray(b'{\"topic\": \"/battery\", \"value\": 82.3}') {b'd\\xe83\\x86\\x8e\\xc8': [-40, 1428227], b'\\xe4\\xb3#\\xb5r\\x9c': [-46, 2886614]}\nb'\\xe4\\xb3#\\xb5r\\x9c' bytearray(b'{\"topic\": \"/battery\", \"value\": 82.0}') {b'd\\xe83\\x86\\x8e\\xc8': [-40, 1428227], b'\\xe4\\xb3#\\xb5r\\x9c': [-55, 2952725]}\nb'\\xe4\\xb3#\\xb5r\\x9c' bytearray(b'{\"topic\": \"/battery\", \"value\": 81.7}') {b'd\\xe83\\x86\\x8e\\xc8': [-40, 1428227], b'\\xe4\\xb3#\\xb5r\\x9c': [-45, 3018838]}\nb'\\xe4\\xb3#\\xb5r\\x9c' bytearray(b'{\"topic\": \"/battery\", \"value\": 81.4}') {b'd\\xe83\\x86\\x8e\\xc8': [-40, 1428227], b'\\xe4\\xb3#\\xb5r\\x9c': [-45, 3084947]}\nb'\\xe4\\xb3#\\xb5r\\x9c' bytearray(b'{\"topic\": \"/battery\", \"value\": 81.1}') {b'd\\xe83\\x86\\x8e\\xc8': [-40, 1428227], b'\\xe4\\xb3#\\xb5r\\x9c': [-45, 3151063]}\nb'\\xe4\\xb3#\\xb5r\\x9c' bytearray(b'{\"topic\": \"/battery\", \"value\": 80.8}') {b'd\\xe83\\x86\\x8e\\xc8': [-40, 1428227], b'\\xe4\\xb3#\\xb5r\\x9c': [-45, 3217180]}\nb'\\xe4\\xb3#\\xb5r\\x9c' bytearray(b'{\"topic\": \"/battery\", \"value\": 80.6}') {b'd\\xe83\\x86\\x8e\\xc8': [-40, 1428227], b'\\xe4\\xb3#\\xb5r\\x9c': [-45, 3283291]}\nb'\\xe4\\xb3#\\xb5r\\x9c' bytearray(b'{\"topic\": \"/battery\", \"value\": 80.2}') {b'd\\xe83\\x86\\x8e\\xc8': [-40, 1428227], b'\\xe4\\xb3#\\xb5r\\x9c': [-44, 3349409]}\nb'\\xe4\\xb3#\\xb5r\\x9c' bytearray(b'{\"topic\": \"/battery\", \"value\": 79.9}') {b'd\\xe83\\x86\\x8e\\xc8': [-40, 1428227], b'\\xe4\\xb3#\\xb5r\\x9c': [-45, 3415534]}\nb'\\xe4\\xb3#\\xb5r\\x9c' bytearray(b'{\"topic\": \"/battery\", \"value\": 79.6}') {b'd\\xe83\\x86\\x8e\\xc8': [-40, 1428227], b'\\xe4\\xb3#\\xb5r\\x9c': [-45, 3481646]}\nb'\\xe4\\xb3#\\xb5r\\x9c' bytearray(b'{\"topic\": \"/battery\", \"value\": 79.3}') {b'd\\xe83\\x86\\x8e\\xc8': [-40, 1428227], b'\\xe4\\xb3#\\xb5r\\x9c': [-45, 3547757]}\nb'\\xe4\\xb3#\\xb5r\\x9c' bytearray(b'{\"topic\": \"/battery\", \"value\": 79.0}') {b'd\\xe83\\x86\\x8e\\xc8': [-40, 1428227], b'\\xe4\\xb3#\\xb5r\\x9c': [-45, 3613868]}\nb'\\xe4\\xb3#\\xb5r\\x9c' bytearray(b'{\"topic\": \"/battery\", \"value\": 78.7}') {b'd\\xe83\\x86\\x8e\\xc8': [-40, 1428227], b'\\xe4\\xb3#\\xb5r\\x9c': [-45, 3679981]}\nb'\\xe4\\xb3#\\xb5r\\x9c' bytearray(b'{\"topic\": \"/battery\", \"value\": 78.4}') {b'd\\xe83\\x86\\x8e\\xc8': [-40, 1428227], b'\\xe4\\xb3#\\xb5r\\x9c': [-45, 3746092]}\nb'\\xe4\\xb3#\\xb5r\\x9c' bytearray(b'{\"topic\": \"/battery\", \"value\": 78.1}') {b'd\\xe83\\x86\\x8e\\xc8': [-40, b3#\\xb5r\\x9c': [-44, 4076652]}\nb'\\xe4\\xb3#\\xb5r\\x9c' bytearray(b'{\"topic\": \"/battery\", \"value\": 76.5}') {b'd\\xe83\\x86\\x8e\\xc8': [-40, 1428227], b'\\xe4\\xb3#\\xb5r\\x9c': [-44, 4142769]}\nb'\\xe4\\xb3#\\xb5r\\x9c' bytearray(b'{\"topic\": \"/battery\", \"value\": 76.1}') {b'd\\xe83\\x86\\x8e\\xc8': [-40, 1428227], b'\\xe4\\xb3#\\xb5r\\x9c': [-45, 4208881]}\nb'\\xe4\\xb3#\\xb5r\\x9c' bytearray(b'{\"topic\": \"/battery\", \"value\": 75.8}') {b'd\\xe83\\x86\\x8e\\xc8': [-40, 1428227], b'\\xe4\\xb3#\\xb5r\\x9c': [-45, 4274997]}\nb'\\xe4\\xb3#\\xb5r\\x9c' bytearray(b'{\"topic\": \"/battery\", \"value\": 75.5}') {b'd\\xe83\\x86\\x8e\\xc8': [-40, 1428227], b'\\xe4\\xb3#\\xb5r\\x9c': [-45, 4341114]}\nb'\\xe4\\xb3#\\xb5r\\x9c' bytearray(b'{\"topic\": \"/battery\", \"value\": 75.1}') {b'd\\xe83\\x86\\x8e\\xc8': [-40, 1428227], b'\\xe4\\xb3#\\xb5r\\x9c': [-45, 4407225]}\nb'\\xe4\\xb3#\\xb5r\\x9c' bytearray(b'{\"topic\": \"/battery\", \"value\": 74.8}') {b'd\\xe83\\x86\\x8e\\xc8': [-40, 1428227], b'\\xe4\\xb3#\\xb5r\\x9c': [-44, 4473337]}\nb'\\xe4\\xb3#\\xb5r\\x9c' bytearray(b'{\"topic\": \"/battery\", \"value\": 74.4}') {b'd\\xe83\\x86\\x8e\\xc8': [-40, 1428227], b'\\xe4\\xb3#\\xb5r\\x9c': [-45, 4539456]}\nb'\\xe4\\xb3#\\xb5r\\x9c' bytearray(b'{\"topic\": \"/battery\", \"value\": 74.1}') {b'd\\xe83\\x86\\x8e\\xc8': [-40, 1428227], b'\\xe4\\xb3#\\xb5r\\x9c': [-45, 4605571]}\nb'\\xe4\\xb3#\\xb5r\\x9c' bytearray(b'{\"topic\": \"/battery\", \"value\": 73.8}') {b'd\\xe83\\x86\\x8e\\xc8': [-40, 1428227], b'\\xe4\\xb3#\\xb5r\\x9c': [-45, 4671683]}\nb'\\xe4\\xb3#\\xb5r\\x9c' bytearray(b'{\"topic\": \"/battery\", \"value\": 73.4}') {b'd\\xe83\\x86\\x8e\\xc8': [-40, 1428227], b'\\xe4\\xb3#\\xb5r\\x9c': [-44, 4737792]}\nb'\\xe4\\xb3#\\xb5r\\x9c' bytearray(b'{\"topic\": \"/battery\", \"value\": 73.1}') {b'd\\xe83\\x86\\x8e\\xc8': [-40, 1428227], b'\\xe4\\xb3#\\xb5r\\x9c': [-45, 4803905]}\nb'\\xe4\\xb3#\\xb5r\\x9c' bytearray(b'{\"topic\": \"/battery\", \"value\": 72.7}') {b'd\\xe83\\x86\\x8e\\xc8': [-40, 1428227], b'\\xe4\\xb3#\\xb5r\\x9c': [-45, 4870015]}\nb'\\xe4\\xb3#\\xb5r\\x9c' bytearray(b'{\"topic\": \"/battery\", \"value\": 72.4}') {b'd\\xe83\\x86\\x8e\\xc8': [-40, 1428227], b'\\xe4\\xb3#\\xb5r\\x9c': [-45, 4936128]}\nb'\\xe4\\xb3#\\xb5r\\x9c' bytearray(b'{\"topic\": \"/battery\", \"value\": 72.0}') {b'd\\xe83\\x86\\x8e\\xc8': [-40, 1428227], b'\\xe4\\xb3#\\xb5r\\x9c': [-45, 5002238]}\nb'\\xe4\\xb3#\\xb5r\\x9c' bytearray(b'{\"topic\": \"/battery\", \"value\": 71.7}') {b'd\\xe83\\x86\\x8e\\xc8': [-40, 1428227], b'\\xe4\\xb3#\\xb5r\\x9c': [-43, 5068349]}\nb'\\xe4\\xb3#\\xb5r\\x9c' bytearray(b'{\"topic\": \"/battery\", \"value\": 71.3}') {b'd\\xe83\\x86\\x8e\\xc8': [-40, 1428227], b'\\xe4\\xb3#\\xb5r\\x9c': [-44, 5134460]}\nb'\\xe4\\xb3#\\xb5r\\x9c' bytearray(b'{\"topic\": \"/battery\", \"value\": 71.0}') {b'd\\xe83\\x86\\x8e\\xc8': [-40, 1428227], b'\\xe4\\xb3#\\xb5r\\x9c': [-44, 5200571]}\nb'\\xe4\\xb3#\\xb5r\\x9c' bytearray(b'{\"topic\": \"/battery\", \"value\": 70.6}') {b'd\\xe83\\x86\\x8e\\xc8': [-40, 1428227], b'\\xe4\\xb3#\\xb5r\\x9c': [-44, 5266685]}\nb'\\xe4\\xb3#\\xb5r\\x9c' bytearray(b'{\"topic\": \"/battery\", \"value\": 70.3}') {b'd\\xe83\\x86\\x8e\\xc8': [-40, 1428227], b'\\xe4\\xb3#\\xb5r\\x9c': [-44, 5332794]}\nb'\\xe4\\xb3#\\xb5r\\x9c' bytearray(b'{\"topic\": \"/battery\", \"value\": 69.9}') {b'd\\xe83\\x86\\x8e\\xc8': [-40, 1428227], b'\\xe4\\xb3#\\xb5r\\x9c': [-44, 5398906]}\nb'\\xe4\\xb3#\\xb5r\\x9c' bytearray(b'{\"topic\": \"/battery\", \"value\": 69.6}') {b'd\\xe83\\x86\\x8e\\xc8': [-40, 1428227], b'\\xe4\\xb3#\\xb5r\\x9c': [-44, 5465017]}\nb'\\xe4\\xb3#\\xb5r\\x9c' bytearray(b'{\"topic\": \"/battery\", \"value\": 69.3}') {b'd\\xe83\\x86\\x8e\\xc8': [-40, b'\\xe4\\xb3#\\xb5r\\x9c' bytearray(b'{\"topic\": \"/battery\", \"value\": 68.9}') {b'd\\xe83\\x86\\x8e\\xc8': [-40, 1428227], b'\\xe4\\xb3#\\xb5r\\x9c': [-44, 5597242]}\nb'\\xe4\\xb3#\\xb5r\\x9c' bytearray(b'{\"topic\": \"/battery\", \"value\": 68.6}') {b'd\\xe83\\x86\\x8e\\xc8': [-40, 1428227], b'\\xe4\\xb3#\\xb5r\\x9c': [-44, 5663351]}\nb'\\xe4\\xb3#\\xb5r\\x9c' bytearray(b'{\"topic\": \"/battery\", \"value\": 68.2}') {b'd\\xe83\\x86\\x8e\\xc8': [-40, 1428227], b'\\xe4\\xb3#\\xb5r\\x9c': [-45, 5729463]}\nb'\\xe4\\xb3#\\xb5r\\x9c' bytearray(b'{\"topic\": \"/battery\", \"value\": 67.9}') {b'd\\xe83\\x86\\x8e\\xc8': [-40, 1428227], b'\\xe4\\xb3#\\xb5r\\x9c': [-44, 5795574]}\nb'\\xe4\\xb3#\\xb5r\\x9c' bytearray(b'{\"topic\": \"/battery\", \"value\": 67.5}') {b'd\\xe83\\x86\\x8e\\xc8': [-40, 1428227], b'\\xe4\\xb3#\\xb5r\\x9c': [-44, 5861685]}\nb'\\xe4\\xb3#\\xb5r\\x9c' bytearray(b'{\"topic\": \"/battery\", \"value\": 67.2}') {b'd\\xe83\\x86\\x8e\\xc8': [-40, 1428227], b'\\xe4\\xb3#\\xb5r\\x9c': [-44, 5927798]}\nb'\\xe4\\xb3#\\xb5r\\x9c' bytearray(b'{\"topic\": \"/battery\", \"value\": 66.8}') {b'd\\xe83\\x86\\x8e\\xc8': [-40, 1428227], b'\\xe4\\xb3#\\xb5r\\x9c': [-44, 5993909]}\nb'\\xe4\\xb3#\\xb5r\\x9c' bytearray(b'{\"topic\": \"/battery\", \"value\": 66.5}') {b'd\\xe83\\x86\\x8e\\xc8': [-40, 1428227], b'\\xe4\\xb3#\\xb5r\\x9c': [-44, 6060020]}\nb'\\xe4\\xb3#\\xb5r\\x9c' bytearray(b'{\"topic\": \"/battery\", \"value\": 66.2}') {b'd\\xe83\\x86\\x8e\\xc8': [-40, 1428227], b'\\xe4\\xb3#\\xb5r\\x9c': [-44, 6126131]}\nb'\\xe4\\xb3#\\xb5r\\x9c' bytearray(b'{\"topic\": \"/battery\", \"value\": 65.8}') {b'd\\xe83\\x86\\x8e\\xc8': [-40, 1428227], b'\\xe4\\xb3#\\xb5r\\x9c': [-44, 6192242]}\nb'\\xe4\\xb3#\\xb5r\\x9c' bytearray(b'{\"topic\": \"/battery\", \"value\": 65.5}') {b'd\\xe83\\x86\\x8e\\xc8': [-40, 1428227], b'\\xe4\\xb3#\\xb5r\\x9c': [-44, 6258355]}\nb'\\xe4\\xb3#\\xb5r\\x9c' bytearray(b'{\"topic\": \"/battery\", \"value\": 65.1}') {b'd\\xe83\\x86\\x8e\\xc8': [-40, 1428227], b'\\xe4\\xb3#\\xb5r\\x9c': [-44, 6324467]}\nb'\\xe4\\xb3#\\xb5r\\x9c' bytearray(b'{\"topic\": \"/battery\", \"value\": 64.7}') {b'd\\xe83\\x86\\x8e\\xc8': [-40, 1428227], b'\\xe4\\xb3#\\xb5r\\x9c': [-44, 6390576]}\nb'\\xe4\\xb3#\\xb5r\\x9c' bytearray(b'{\"topic\": \"/battery\", \"value\": 64.4}') {b'd\\xe83\\x86\\x8e\\xc8': [-40, 1428227], b'\\xe4\\xb3#\\xb5r\\x9c': [-43, 6456688]}\nb'\\xe4\\xb3#\\xb5r\\x9c' bytearray(b'{\"topic\": \"/battery\", \"value\": 64.0}') {b'd\\xe83\\x86\\x8e\\xc8': [-40, 1428227], b'\\xe4\\xb3#\\xb5r\\x9c': [-44, 6522799]}\nb'\\xe4\\xb3#\\xb5r\\x9c' bytearray(b'{\"topic\": \"/battery\", \"value\": 63.7}') {b'd\\xe83\\x86\\x8e\\xc8': [-40, 1428227], b'\\xe4\\xb3#\\xb5r\\x9c': [-44, 6588911]}\nb'\\xe4\\xb3#\\xb5r\\x9c' bytearray(b'{\"topic\": \"/battery\", \"value\": 63.3}') {b'd\\xe83\\x86\\x8e\\xc8': [-40, 1428227], b'\\xe4\\xb3#\\xb5r\\x9c': [-44, 6655022]}\nb'\\xe4\\xb3#\\xb5r\\x9c' bytearray(b'{\"topic\": \"/battery\", \"value\": 63.0}') {b'd\\xe83\\x86\\x8e\\xc8': [-40, 1428227], b'\\xe4\\xb3#\\xb5r\\x9c': [-44, 6721139]}\nb'\\xe4\\xb3#\\xb5r\\x9c' bytearray(b'{\"topic\": \"/battery\", \"value\": 62.6}') {b'd\\xe83\\x86\\x8e\\xc8': [-40, 1428227], b'\\xe4\\xb3#\\xb5r\\x9c': [-45, 6787255]}\nb'\\xe4\\xb3#\\xb5r\\x9c' bytearray(b'{\"topic\": \"/battery\", \"value\": 62.3}') {b'd\\xe83\\x86\\x8e\\xc8': [-40, 1428227], b'\\xe4\\xb3#\\xb5r\\x9c': [-45, 6853366]}\nb'\\xe4\\xb3#\\xb5r\\x9c' bytearray(b'{\"topic\": \"/battery\", \"value\": 61.9}') {b'd\\xe83\\x86\\x8e\\xc8': [-40, 1428227], b'\\xe4\\xb3#\\xb5r\\x9c': [-44, 6919478]}\nb'\\xe4\\xb3#\\xb5r\\x9c' bytearray(b'{\"topic\": \"/battery\", \"value\": 61.5}') {b'd\\xe83\\x86\\x8e\\xc8': [-40, b'\\xe4\\xb3#\\xb5r\\x9c' bytearray(b'{\"topic\": \"/battery\", \"value\": 61.2}') {b'd\\xe83\\x86\\x8e\\xc8': [-40, 1428227], b'\\xe4\\xb3#\\xb5r\\x9c': [-44, 7051703]}\nb'\\xe4\\xb3#\\xb5r\\x9c' bytearray(b'{\"topic\": \"/battery\", \"value\": 60.8}') {b'd\\xe83\\x86\\x8e\\xc8': [-40, 1428227], b'\\xe4\\xb3#\\xb5r\\x9c': [-44, 7117811]}\nb'\\xe4\\xb3#\\xb5r\\x9c' bytearray(b'{\"topic\": \"/battery\", \"value\": 60.4}') {b'd\\xe83\\x86\\x8e\\xc8': [-40, b3#\\xb5r\\x9c': [-44, 7250034]}\nb'\\xe4\\xb3#\\xb5r\\x9c' bytearray(b'{\"topic\": \"/battery\", \"value\": 59.7}') {b'd\\xe83\\x86\\x8e\\xc8': [-40, 1428227], b'\\xe4\\xb3#\\xb5r\\x9c': [-44, 7316146]}\nb'\\xe4\\xb3#\\xb5r\\x9c' bytearray(b'{\"topic\": \"/battery\", \"value\": 59.3}') {b'd\\xe83\\x86\\x8e\\xc8': [-40, 1428227], b'\\xe4\\xb3#\\xb5r\\x9c': [-44, 7382257]}\nb'\\xe4\\xb3#\\xb5r\\x9c' bytearray(b'{\"topic\": \"/battery\", \"value\": 58.9}') {b'd\\xe83\\x86\\x8e\\xc8': [-40, 1428227], b'\\xe4\\xb3#\\xb5r\\x9c': [-44, 7448370]}\nb'\\xe4\\xb3#\\xb5r\\x9c' bytearray(b'{\"topic\": \"/battery\", \"value\": 58.5}') {b'd\\xe83\\x86\\x8e\\xc8': [-40, 1428227], b'\\xe4\\xb3#\\xb5r\\x9c': [-44, 7514480]}\nb'\\xe4\\xb3#\\xb5r\\x9c' bytearray(b'{\"topic\": \"/battery\", \"value\": 58.1}') {b'd\\xe83\\x86\\x8e\\xc8': [-40, 1428227], b'\\xe4\\xb3#\\xb5r\\x9c': [-43, 7580591]}\nb'\\xe4\\xb3#\\xb5r\\x9c' bytearray(b'{\"topic\": \"/battery\", \"value\": 57.7}') {b'd\\xe83\\x86\\x8e\\xc8': [-40, 1428227], b'\\xe4\\xb3#\\xb5r\\x9c': [-53, 7646702]}\nb'\\xe4\\xb3#\\xb5r\\x9c' bytearray(b'{\"topic\": \"/battery\", \"value\": 57.3}') {b'd\\xe83\\x86\\x8e\\xc8': [-40, 1428227], b'\\xe4\\xb3#\\xb5r\\x9c': [-51, 7712817]}\nb'd\\xe83\\x86\\x8e\\xc8' bytearray(b'{\"topic\": \"/gem\", \"value\": \"ZOgzho7I\\\\n\"}') {b'd\\xe83\\x86\\x8e\\xc8': [-45, 7831506], b'\\xe4\\xb3#\\xb5r\\x9c': [-51, 7778925]}\nb'd\\xe83\\x86\\x8e\\xc8' bytearray(b'{\"topic\": \"/game\", \"value\": 2}') {b'd\\xe83\\x86\\x8e\\xc8': [-38, 7832009], b'\\xe4\\xb3#\\xb5r\\x9c': [-51, 7778925]}\nb'd\\xe83\\x86\\x8e\\xc8' bytearray(b'{\"topic\": \"/battery\", \"value\": 56.4}') {b'd\\xe83\\x86\\x8e\\xc8': [-25, 7844975], b'\\xe4\\xb3#\\xb5r\\x9c': [-43, 7845037]}\nb'\\xe4\\xb3#\\xb5r\\x9c' bytearray(b'{\"topic\": \"/battery\", \"value\": 56.4}') {b'd\\xe83\\x86\\x8e\\xc8': [-25, 7844975], b'\\xe4\\xb3#\\xb5r\\x9c': [-43, 7845037]}\nb'\\xe4\\xb3#\\xb5r\\x9c' bytearray(b'{\"topic\": \"/battery\", \"value\": 56.0}') {b'd\\xe83\\x86\\x8e\\xc8': [-25, 7911113], b'\\xe4\\xb3#\\xb5r\\x9c': [-44, 7911156]}\nb'd\\xe83\\x86\\x8e\\xc8' bytearray(b'{\"topic\": \"/battery\", \"value\": 55.1}') {b'd\\xe83\\x86\\x8e\\xc8': [-25, 8043380], b'\\xe4\\xb3#\\xb5r\\x9c': [-44, 8043381]}\nb'\\xe4\\xb3#\\xb5r\\x9c' bytearray(b'{\"topic\": \"/battery\", \"value\": 55.1}') {b'd\\xe83\\x86\\x8e\\xc8': [-25, 8043380], b'\\xe4\\xb3#\\xb5r\\x9c': [-44, 8043381]}\nb'\\xe4\\xb3#\\xb5r\\x9c' bytearray(b'{\"topic\": \"/battery\", \"value\": 54.7}') {b'd\\xe83\\x86\\x8e\\xc8': [-26, 8109362], b'\\xe4\\xb3#\\xb5r\\x9c': [-43, 8109493]}\nb'\\xe4\\xb3#\\xb5r\\x9c' bytearray(b'{\"topic\": \"/battery\", \"value\": 54.2}') {b'd\\xe83\\x86\\x8e\\xc8': [-26, 8175580], b'\\xe4\\xb3#\\xb5r\\x9c': [-43, 8175604]}\nb'\\xe4\\xb3#\\xb5r\\x9c' bytearray(b'{\"topic\": \"/battery\", \"value\": 53.7}') {b'd\\xe83\\x86\\x8e\\xc8': [-25, 8241682], b'\\xe4\\xb3#\\xb5r\\x9c': [-49, 8241715]}\nb'\\xe4\\xb3#\\xb5r\\x9c' bytearray(b'{\"topic\": \"/battery\", \"value\": 53.3}') {b'd\\xe83\\x86\\x8e\\xc8': [-25, 8307791], b'\\xe4\\xb3#\\xb5r\\x9c': [-48, 8307826]}\nb'\\xe4\\xb3#\\xb5r\\x9c' bytearray(b'{\"topic\": \"/battery\", \"value\": 52.8}') {b'd\\xe83\\x86\\x8e\\xc8': [-25, 8373812], b'\\xe4\\xb3#\\xb5r\\x9c': [-48, 8373938]}\nb'd\\xe83\\x86\\x8e\\xc8' bytearray(b'{\"topic\": \"/battery\", \"value\": 52.3}') {b'd\\xe83\\x86\\x8e\\xc8': [-26, 8439985], b'\\xe4\\xb3#\\xb5r\\x9c': [-49, 8440050]}\nb'\\xe4\\xb3#\\xb5r\\x9c' bytearray(b'{\"topic\": \"/battery\", \"value\": 52.3}') {b'd\\xe83\\x86\\x8e\\xc8': [-26, 8439985], b'\\xe4\\xb3#\\xb5r\\x9c': [-49, 8440050]}\nb'd\\xe83\\x86\\x8e\\xc8' bytearray(b'{\"topic\": \"/battery\", \"value\": 51.8}') {b'd\\xe83\\x86\\x8e\\xc8': [-26, 8506069], b'\\xe4\\xb3#\\xb5r\\x9c': [-51, 8506161]}\nb'\\xe4\\xb3#\\xb5r\\x9c' bytearray(b'{\"topic\": \"/battery\", \"value\": 51.8}') {b'd\\xe83\\x86\\x8e\\xc8': [-26, 8506069], b'\\xe4\\xb3#\\xb5r\\x9c': [-51, 8506161]}\nb'\\xe4\\xb3#\\xb5r\\x9c' bytearray(b'{\"topic\": \"/battery\", \"value\": 51.3}') {b'd\\xe83\\x86\\x8e\\xc8': [-26, 8572167], b'\\xe4\\xb3#\\xb5r\\x9c': [-50, 8572273]}\nb'\\xe4\\xb3#\\xb5r\\x9c' bytearray(b'{\"topic\": \"/battery\", \"value\": 50.8}') {b'd\\xe83\\x86\\x8e\\xc8': [-26, 8638298], b'\\xe4\\xb3#\\xb5r\\x9c': [-54, 8638384]}\nb'\\xe4\\xb3#\\xb5r\\x9c' bytearray(b'{\"topic\": \"/battery\", \"value\": 50.3}') {b'd\\xe83\\x86\\x8e\\xc8': [-25, 8704439], b'\\xe4\\xb3#\\xb5r\\x9c': [-51, 8704496]}\nb'd\\xe83\\x86\\x8e\\xc8' bytearray(b'{\"topic\": \"/battery\", \"value\": 49.8}') {b'd\\xe83\\x86\\x8e\\xc8': [-25, 8770545], b'\\xe4\\xb3#\\xb5r\\x9c': [-49, 8770609]}\nb'\\xe4\\xb3#\\xb5r\\x9c' bytearray(b'{\"topic\": \"/battery\", \"value\": 49.8}') {b'd\\xe83\\x86\\x8e\\xc8': [-25, 8770545], b'\\xe4\\xb3#\\xb5r\\x9c': [-49, 8770609]}\nb'\\xe4\\xb3#\\xb5r\\x9c' bytearray(b'{\"topic\": \"/battery\", \"value\": 49.3}') {b'd\\xe83\\x86\\x8e\\xc8': [-25, 8836711], b'\\xe4\\xb3#\\xb5r\\x9c': [-47, 8836721]}\nb'\\xe4\\xb3#\\xb5r\\x9c' bytearray(b'{\"topic\": \"/battery\", \"value\": 48.7}') {b'd\\xe83\\x86\\x8e\\xc8': [-25, 8902774], b'\\xe4\\xb3#\\xb5r\\x9c': [-49, 8902829]}\nb'\\xe4\\xb3#\\xb5r\\x9c' bytearray(b'{\"topic\": \"/battery\", \"value\": 48.2}') {b'd\\xe83\\x86\\x8e\\xc8': [-26, 8968889], b'\\xe4\\xb3#\\xb5r\\x9c': [-47, 8968940]}\nb'\\xe4\\xb3#\\xb5r\\x9c' bytearray(b'{\"topic\": \"/battery\", \"value\": 47.6}') {b'd\\xe83\\x86\\x8e\\xc8': [-26, 9034964], b'\\xe4\\xb3#\\xb5r\\x9c': [-45, 9035056]}\nb'd\\xe83\\x86\\x8e\\xc8' bytearray(b'{\"topic\": \"/battery\", \"value\": 47.1}') {b'd\\xe83\\x86\\x8e\\xc8': [-26, 9101060], b'\\xe4\\xb3#\\xb5r\\x9c': [-46, 9101177]}\nb'\\xe4\\xb3#\\xb5r\\x9c' bytearray(b'{\"topic\": \"/battery\", \"value\": 47.1}') {b'd\\xe83\\x86\\x8e\\xc8': [-26, 9101060], b'\\xe4\\xb3#\\xb5r\\x9c': [-46, 9101177]}\nb'd\\xe83\\x86\\x8e\\xc8' bytearray(b'{\"topic\": \"/battery\", \"value\": 45.9}') {b'd\\xe83\\x86\\x8e\\xc8': [-26, 9233395], b'\\xe4\\xb3#\\xb5r\\x9c': [-49, 9233408]}\nb'\\xe4\\xb3#\\xb5r\\x9c' bytearray(b'{\"topic\": \"/battery\", \"value\": 45.9}') {b'd\\xe83\\x86\\x8e\\xc8': [-26, 9233395], b'\\xe4\\xb3#\\xb5r\\x9c': [-49, 9233408]}\nb'\\xe4\\xb3#\\xb5r\\x9c' bytearray(b'{\"topic\": \"/battery\", \"value\": 45.3}') {b'd\\xe83\\x86\\x8e\\xc8': [-26, 9299417], b'\\xe4\\xb3#\\xb5r\\x9c': [-43, 9299518]}\nb'\\xe4\\xb3#\\xb5r\\x9c' bytearray(b'{\"topic\": \"/battery\", \"value\": 44.7}') {b'd\\xe83\\x86\\x8e\\xc8': [-26, 9365516], b'\\xe4\\xb3#\\xb5r\\x9c': [-47, 9365630]}\nb'\\xe4\\xb3#\\xb5r\\x9c' bytearray(b'{\"topic\": \"/battery\", \"value\": 44.1}') {b'd\\xe83\\x86\\x8e\\xc8': [-26, 9431708], b'\\xe4\\xb3#\\xb5r\\x9c': [-47, 9431741]}\nb'\\xe4\\xb3#\\xb5r\\x9c' bytearray(b'{\"topic\": \"/battery\", \"value\": 42.9}') {b'd\\xe83\\x86\\x8e\\xc8': [-26, 9563840], b'\\xe4\\xb3#\\xb5r\\x9c': [-47, 9563964]}\nb'\\xe4\\xb3#\\xb5r\\x9c' bytearray(b'{\"topic\": \"/battery\", \"value\": 41.7}') {b'd\\xe83\\x86\\x8e\\xc8': [-26, 9696182], b'\\xe4\\xb3#\\xb5r\\x9c': [-49, 9696186]}\nb'\\xe4\\xb3#\\xb5r\\x9c' bytearray(b'{\"topic\": \"/battery\", \"value\": 41.0}') {b'd\\xe83\\x86\\x8e\\xc8': [-25, 9762263], b'\\xe4\\xb3#\\xb5r\\x9c': [-47, 9762297]}\nb'\\xe4\\xb3#\\xb5r\\x9c' bytearray(b'{\"topic\": \"/battery\", \"value\": 40.4}') {b'd\\xe83\\x86\\x8e\\xc8': [-26, 9828353], b'\\xe4\\xb3#\\xb5r\\x9c': [-49, 9828409]}\nb'\\xe4\\xb3#\\xb5r\\x9c' bytearray(b'{\"topic\": \"/battery\", \"value\": 39.8}') {b'd\\xe83\\x86\\x8e\\xc8': [-25, 9894441], b'\\xe4\\xb3#\\xb5r\\x9c': [-46, 9894521]}\nb'd\\xe83\\x86\\x8e\\xc8' bytearray(b'{\"topic\": \"/battery\", \"value\": 37.8}') {b'd\\xe83\\x86\\x8e\\xc8': [-25, 10092852], b'\\xe4\\xb3#\\xb5r\\x9c': [-45, 10092857]}\nb'\\xe4\\xb3#\\xb5r\\x9c' bytearray(b'{\"topic\": \"/battery\", \"value\": 37.8}') {b'd\\xe83\\x86\\x8e\\xc8': [-25, 10092852], b'\\xe4\\xb3#\\xb5r\\x9c': [-45, 10092857]}\nb'd\\xe83\\x86\\x8e\\xc8' bytearray(b'{\"topic\": \"/battery\", \"value\": 37.2}') {b'd\\xe83\\x86\\x8e\\xc8': [-25, 10158909], b'\\xe4\\xb3#\\xb5r\\x9c': [-46, 10158975]}\nb'\\xe4\\xb3#\\xb5r\\x9c' bytearray(b'{\"topic\": \"/battery\", \"value\": 37.2}') {b'd\\xe83\\x86\\x8e\\xc8': [-25, 10158909], b'\\xe4\\xb3#\\xb5r\\x9c': [-46, 10158975]}\nb'\\xe4\\xb3#\\xb5r\\x9c' bytearray(b'{\"topic\": \"/battery\", \"value\": 36.5}') {b'd\\xe83\\x86\\x8e\\xc8': [-26, 10224953], b'\\xe4\\xb3#\\xb5r\\x9c': [-46, 10225086]}\nb'\\xe4\\xb3#\\xb5r\\x9c' bytearray(b'{\"topic\": \"/battery\", \"value\": 35.9}') {b'd\\xe83\\x86\\x8e\\xc8': [-25, 10291171], b'\\xe4\\xb3#\\xb5r\\x9c': [-44, 10291198]}\nb'\\xe4\\xb3#\\xb5r\\x9c' bytearray(b'{\"topic\": \"/battery\", \"value\": 35.2}') {b'd\\xe83\\x86\\x8e\\xc8': [-26, 10357238], b'\\xe4\\xb3#\\xb5r\\x9c': [-47, 10357309]}\nb'd\\xe83\\x86\\x8e\\xc8' bytearray(b'{\"topic\": \"/battery\", \"value\": 34.5}') {b'd\\xe83\\x86\\x8e\\xc8': [-26, 10423383], b'\\xe4\\xb3#\\xb5r\\x9c': [-46, 10423420]}\nb'\\xe4\\xb3#\\xb5r\\x9c' bytearray(b'{\"topic\": \"/battery\", \"value\": 34.5}') {b'd\\xe83\\x86\\x8e\\xc8': [-26, 10423383], b'\\xe4\\xb3#\\xb5r\\x9c': [-46, 10423420]}\nb'd\\xe83\\x86\\x8e\\xc8' bytearray(b'{\"topic\": \"/battery\", \"value\": 33.8}') {b'd\\xe83\\x86\\x8e\\xc8': [-26, 10489472], b'\\xe4\\xb3#\\xb5r\\x9c': [-48, 10489532]}\nb'\\xe4\\xb3#\\xb5r\\x9c' bytearray(b'{\"topic\": \"/battery\", \"value\": 33.8}') {b'd\\xe83\\x86\\x8e\\xc8': [-26, 10489472], b'\\xe4\\xb3#\\xb5r\\x9c': [-48, 10489532]}\nb'\\xe4\\xb3#\\xb5r\\x9c' bytearray(b'{\"topic\": \"/battery\", \"value\": 33.1}') {b'd\\xe83\\x86\\x8e\\xc8': [-26, 10555527], b'\\xe4\\xb3#\\xb5r\\x9c': [-47, 10555644]}\nb'\\xe4\\xb3#\\xb5r\\x9c' bytearray(b'{\"topic\": \"/battery\", \"value\": 32.4}') {b'd\\xe83\\x86\\x8e\\xc8': [-25, 10621701], b'\\xe4\\xb3#\\xb5r\\x9c': [-47, 10621755]}\nb'\\xe4\\xb3#\\xb5r\\x9c' bytearray(b'{\"topic\": \"/battery\", \"value\": 31.8}') {b'd\\xe83\\x86\\x8e\\xc8': [-27, 10687796], b'\\xe4\\xb3#\\xb5r\\x9c': [-46, 10687866]}\nb'\\xe4\\xb3#\\xb5r\\x9c' bytearray(b'{\"topic\": \"/battery\", \"value\": 31.1}') {b'd\\xe83\\x86\\x8e\\xc8': [-26, 10753853], b'\\xe4\\xb3#\\xb5r\\x9c': [-50, 10753977]}\nb'd\\xe83\\x86\\x8e\\xc8' bytearray(b'{\"topic\": \"/battery\", \"value\": 28.4}') {b'd\\xe83\\x86\\x8e\\xc8': [-25, 11018390], b'\\xe4\\xb3#\\xb5r\\x9c': [-46, 11018423]}\nb'\\xe4\\xb3#\\xb5r\\x9c' bytearray(b'{\"topic\": \"/battery\", \"value\": 28.4}') {b'd\\xe83\\x86\\x8e\\xc8': [-25, 11018390], b'\\xe4\\xb3#\\xb5r\\x9c': [-46, 11018423]}\nb'd\\xe83\\x86\\x8e\\xc8' bytearray(b'{\"topic\": \"/battery\", \"value\": 27.7}') {b'd\\xe83\\x86\\x8e\\xc8': [-25, 11084447], b'\\xe4\\xb3#\\xb5r\\x9c': [-50, 11084535]}\nb'\\xe4\\xb3#\\xb5r\\x9c' bytearray(b'{\"topic\": \"/battery\", \"value\": 27.7}') {b'd\\xe83\\x86\\x8e\\xc8': [-25, 11084447], b'\\xe4\\xb3#\\xb5r\\x9c': [-50, 11084535]}\nb'\\xe4\\xb3#\\xb5r\\x9c' bytearray(b'{\"topic\": \"/battery\", \"value\": 27.1}') {b'd\\xe83\\x86\\x8e\\xc8': [-25, 11150645], b'\\xe4\\xb3#\\xb5r\\x9c': [-46, 11150645]}\nb'd\\xe83\\x86\\x8e\\xc8' bytearray(b'{\"topic\": \"/battery\", \"value\": 26.4}') {b'd\\xe83\\x86\\x8e\\xc8': [-26, 11216620], b'\\xe4\\xb3#\\xb5r\\x9c': [-50, 11216757]}\nb'\\xe4\\xb3#\\xb5r\\x9c' bytearray(b'{\"topic\": \"/battery\", \"value\": 26.4}') {b'd\\xe83\\x86\\x8e\\xc8': [-26, 11216620], b'\\xe4\\xb3#\\xb5r\\x9c': [-50, 11216757]}\nb'd\\xe83\\x86\\x8e\\xc8' bytearray(b'{\"topic\": \"/battery\", \"value\": 25.7}') {b'd\\xe83\\x86\\x8e\\xc8': [-27, 11282861], b'\\xe4\\xb3#\\xb5r\\x9c': [-49, 11282870]}\nb'\\xe4\\xb3#\\xb5r\\x9c' bytearray(b'{\"topic\": \"/battery\", \"value\": 25.7}') {b'd\\xe83\\x86\\x8e\\xc8': [-27, 11282861], b'\\xe4\\xb3#\\xb5r\\x9c': [-49, 11282870]}\nb'\\xe4\\xb3#\\xb5r\\x9c' bytearray(b'{\"topic\": \"/battery\", \"value\": 25.1}') {b'd\\xe83\\x86\\x8e\\xc8': [-30, 11348896], b'\\xe4\\xb3#\\xb5r\\x9c': [-47, 11348981]}\nb'\\xe4\\xb3#\\xb5r\\x9c' bytearray(b'{\"topic\": \"/battery\", \"value\": 24.5}') {b'd\\xe83\\x86\\x8e\\xc8': [-30, 11414961], b'\\xe4\\xb3#\\xb5r\\x9c': [-45, 11415091]}\nb'\\xe4\\xb3#\\xb5r\\x9c' bytearray(b'{\"topic\": \"/battery\", \"value\": 23.8}') {b'd\\xe83\\x86\\x8e\\xc8': [-31, 11481178], b'\\xe4\\xb3#\\xb5r\\x9c': [-45, 11481203]}\nb'\\xe4\\xb3#\\xb5r\\x9c' bytearray(b'{\"topic\": \"/battery\", \"value\": 23.2}') {b'd\\xe83\\x86\\x8e\\xc8': [-30, 11547254], b'\\xe4\\xb3#\\xb5r\\x9c': [-46, 11547316]}\nb'd\\xe83\\x86\\x8e\\xc8' bytearray(b'{\"topic\": \"/battery\", \"value\": 22.5}') {b'd\\xe83\\x86\\x8e\\xc8': [-31, 11613425], b'\\xe4\\xb3#\\xb5r\\x9c': [-46, 11613427]}\nb'\\xe4\\xb3#\\xb5r\\x9c' bytearray(b'{\"topic\": \"/battery\", \"value\": 22.5}') {b'd\\xe83\\x86\\x8e\\xc8': [-31, 11613425], b'\\xe4\\xb3#\\xb5r\\x9c': [-46, 11613427]}\nb'\\xe4\\xb3#\\xb5r\\x9c' bytearray(b'{\"topic\": \"/battery\", \"value\": 21.9}') {b'd\\xe83\\x86\\x8e\\xc8': [-30, 11679447], b'\\xe4\\xb3#\\xb5r\\x9c': [-47, 11679538]}\nb'\\xe4\\xb3#\\xb5r\\x9c' bytearray(b'{\"topic\": \"/battery\", \"value\": 21.3}') {b'd\\xe83\\x86\\x8e\\xc8': [-30, 11745643], b'\\xe4\\xb3#\\xb5r\\x9c': [-46, 11745648]}\nb'd\\xe83\\x86\\x8e\\xc8' bytearray(b'{\"topic\": \"/battery\", \"value\": 20.7}') {b'd\\xe83\\x86\\x8e\\xc8': [-30, 11811626], b'\\xe4\\xb3#\\xb5r\\x9c': [-47, 11811759]}\nb'\\xe4\\xb3#\\xb5r\\x9c' bytearray(b'{\"topic\": \"/battery\", \"value\": 20.7}') {b'd\\xe83\\x86\\x8e\\xc8': [-30, 11811626], b'\\xe4\\xb3#\\xb5r\\x9c': [-47, 11811759]}\nb'\\xe4\\xb3#\\xb5r\\x9c' bytearray(b'{\"topic\": \"/battery\", \"value\": 20.1}') {b'd\\xe83\\x86\\x8e\\xc8': [-30, 11877785], b'\\xe4\\xb3#\\xb5r\\x9c': [-48, 11877871]}\nb'\\xe4\\xb3#\\xb5r\\x9c' bytearray(b'{\"topic\": \"/battery\", \"value\": 19.5}') {b'd\\xe83\\x86\\x8e\\xc8': [-29, 11943877], b'\\xe4\\xb3#\\xb5r\\x9c': [-44, 11943982]}\nb'\\xe4\\xb3#\\xb5r\\x9c' bytearray(b'{\"topic\": \"/battery\", \"value\": 18.8}') {b'd\\xe83\\x86\\x8e\\xc8': [-30, 12009966], b'\\xe4\\xb3#\\xb5r\\x9c': [-46, 12010094]}\nb'd\\xe83\\x86\\x8e\\xc8' bytearray(b'{\"topic\": \"/battery\", \"value\": 18.3}') {b'd\\xe83\\x86\\x8e\\xc8': [-30, 12076119], b'\\xe4\\xb3#\\xb5r\\x9c': [-46, 12076205]}\nb'\\xe4\\xb3#\\xb5r\\x9c' bytearray(b'{\"topic\": \"/battery\", \"value\": 18.3}') {b'd\\xe83\\x86\\x8e\\xc8': [-30, 12076119], b'\\xe4\\xb3#\\xb5r\\x9c': [-46, 12076205]}\nb'\\xe4\\xb3#\\xb5r\\x9c' bytearray(b'{\"topic\": \"/battery\", \"value\": 17.7}') {b'd\\xe83\\x86\\x8e\\xc8': [-30, 12142242], b'\\xe4\\xb3#\\xb5r\\x9c': [-47, 12142316]}\nb'\\xe4\\xb3#\\xb5r\\x9c' bytearray(b'{\"topic\": \"/battery\", \"value\": 17.1}') {b'd\\xe83\\x86\\x8e\\xc8': [-27, 12208324], b'\\xe4\\xb3#\\xb5r\\x9c': [-44, 12208429]}\nb'd\\xe83\\x86\\x8e\\xc8' bytearray(b'{\"topic\": \"/battery\", \"value\": 16.5}') {b'd\\xe83\\x86\\x8e\\xc8': [-29, 12274521], b'\\xe4\\xb3#\\xb5r\\x9c': [-41, 12274539]}\nb'\\xe4\\xb3#\\xb5r\\x9c' bytearray(b'{\"topic\": \"/battery\", \"value\": 16.5}') {b'd\\xe83\\x86\\x8e\\xc8': [-29, 12274521], b'\\xe4\\xb3#\\xb5r\\x9c': [-41, 12274539]}\nb'd\\xe83\\x86\\x8e\\xc8' bytearray(b'{\"topic\": \"/battery\", \"value\": 15.4}') {b'd\\xe83\\x86\\x8e\\xc8': [-30, 12406637], b'\\xe4\\xb3#\\xb5r\\x9c': [-51, 12406762]}\nb'\\xe4\\xb3#\\xb5r\\x9c' bytearray(b'{\"topic\": \"/battery\", \"value\": 15.4}') {b'd\\xe83\\x86\\x8e\\xc8': [-30, 12406637], b'\\xe4\\xb3#\\xb5r\\x9c': [-51, 12406762]}\nb'\\xe4\\xb3#\\xb5r\\x9c' bytearray(b'{\"topic\": \"/battery\", \"value\": 14.9}') {b'd\\xe83\\x86\\x8e\\xc8': [-31, 12472827], b'\\xe4\\xb3#\\xb5r\\x9c': [-50, 12472873]}\nb'\\xe4\\xb3#\\xb5r\\x9c' bytearray(b'{\"topic\": \"/battery\", \"value\": 14.3}') {b'd\\xe83\\x86\\x8e\\xc8': [-31, 12538906], b'\\xe4\\xb3#\\xb5r\\x9c': [-50, 12538985]}\nb'\\xe4\\xb3#\\xb5r\\x9c' bytearray(b'{\"topic\": \"/battery\", \"value\": 13.8}') {b'd\\xe83\\x86\\x8e\\xc8': [-31, 12604985], b'\\xe4\\xb3#\\xb5r\\x9c': [-50, 12605098]}\nb'\\xe4\\xb3#\\xb5r\\x9c' bytearray(b'{\"topic\": \"/battery\", \"value\": 13.3}') {b'd\\xe83\\x86\\x8e\\xc8': [-26, 12671173], b'\\xe4\\xb3#\\xb5r\\x9c': [-48, 12671209]}\nb'\\xe4\\xb3#\\xb5r\\x9c' bytearray(b'{\"topic\": \"/battery\", \"value\": 12.3}') {b'd\\xe83\\x86\\x8e\\xc8': [-25, 12803395], b'\\xe4\\xb3#\\xb5r\\x9c': [-50, 12803430]}\nb'\\xe4\\xb3#\\xb5r\\x9c' bytearray(b'{\"topic\": \"/battery\", \"value\": 11.3}') {b'd\\xe83\\x86\\x8e\\xc8': [-25, 12935525], b'\\xe4\\xb3#\\xb5r\\x9c': [-48, 12935654]}\nb'\\xe4\\xb3#\\xb5r\\x9c' bytearray(b'{\"topic\": \"/battery\", \"value\": 10.8}') {b'd\\xe83\\x86\\x8e\\xc8': [-26, 13001756], b'\\xe4\\xb3#\\xb5r\\x9c': [-48, 13001764]}\nb'\\xe4\\xb3#\\xb5r\\x9c' bytearray(b'{\"topic\": \"/battery\", \"value\": 10.3}') {b'd\\xe83\\x86\\x8e\\xc8': [-25, 13067853], b'\\xe4\\xb3#\\xb5r\\x9c': [-49, 13067876]}\nb'd\\xe83\\x86\\x8e\\xc8' bytearray(b'{\"topic\": \"/battery\", \"value\": 9.9}') {b'd\\xe83\\x86\\x8e\\xc8': [-25, 13133942], b'\\xe4\\xb3#\\xb5r\\x9c': [-48, 13133997]}\nb'\\xe4\\xb3#\\xb5r\\x9c' bytearray(b'{\"topic\": \"/battery\", \"value\": 9.9}') {b'd\\xe83\\x86\\x8e\\xc8': [-25, 13133942], b'\\xe4\\xb3#\\xb5r\\x9c': [-48, 13133997]}\nb'\\xe4\\xb3#\\xb5r\\x9c' bytearray(b'{\"topic\": \"/battery\", \"value\": 8.9}') {b'd\\xe83\\x86\\x8e\\xc8': [-25, 13266147], b'\\xe4\\xb3#\\xb5r\\x9c': [-49, 13266220]}\nb'\\xe4\\xb3#\\xb5r\\x9c' bytearray(b'{\"topic\": \"/battery\", \"value\": 8.5}') {b'd\\xe83\\x86\\x8e\\xc8': [-26, 13332300], b'\\xe4\\xb3#\\xb5r\\x9c': [-49, 13332331]}\nb'\\xe4\\xb3#\\xb5r\\x9c' bytearray(b'{\"topic\": \"/battery\", \"value\": 8.0}') {b'd\\xe83\\x86\\x8e\\xc8': [-26, 13398423], b'\\xe4\\xb3#\\xb5r\\x9c': [-48, 13398443]}\nb'\\xe4\\xb3#\\xb5r\\x9c' bytearray(b'{\"topic\": \"/battery\", \"value\": 5.9}') {b'd\\xe83\\x86\\x8e\\xc8': [-26, 13728995], b'\\xe4\\xb3#\\xb5r\\x9c': [-49, 13729009]}\nb'\\xe4\\xb3#\\xb5r\\x9c' bytearray(b'{\"topic\": \"/battery\", \"value\": 5.6}') {b'd\\xe83\\x86\\x8e\\xc8': [-26, 13795106], b'\\xe4\\xb3#\\xb5r\\x9c': [-49, 13795121]}\nb'\\xe4\\xb3#\\xb5r\\x9c' bytearray(b'{\"topic\": \"/battery\", \"value\": 5.3}') {b'd\\xe83\\x86\\x8e\\xc8': [-25, 13861154], b'\\xe4\\xb3#\\xb5r\\x9c': [-50, 13861232]}\nb'd\\xe83\\x86\\x8e\\xc8' bytearray(b'{\"topic\": \"/battery\", \"value\": 4.9}') {b'd\\xe83\\x86\\x8e\\xc8': [-25, 13927285], b'\\xe4\\xb3#\\xb5r\\x9c': [-49, 13927344]}\nb'\\xe4\\xb3#\\xb5r\\x9c' bytearray(b'{\"topic\": \"/battery\", \"value\": 4.9}') {b'd\\xe83\\x86\\x8e\\xc8': [-25, 13927285], b'\\xe4\\xb3#\\xb5r\\x9c': [-49, 13927344]}\nb'd\\xe83\\x86\\x8e\\xc8' bytearray(b'{\"topic\": \"/battery\", \"value\": 4.8}') {b'd\\xe83\\x86\\x8e\\xc8': [-26, 13993384], b'\\xe4\\xb3#\\xb5r\\x9c': [-47, 13993455]}\nb'\\xe4\\xb3#\\xb5r\\x9c' bytearray(b'{\"topic\": \"/battery\", \"value\": 4.8}') {b'd\\xe83\\x86\\x8e\\xc8': [-26, 13993384], b'\\xe4\\xb3#\\xb5r\\x9c': [-47, 13993455]}\nb'd\\xe83\\x86\\x8e\\xc8' bytearray(b'{\"topic\": \"/battery\", \"value\": 4.6}') {b'd\\xe83\\x86\\x8e\\xc8': [-25, 14059441], b'\\xe4\\xb3#\\xb5r\\x9c': [-23, 14059566]}\nb'\\xe4\\xb3#\\xb5r\\x9c' bytearray(b'{\"topic\": \"/battery\", \"value\": 4.6}') {b'd\\xe83\\x86\\x8e\\xc8': [-25, 14059441], b'\\xe4\\xb3#\\xb5r\\x9c': [-23, 14059566]}\nb'\\xe4\\xb3#\\xb5r\\x9c' bytearray(b'{\"topic\": \"/battery\", \"value\": 4.4}') {b'd\\xe83\\x86\\x8e\\xc8': [-25, 14125664], b'\\xe4\\xb3#\\xb5r\\x9c': [-22, 14125678]}\nb'\\xe4\\xb3#\\xb5r\\x9c' bytearray(b'{\"topic\": \"/battery\", \"value\": 4.2}') {b'd\\xe83\\x86\\x8e\\xc8': [-29, 14191695], b'\\xe4\\xb3#\\xb5r\\x9c': [-21, 14191789]}\nb'\\xe4\\xb3#\\xb5r\\x9c' bytearray(b'{\"topic\": \"/battery\", \"value\": 4.0}') {b'd\\xe83\\x86\\x8e\\xc8': [-29, 14257793], b'\\xe4\\xb3#\\xb5r\\x9c': [-20, 14257901]}\nb'\\xe4\\xb3#\\xb5r\\x9c' bytearray(b'{\"topic\": \"/battery\", \"value\": 3.9}') {b'd\\xe83\\x86\\x8e\\xc8': [-29, 14456133], b'\\xe4\\xb3#\\xb5r\\x9c': [-20, 14456245]}\nb'd\\xe83\\x86\\x8e\\xc8' bytearray(b'{\"topic\": \"/battery\", \"value\": 3.9}') {b'd\\xe83\\x86\\x8e\\xc8': [-28, 14522258], b'\\xe4\\xb3#\\xb5r\\x9c': [-21, 14522357]}\nb'\\xe4\\xb3#\\xb5r\\x9c' bytearray(b'{\"topic\": \"/battery\", \"value\": 3.9}') {b'd\\xe83\\x86\\x8e\\xc8': [-28, 14522258], b'\\xe4\\xb3#\\xb5r\\x9c': [-21, 14522357]}\nb'd\\xe83\\x86\\x8e\\xc8' bytearray(b'{\"topic\": \"/battery\", \"value\": 3.9}') {b'd\\xe83\\x86\\x8e\\xc8': [-29, 14588351], b'\\xe4\\xb3#\\xb5r\\x9c': [-19, 14588467]}\nb'\\xe4\\xb3#\\xb5r\\x9c' bytearray(b'{\"topic\": \"/battery\", \"value\": 3.9}') {b'd\\xe83\\x86\\x8e\\xc8': [-29, 14588351], b'\\xe4\\xb3#\\xb5r\\x9c': [-19, 14588467]}\nb'\\xe4\\xb3#\\xb5r\\x9c' bytearray(b'{\"topic\": \"/battery\", \"value\": 3.9}') {b'd\\xe83\\x86\\x8e\\xc8': [-27, 14654578], b'\\xe4\\xb3#\\xb5r\\x9c': [-19, 14654583]}\nb'\\xe4\\xb3#\\xb5r\\x9c' bytearray(b'{\"topic\": \"/battery\", \"value\": 3.9}') {b'd\\xe83\\x86\\x8e\\xc8': [-27, 14720565], b'\\xe4\\xb3#\\xb5r\\x9c': [-19, 14720700]}\nb'\\xe4\\xb3#\\xb5r\\x9c' bytearray(b'{\"topic\": \"/battery\", \"value\": 3.9}') {b'd\\xe83\\x86\\x8e\\xc8': [-28, 14786679], b'\\xe4\\xb3#\\xb5r\\x9c': [-19, 14786812]}\nb'\\xe4\\xb3#\\xb5r\\x9c' bytearray(b'{\"topic\": \"/battery\", \"value\": 3.9}') {b'd\\xe83\\x86\\x8e\\xc8': [-28, 14852897], b'\\xe4\\xb3#\\xb5r\\x9c': [-19, 14852926]}\nb'\\xe4\\xb3#\\xb5r\\x9c' bytearray(b'{\"topic\": \"/battery\", \"value\": 3.9}') {b'd\\xe83\\x86\\x8e\\xc8': [-27, 14919030], b'\\xe4\\xb3#\\xb5r\\x9c': [-19, 14919035]}\nb'd\\xe83\\x86\\x8e\\xc8' bytearray(b'{\"topic\": \"/battery\", \"value\": 3.8}') {b'd\\xe83\\x86\\x8e\\xc8': [-27, 14985136], b'\\xe4\\xb3#\\xb5r\\x9c': [-19, 14985146]}\nb'\\xe4\\xb3#\\xb5r\\x9c' bytearray(b'{\"topic\": \"/battery\", \"value\": 3.8}') {b'd\\xe83\\x86\\x8e\\xc8': [-27, 14985136], b'\\xe4\\xb3#\\xb5r\\x9c': [-19, 14985146]}\nb'\\xe4\\xb3#\\xb5r\\x9c' bytearray(b'{\"topic\": \"/battery\", \"value\": 3.7}') {b'd\\xe83\\x86\\x8e\\xc8': [-28, 15117350], b'\\xe4\\xb3#\\xb5r\\x9c': [-20, 15117371]}\nb'\\xe4\\xb3#\\xb5r\\x9c' bytearray(b'{\"topic\": \"/battery\", \"value\": 3.6}') {b'd\\xe83\\x86\\x8e\\xc8': [-27, 15183438], b'\\xe4\\xb3#\\xb5r\\x9c': [-19, 15183480]}\nb'\\xe4\\xb3#\\xb5r\\x9c' bytearray(b'{\"topic\": \"/battery\", \"value\": 3.6}') {b'd\\xe83\\x86\\x8e\\xc8': [-27, 15249494], b'\\xe4\\xb3#\\xb5r\\x9c': [-18, 15249591]}\nb'\\xe4\\xb3#\\xb5r\\x9c' bytearray(b'{\"topic\": \"/battery\", \"value\": 3.5}') {b'd\\xe83\\x86\\x8e\\xc8': [-27, 15315593], b'\\xe4\\xb3#\\xb5r\\x9c': [-17, 15315703]}\nb'd\\xe83\\x86\\x8e\\xc8' bytearray(b'{\"topic\": \"/battery\", \"value\": 3.4}') {b'd\\xe83\\x86\\x8e\\xc8': [-26, 15381731], b'\\xe4\\xb3#\\xb5r\\x9c': [-16, 15381815]}\nb'\\xe4\\xb3#\\xb5r\\x9c' bytearray(b'{\"topic\": \"/battery\", \"value\": 3.4}') {b'd\\xe83\\x86\\x8e\\xc8': [-26, 15381731], b'\\xe4\\xb3#\\xb5r\\x9c': [-16, 15381815]}\nb'\\xe4\\xb3#\\xb5r\\x9c' bytearray(b'{\"topic\": \"/battery\", \"value\": 3.3}') {b'd\\xe83\\x86\\x8e\\xc8': [-33, 15447924], b'\\xe4\\xb3#\\xb5r\\x9c': [-21, 15447926]}\nb'\\xe4\\xb3#\\xb5r\\x9c' bytearray(b'{\"topic\": \"/battery\", \"value\": 3.2}') {b'd\\xe83\\x86\\x8e\\xc8': [-32, 15514020], b'\\xe4\\xb3#\\xb5r\\x9c': [-20, 15514038]}\nb'\\xe4\\xb3#\\xb5r\\x9c' bytearray(b'{\"topic\": \"/battery\", \"value\": 3.1}') {b'd\\xe83\\x86\\x8e\\xc8': [-32, 15580099], b'\\xe4\\xb3#\\xb5r\\x9c': [-20, 15580148]}\nb'd\\xe83\\x86\\x8e\\xc8' bytearray(b'{\"topic\": \"/battery\", \"value\": 2.9}') {b'd\\xe83\\x86\\x8e\\xc8': [-33, 15712256], b'\\xe4\\xb3#\\xb5r\\x9c': [-20, 15712371]}\nb'\\xe4\\xb3#\\xb5r\\x9c' bytearray(b'{\"topic\": \"/battery\", \"value\": 2.9}') {b'd\\xe83\\x86\\x8e\\xc8': [-33, 15712256], b'\\xe4\\xb3#\\xb5r\\x9c': [-20, 15712371]}\nb'\\xe4\\xb3#\\xb5r\\x9c' bytearray(b'{\"topic\": \"/battery\", \"value\": 2.9}') {b'd\\xe83\\x86\\x8e\\xc8': [-33, 15778472], b'\\xe4\\xb3#\\xb5r\\x9c': [-20, 15778485]}\nb'\\xe4\\xb3#\\xb5r\\x9c' bytearray(b'{\"topic\": \"/battery\", \"value\": 2.9}') {b'd\\xe83\\x86\\x8e\\xc8': [-33, 15844526], b'\\xe4\\xb3#\\xb5r\\x9c': [-19, 15844595]}\nb'\\xe4\\xb3#\\xb5r\\x9c' bytearray(b'{\"topic\": \"/battery\", \"value\": 3.0}') {b'd\\xe83\\x86\\x8e\\xc8': [-32, 15910584], b'\\xe4\\xb3#\\xb5r\\x9c': [-20, 15910705]}\nb'\\xe4\\xb3#\\xb5r\\x9c' bytearray(b'{\"topic\": \"/battery\", \"value\": 2.9}') {b'd\\xe83\\x86\\x8e\\xc8': [-32, 15976703], b'\\xe4\\xb3#\\xb5r\\x9c': [-20, 15976816]}\nb'\\xe4\\xb3#\\xb5r\\x9c' bytearray(b'{\"topic\": \"/battery\", \"value\": 2.9}') {b'd\\xe83\\x86\\x8e\\xc8': [-30, 16108948], b'\\xe4\\xb3#\\xb5r\\x9c': [-20, 16109040]}\nb'\\xe4\\xb3#\\xb5r\\x9c' bytearray(b'{\"topic\": \"/battery\", \"value\": 2.9}') {b'd\\xe83\\x86\\x8e\\xc8': [-31, 16175039], b'\\xe4\\xb3#\\xb5r\\x9c': [-21, 16175161]}\nb'\\xe4\\xb3#\\xb5r\\x9c' bytearray(b'{\"topic\": \"/battery\", \"value\": 2.9}') {b'd\\xe83\\x86\\x8e\\xc8': [-32, 16241146], b'\\xe4\\xb3#\\xb5r\\x9c': [-21, 16241273]}\nb'\\xe4\\xb3#\\xb5r\\x9c' bytearray(b'{\"topic\": \"/battery\", \"value\": 3.0}') {b'd\\xe83\\x86\\x8e\\xc8': [-31, 16307347], b'\\xe4\\xb3#\\xb5r\\x9c': [-21, 16307384]}\nb'\\xe4\\xb3#\\xb5r\\x9c' bytearray(b'{\"topic\": \"/battery\", \"value\": 2.9}') {b'd\\xe83\\x86\\x8e\\xc8': [-33, 16373412], b'\\xe4\\xb3#\\xb5r\\x9c': [-20, 16373495]}\nb'\\xe4\\xb3#\\xb5r\\x9c' bytearray(b'{\"topic\": \"/battery\", \"value\": 3.0}') {b'd\\xe83\\x86\\x8e\\xc8': [-31, 16439480], b'\\xe4\\xb3#\\xb5r\\x9c': [-21, 16439606]}\nb'\\xe4\\xb3#\\xb5r\\x9c' bytearray(b'{\"topic\": \"/battery\", \"value\": 2.9}') {b'd\\xe83\\x86\\x8e\\xc8': [-32, 16571786], b'\\xe4\\xb3#\\xb5r\\x9c': [-21, 16571839]}\nb'\\xe4\\xb3#\\xb5r\\x9c' bytearray(b'{\"topic\": \"/battery\", \"value\": 3.0}') {b'd\\xe83\\x86\\x8e\\xc8': [-34, 16637857], b'\\xe4\\xb3#\\xb5r\\x9c': [-21, 16637951]}\nb'\\xe4\\xb3#\\xb5r\\x9c' bytearray(b'{\"topic\": \"/battery\", \"value\": 2.9}') {b'd\\xe83\\x86\\x8e\\xc8': [-32, 16836255], b'\\xe4\\xb3#\\xb5r\\x9c': [-15, 16836286]}\nb'd\\xe83\\x86\\x8e\\xc8' bytearray(b'{\"topic\": \"/battery\", \"value\": 2.9}') {b'd\\xe83\\x86\\x8e\\xc8': [-31, 16902346], b'\\xe4\\xb3#\\xb5r\\x9c': [-16, 16902396]}\nb'\\xe4\\xb3#\\xb5r\\x9c' bytearray(b'{\"topic\": \"/battery\", \"value\": 2.9}') {b'd\\xe83\\x86\\x8e\\xc8': [-31, 16902346], b'\\xe4\\xb3#\\xb5r\\x9c': [-16, 16902396]}\nb'd\\xe83\\x86\\x8e\\xc8' bytearray(b'{\"topic\": \"/battery\", \"value\": 2.9}') {b'd\\xe83\\x86\\x8e\\xc8': [-31, 16968437], b'\\xe4\\xb3#\\xb5r\\x9c': [-16, 16968508]}\nb'\\xe4\\xb3#\\xb5r\\x9c' bytearray(b'{\"topic\": \"/battery\", \"value\": 2.9}') {b'd\\xe83\\x86\\x8e\\xc8': [-31, 16968437], b'\\xe4\\xb3#\\xb5r\\x9c': [-16, 16968508]}\nb'd\\xe83\\x86\\x8e\\xc8' bytearray(b'{\"topic\": \"/battery\", \"value\": 2.9}') {b'd\\xe83\\x86\\x8e\\xc8': [-31, 17034544], b'\\xe4\\xb3#\\xb5r\\x9c': [-15, 17034620]}\nb'\\xe4\\xb3#\\xb5r\\x9c' bytearray(b'{\"topic\": \"/battery\", \"value\": 2.9}') {b'd\\xe83\\x86\\x8e\\xc8': [-31, 17034544], b'\\xe4\\xb3#\\xb5r\\x9c': [-15, 17034620]}\nb'\\xe4\\xb3#\\xb5r\\x9c' bytearray(b'{\"topic\": \"/battery\", \"value\": 2.8}') {b'd\\xe83\\x86\\x8e\\xc8': [-25, 17166731], b'\\xe4\\xb3#\\xb5r\\x9c': [-15, 17166852]}\nb'd\\xe83\\x86\\x8e\\xc8' bytearray(b'{\"topic\": \"/battery\", \"value\": 2.7}') {b'd\\xe83\\x86\\x8e\\xc8': [-29, 17232925], b'\\xe4\\xb3#\\xb5r\\x9c': [-20, 17232973]}\nb'\\xe4\\xb3#\\xb5r\\x9c' bytearray(b'{\"topic\": \"/battery\", \"value\": 2.7}') {b'd\\xe83\\x86\\x8e\\xc8': [-29, 17232925], b'\\xe4\\xb3#\\xb5r\\x9c': [-20, 17232973]}\nb'd\\xe83\\x86\\x8e\\xc8' bytearray(b'{\"topic\": \"/battery\", \"value\": 2.7}') {b'd\\xe83\\x86\\x8e\\xc8': [-29, 17299001], b'\\xe4\\xb3#\\xb5r\\x9c': [-20, 17299087]}\nb'\\xe4\\xb3#\\xb5r\\x9c' bytearray(b'{\"topic\": \"/battery\", \"value\": 2.7}') {b'd\\xe83\\x86\\x8e\\xc8': [-29, 17299001], b'\\xe4\\xb3#\\xb5r\\x9c': [-20, 17299087]}\nb'd\\xe83\\x86\\x8e\\xc8' bytearray(b'{\"topic\": \"/battery\", \"value\": 2.6}') {b'd\\xe83\\x86\\x8e\\xc8': [-29, 17365064], b'\\xe4\\xb3#\\xb5r\\x9c': [-20, 17365196]}\nb'\\xe4\\xb3#\\xb5r\\x9c' bytearray(b'{\"topic\": \"/battery\", \"value\": 2.6}') {b'd\\xe83\\x86\\x8e\\xc8': [-29, b'\\xe4\\xb3#\\xb5r\\x9c' bytearray(b'{\"topic\": \"/battery\", \"value\": 2.0}') {b'd\\xe83\\x86\\x8e\\xc8': [-29, 18026243], b'\\xe4\\xb3#\\xb5r\\x9c': [-20, 18026310]}\nb'\\xe4\\xb3#\\xb5r\\x9c' bytearray(b'{\"topic\": \"/battery\", \"value\": 1.9}') {b'd\\xe83\\x86\\x8e\\xc8': [-29, 18092339], b'\\xe4\\xb3#\\xb5r\\x9c': [-20, 18092424]}\nb'\\xe4\\xb3#\\xb5r\\x9c' bytearray(b'{\"topic\": \"/battery\", \"value\": 1.9}') {b'd\\xe83\\x86\\x8e\\xc8': [-29, b'\\xe4\\xb3#\\xb5r\\x9c' bytearray(b'{\"topic\": \"/battery\", \"value\": 1.9}') {b'd\\xe83\\x86\\x8e\\xc8': [-29, 18819613], b'\\xe4\\xb3#\\xb5r\\x9c': [-20, 18819647]}\nb'\\xe4\\xb3#\\xb5r\\x9c' bytearray(b'{\"topic\": \"/battery\", \"value\": 1.9}') {b'd\\xe83\\x86\\x8e\\xc8': [-29, 18885729], b'\\xe4\\xb3#\\xb5r\\x9c': [-20, 18885758]}\nb'\\xe4\\xb3#\\xb5r\\x9c' bytearray(b'{\"topic\": \"/battery\", \"value\": 1.9}') {b'd\\xe83\\x86\\x8e\\xc8': [-29, 18951805], b'\\xe4\\xb3#\\xb5r\\x9c': [-20, 18951869]}\nb'd\\xe83\\x86\\x8e\\xc8' bytearray(b'{\"topic\": \"/battery\", \"value\": 1.9}') {b'd\\xe83\\x86\\x8e\\xc8': [-29, 19017892], b'\\xe4\\xb3#\\xb5r\\x9c': [-20, 19017981]}\nb'\\xe4\\xb3#\\xb5r\\x9c' bytearray(b'{\"topic\": \"/battery\", \"value\": 1.9}') {b'd\\xe83\\x86\\x8e\\xc8': [-29, 19017892], b'\\xe4\\xb3#\\xb5r\\x9c': [-20, 19017981]}\nb'\\xe4\\xb3#\\xb5r\\x9c' bytearray(b'{\"topic\": \"/battery\", \"value\": 1.9}') {b'd\\xe83\\x86\\x8e\\xc8': [-29, 19084070], b'\\xe4\\xb3#\\xb5r\\x9c': [-20, 19084092]}\nb'\\xe4\\xb3#\\xb5r\\x9c' bytearray(b'{\"topic\": \"/battery\", \"value\": 1.9}') {b'd\\xe83\\x86\\x8e\\xc8': [-29, 19150122], b'\\xe4\\xb3#\\xb5r\\x9c': [-20, 19150203]}\nb'\\xe4\\xb3#\\xb5r\\x9c' bytearray(b'{\"topic\": \"/battery\", \"value\": 1.9}') {b'd\\xe83\\x86\\x8e\\xc8': [-29, 19216204], b'\\xe4\\xb3#\\xb5r\\x9c': [-20, 19216315]}\nb'\\xe4\\xb3#\\xb5r\\x9c' bytearray(b'{\"topic\": \"/battery\", \"value\": 1.1}') {b'd\\xe83\\x86\\x8e\\xc8': [-29, 19480632], b'\\xe4\\xb3#\\xb5r\\x9c': [-20, 19480760]}\nb'd\\xe83\\x86\\x8e\\xc8' bytearray(b'{\"topic\": \"/battery\", \"value\": 0.9}') {b'd\\xe83\\x86\\x8e\\xc8': [-29, 19612863], b'\\xe4\\xb3#\\xb5r\\x9c': [-20, 19612983]}\nb'\\xe4\\xb3#\\xb5r\\x9c' bytearray(b'{\"topic\": \"/battery\", \"value\": 0.9}') {b'd\\xe83\\x86\\x8e\\xc8': [-29, 19612863], b'\\xe4\\xb3#\\xb5r\\x9c': [-20, 19612983]}\nb'\\xe4\\xb3#\\xb5r\\x9c' bytearray(b'{\"topic\": \"/battery\", \"value\": 0.8}') {b'd\\xe83\\x86\\x8e\\xc8': [-29, 19679096], b'\\xe4\\xb3#\\xb5r\\x9c': [-20, 19679096]}\nb'\\xe4\\xb3#\\xb5r\\x9c' bytearray(b'{\"topic\": \"/battery\", \"value\": 0.6}') {b'd\\xe83\\x86\\x8e\\xc8': [-29, 19745152], b'\\xe4\\xb3#\\xb5r\\x9c': [-20, 19745208]}\nb'\\xe4\\xb3#\\xb5r\\x9c' bytearray(b'{\"topic\": \"/battery\", \"value\": 0.1}') {b'd\\xe83\\x86\\x8e\\xc8': [-29, 19811206], b'\\xe4\\xb3#\\xb5r\\x9c': [-20, 19811317]}\nb'\\xe4\\xb3#\\xb5r\\x9c' bytearray(b'{\"topic\": \"/battery\", \"value\": 0.0}') {b'd\\xe83\\x86\\x8e\\xc8': [-29, 19943457], b'\\xe4\\xb3#\\xb5r\\x9c': [-20, 19943540]}\n"
  out "XY Graph":cluster{"X":dbl, "Y":dbl}[](graph)=[{"X"=0.018364722222222223, "Y"=0.2}, {"X"=0.036728611111111115, "Y"=0.2}, {"X"=0.055092777777777775, "Y"=0.7}, {"X"=0.0734575, "Y"=1.0}, {"X"=0.09182166666666666, "Y"=1.1}, {"X"=0.11018583333333333, "Y"=1.2}, {"X"=0.12855111111111112, "Y"=1.4}, {"X"=0.14691444444444446, "Y"=1.7}, {"X"=0.16527916666666667, "Y"=2.0}, {"X"=0.18364277777777777, "Y"=2.0}, {"X"=0.20200777777777776, "Y"=2.0}, {"X"=0.22037138888888888, "Y"=2.0}, {"X"=0.23873555555555553, "Y"=2.0}, {"X"=0.2571, "Y"=2.1}, {"X"=0.2754641666666667, "Y"=2.1}, {"X"=0.2938288888888889, "Y"=2.2}, {"X"=0.3305572222222223, "Y"=2.3}, {"X"=0.3489213888888889, "Y"=2.4}, {"X"=0.4223783333333333, "Y"=2.8}, {"X"=0.4407433333333333, "Y"=2.8}, {"X"=0.4591088888888889, "Y"=2.9}, {"X"=0.47747472222222226, "Y"=2.9}, {"X"=0.4958383333333333, "Y"=2.9}, {"X"=0.5142025, "Y"=3.0}, {"X"=0.6060244444444444, "Y"=3.0}, {"X"=0.6243880555555557, "Y"=2.9}, {"X"=0.6427525000000001, "Y"=3.0}, {"X"=0.6611172222222221, "Y"=3.0}, {"X"=0.6794811111111111, "Y"=3.0}, {"X"=0.6978452777777778, "Y"=3.0}, {"X"=0.7162094444444445, "Y"=3.0}, {"X"=0.7345738888888889, "Y"=3.0}, {"X"=0.7529380555555556, "Y"=3.0}, {"X"=0.7713024999999999, "Y"=3.0}, {"X"=0.7896666666666667, "Y"=3.0}, {"X"=0.808031111111111, "Y"=3.0}, {"X"=0.8263952777777778, "Y"=3.0}, {"X"=0.8447600000000001, "Y"=3.1}, {"X"=0.8631238888888889, "Y"=3.1}, {"X"=0.8814886111111111, "Y"=3.2}, {"X"=0.8998524999999999, "Y"=3.3}, {"X"=0.9182166666666666, "Y"=3.5}, {"X"=0.936581388888889, "Y"=3.6}, {"X"=0.9549452777777777, "Y"=3.7}, {"X"=0.97331, "Y"=3.9}, {"X"=0.9916738888888889, "Y"=4.0}, {"X"=1.0100380555555557, "Y"=4.0}, {"X"=1.0284022222222222, "Y"=4.0}, {"X"=1.0467666666666668, "Y"=4.0}, {"X"=1.0651311111111113, "Y"=4.0}, {"X"=1.083496111111111, "Y"=4.0}, {"X"=1.1018597222222224, "Y"=4.0}, {"X"=1.120223611111111, "Y"=4.0}, {"X"=1.1385880555555556, "Y"=4.0}, {"X"=1.1569525, "Y"=4.0}, {"X"=1.175316388888889, "Y"=4.0}, {"X"=1.1936808333333333, "Y"=4.0}, {"X"=1.212045, "Y"=4.0}, {"X"=1.2304099999999998, "Y"=4.0}, {"X"=1.2487738888888888, "Y"=4.0}, {"X"=1.2855022222222223, "Y"=4.2}, {"X"=1.3038663888888888, "Y"=4.3}, {"X"=1.3222308333333332, "Y"=4.4}, {"X"=1.3956880555555555, "Y"=4.8}, {"X"=1.414052222222222, "Y"=4.9}, {"X"=1.4324172222222225, "Y"=5.0}, {"X"=1.4507808333333332, "Y"=5.0}, {"X"=1.4691455555555557, "Y"=5.0}, {"X"=1.4875091666666667, "Y"=5.0}, {"X"=1.505873611111111, "Y"=5.0}, {"X"=1.5242377777777778, "Y"=5.0}, {"X"=1.5426024999999999, "Y"=5.0}, {"X"=1.560966388888889, "Y"=5.0}, {"X"=1.5793308333333334, "Y"=5.0}, {"X"=1.597695, "Y"=5.0}, {"X"=1.6160591666666666, "Y"=5.0}, {"X"=1.6344238888888891, "Y"=5.0}, {"X"=1.6527883333333333, "Y"=5.0}, {"X"=1.6711552777777776, "Y"=5.0}, {"X"=1.6895222222222221, "Y"=5.0}, {"X"=1.7078872222222223, "Y"=5.0}, {"X"=1.7262516666666667, "Y"=5.0}, {"X"=1.7446147222222224, "Y"=5.0}, {"X"=1.7629788888888889, "Y"=5.0}, {"X"=1.7813433333333333, "Y"=5.0}, {"X"=1.7997075, "Y"=5.0}, {"X"=1.8180719444444444, "Y"=5.0}, {"X"=1.8364361111111112, "Y"=5.0}, {"X"=1.8548002777777777, "Y"=5.1}, {"X"=1.873165, "Y"=5.2}, {"X"=1.8915288888888888, "Y"=5.2}, {"X"=1.9098933333333332, "Y"=5.3}, {"X"=1.9282575, "Y"=5.4}, {"X"=1.9466216666666665, "Y"=5.5}, {"X"=1.964986388888889, "Y"=5.6}, {"X"=1.9833502777777776, "Y"=5.8}, {"X"=2.001714444444444, "Y"=5.9}, {"X"=2.0200788888888885, "Y"=6.0}, {"X"=2.038443333333333, "Y"=6.0}, {"X"=2.0568074999999997, "Y"=6.0}, {"X"=2.0751719444444445, "Y"=6.1}, {"X"=2.093536388888889, "Y"=6.2}, {"X"=2.1119002777777776, "Y"=6.3}, {"X"=2.1302644444444443, "Y"=6.4}, {"X"=2.1486288888888887, "Y"=6.5}, {"X"=2.166993888888889, "Y"=6.6}, {"X"=2.185357222222222, "Y"=6.7}, {"X"=2.2037216666666666, "Y"=6.9}, {"X"=2.2220858333333333, "Y"=7.0}, {"X"=2.2404505555555554, "Y"=7.2}, {"X"=2.2588155555555556, "Y"=7.3}, {"X"=2.277178611111111, "Y"=7.4}, {"X"=2.2955430555555556, "Y"=7.6}, {"X"=2.3139072222222223, "Y"=7.8}, {"X"=2.3322716666666663, "Y"=8.0}, {"X"=2.3506361111111116, "Y"=8.2}, {"X"=2.3689999999999998, "Y"=8.4}, {"X"=2.3873644444444446, "Y"=8.6}, {"X"=2.405728611111111, "Y"=8.9}, {"X"=2.4240930555555553, "Y"=9.1}, {"X"=2.442457222222222, "Y"=9.3}, {"X"=2.460821666666667, "Y"=9.6}, {"X"=2.479185833333333, "Y"=9.8}, {"X"=2.49755, "Y"=10.1}, {"X"=2.515914444444444, "Y"=10.4}, {"X"=2.534278888888889, "Y"=10.7}, {"X"=2.5526433333333336, "Y"=11.0}, {"X"=2.6628294444444447, "Y"=13.0}, {"X"=2.681193888888889, "Y"=13.4}, {"X"=2.699557222222223, "Y"=13.7}, {"X"=2.7179213888888887, "Y"=14.1}, {"X"=2.7362855555555554, "Y"=14.5}, {"X"=2.773014166666667, "Y"=15.3}, {"X"=2.7913802777777774, "Y"=15.7}, {"X"=2.8097455555555557, "Y"=16.1}, {"X"=2.828109722222222, "Y"=16.5}, {"X"=2.846474444444445, "Y"=17.0}, {"X"=2.864838333333333, "Y"=17.4}, {"X"=2.883202777777778, "Y"=17.8}, {"X"=2.9015669444444443, "Y"=18.3}, {"X"=2.919931111111111, "Y"=18.7}, {"X"=2.9382958333333336, "Y"=19.2}, {"X"=2.956660277777778, "Y"=19.6}, {"X"=2.9750241666666666, "Y"=20.1}, {"X"=2.9933883333333338, "Y"=20.6}, {"X"=3.0117524999999996, "Y"=21.0}, {"X"=3.0301169444444445, "Y"=21.5}, {"X"=3.0484816666666665, "Y"=22.0}, {"X"=3.0668455555555556, "Y"=22.5}, {"X"=3.0852097222222223, "Y"=23.0}, {"X"=3.1035741666666667, "Y"=23.5}, {"X"=3.121938333333333, "Y"=24.1}, {"X"=3.140302777777778, "Y"=24.6}, {"X"=3.158666944444444, "Y"=25.2}, {"X"=3.177031388888889, "Y"=25.7}, {"X"=3.1953955555555558, "Y"=26.3}, {"X"=3.213759722222222, "Y"=26.8}, {"X"=3.232123888888889, "Y"=27.4}, {"X"=3.2504899999999997, "Y"=28.0}, {"X"=3.268855555555555, "Y"=28.6}, {"X"=3.2872194444444447, "Y"=29.2}, {"X"=3.305583888888889, "Y"=29.8}, {"X"=3.3239480555555554, "Y"=30.4}, {"X"=3.3423125000000002, "Y"=31.0}, {"X"=3.3606780555555558, "Y"=31.7}, {"X"=3.3790408333333337, "Y"=32.3}, {"X"=3.397405555555556, "Y"=33.0}, {"X"=3.4157697222222225, "Y"=33.6}, {"X"=3.4341341666666665, "Y"=34.3}, {"X"=3.4524983333333332, "Y"=35.0}, {"X"=3.4708630555555553, "Y"=35.6}, {"X"=3.4892280555555555, "Y"=36.3}, {"X"=3.507592777777778, "Y"=37.0}, {"X"=3.5259577777777777, "Y"=37.7}, {"X"=3.5443225, "Y"=38.4}, {"X"=3.5626863888888893, "Y"=39.1}, {"X"=3.5810508333333333, "Y"=39.8}, {"X"=3.599415, "Y"=40.5}, {"X"=3.6177791666666663, "Y"=41.3}, {"X"=3.636143611111111, "Y"=42.0}, {"X"=3.654507777777778, "Y"=42.7}, {"X"=3.6728722222222223, "Y"=43.4}, {"X"=3.6912363888888886, "Y"=44.2}, {"X"=3.709601111111111, "Y"=44.9}, {"X"=3.727965, "Y"=45.6}, {"X"=3.746329166666667, "Y"=46.3}, {"X"=3.7646936111111113, "Y"=47.0}, {"X"=3.7830577777777776, "Y"=47.7}, {"X"=3.8014222222222225, "Y"=48.5}, {"X"=3.8197863888888888, "Y"=49.2}, {"X"=3.838150555555556, "Y"=49.9}, {"X"=3.856515, "Y"=50.6}, {"X"=3.8748794444444448, "Y"=51.3}, {"X"=3.893243611111111, "Y"=52.0}, {"X"=3.911607777777778, "Y"=52.7}, {"X"=3.9299719444444445, "Y"=53.4}, {"X"=3.948336388888889, "Y"=54.1}, {"X"=3.9667005555555552, "Y"=54.8}, {"X"=3.9850661111111108, "Y"=55.5}, {"X"=4.003429166666667, "Y"=56.2}, {"X"=4.021793333333333, "Y"=56.9}, {"X"=4.040157777777777, "Y"=57.6}, {"X"=4.0585225000000005, "Y"=58.3}, {"X"=4.076886944444444, "Y"=59.0}, {"X"=4.095250555555555, "Y"=59.6}, {"X"=4.113614999999999, "Y"=60.3}, {"X"=4.1319791666666665, "Y"=61.0}, {"X"=4.1503436111111105, "Y"=61.7}, {"X"=4.168707777777778, "Y"=62.4}, {"X"=4.187071944444445, "Y"=63.1}, {"X"=4.2054366666666665, "Y"=63.8}, {"X"=4.223800555555555, "Y"=64.5}, {"X"=4.242164722222222, "Y"=65.2}, {"X"=4.260528888888889, "Y"=65.9}, {"X"=4.2788933333333325, "Y"=66.5}, {"X"=4.29725861111111, "Y"=67.2}, {"X"=4.315622222222222, "Y"=67.9}, {"X"=4.333986111111112, "Y"=68.6}, {"X"=4.352350555555556, "Y"=69.3}, {"X"=4.370715000000001, "Y"=70.0}, {"X"=4.389080000000001, "Y"=70.7}, {"X"=4.407443611111111, "Y"=71.4}, {"X"=4.4258075, "Y"=72.0}, {"X"=4.444171944444445, "Y"=72.7}, {"X"=4.462536111111111, "Y"=73.3}, {"X"=4.480900555555555, "Y"=74.0}, {"X"=4.499265555555556, "Y"=74.6}, {"X"=4.517628888888889, "Y"=75.2}, {"X"=4.664543055555556, "Y"=79.9}, {"X"=4.6829075, "Y"=80.4}, {"X"=4.701271944444445, "Y"=81.0}, {"X"=4.738000277777777, "Y"=82.1}, {"X"=4.756365000000001, "Y"=82.6}, {"X"=4.774728888888889, "Y"=83.1}, {"X"=4.7930930555555555, "Y"=83.7}, {"X"=4.8114575, "Y"=84.2}, {"X"=4.829822222222222, "Y"=84.7}, {"X"=4.848185833333334, "Y"=85.2}, {"X"=4.866550277777777, "Y"=85.8}, {"X"=4.884914444444444, "Y"=86.3}, {"X"=4.90327861111111, "Y"=86.8}, {"X"=4.921643333333334, "Y"=87.3}, {"X"=4.940007222222222, "Y"=87.9}, {"X"=4.958371666666666, "Y"=88.4}, {"X"=4.976735833333334, "Y"=88.9}, {"X"=4.9951, "Y"=89.5}, {"X"=5.013464444444446, "Y"=90.0}, {"X"=5.031828611111111, "Y"=90.5}, {"X"=5.050193055555555, "Y"=91.0}, {"X"=5.068557222222222, "Y"=91.4}, {"X"=5.0869213888888885, "Y"=91.9}, {"X"=5.105286944444444, "Y"=92.3}, {"X"=5.12365, "Y"=92.8}, {"X"=5.142014444444444, "Y"=93.2}, {"X"=5.160378611111112, "Y"=93.5}, {"X"=5.178742777777777, "Y"=93.9}, {"X"=5.197107222222223, "Y"=94.3}, {"X"=5.215471388888889, "Y"=94.6}, {"X"=5.233836388888889, "Y"=94.9}, {"X"=5.252199999999999, "Y"=95.3}, {"X"=5.270564166666666, "Y"=95.6}, {"X"=5.288928611111111, "Y"=95.9}, {"X"=5.307292777777778, "Y"=96.1}, {"X"=5.325656944444445, "Y"=96.3}, {"X"=5.344021388888889, "Y"=96.5}, {"X"=5.362385555555556, "Y"=96.7}, {"X"=5.380750000000001, "Y"=96.9}, {"X"=5.399114166666667, "Y"=97.0}, {"X"=5.41747861111111, "Y"=97.1}, {"X"=5.435842777777777, "Y"=97.3}, {"X"=5.4542075, "Y"=97.4}, {"X"=5.472571388888889, "Y"=97.5}, {"X"=5.490935555555555, "Y"=97.6}, {"X"=5.509299722222222, "Y"=97.7}, {"X"=5.527664166666667, "Y"=97.8}, {"X"=5.546028333333334, "Y"=98.0}, {"X"=5.564392499999999, "Y"=98.0}, {"X"=5.582757222222223, "Y"=98.0}, {"X"=5.601121111111111, "Y"=98.0}, {"X"=5.619485555555556, "Y"=98.0}, {"X"=5.637849722222222, "Y"=98.0}, {"X"=5.6562141666666665, "Y"=98.0}, {"X"=5.674578333333333, "Y"=98.0}, {"X"=5.692943611111111, "Y"=98.0}, {"X"=5.7113075, "Y"=98.0}, {"X"=5.729671111111111, "Y"=98.0}, {"X"=5.7480352777777775, "Y"=98.0}, {"X"=5.766400277777778, "Y"=98.0}, {"X"=5.7847638888888895, "Y"=98.0}, {"X"=5.803128055555556, "Y"=98.0}, {"X"=5.821492500000001, "Y"=98.0}, {"X"=5.839856944444445, "Y"=98.0}, {"X"=5.858221666666667, "Y"=98.0}, {"X"=5.876585277777777, "Y"=98.0}, {"X"=5.894949444444444, "Y"=98.0}, {"X"=5.913313888888889, "Y"=98.0}, {"X"=5.9316780555555555, "Y"=98.0}]
  out "battery":dbl[](graph)=[0.2, 0.2, 0.7, 1.0, 1.1, 1.2, 1.4, 1.7, 2.0, 2.0, 2.0, 2.0, 2.0, 2.1, 2.1, 2.2, 2.3, 2.4, 2.8, 2.8, 2.9, 2.9, 2.9, 3.0, 3.0, 2.9, 3.0, 3.0, 3.0, 3.0, 3.0, 3.0, 3.0, 3.0, 3.0, 3.0, 3.0, 3.1, 3.1, 3.2, 3.3, 3.5, 3.6, 3.7, 3.9, 4.0, 4.0, 4.0, 4.0, 4.0, 4.0, 4.0, 4.0, 4.0, 4.0, 4.0, 4.0, 4.0, 4.0, 4.0, 4.2, 4.3, 4.4, 4.8, 4.9, 5.0, 5.0, 5.0, 5.0, 5.0, 5.0, 5.0, 5.0, 5.0, 5.0, 5.0, 5.0, 5.0, 5.0, 5.0, 5.0, 5.0, 5.0, 5.0, 5.0, 5.0, 5.0, 5.0, 5.1, 5.2, 5.2, 5.3, 5.4, 5.5, 5.6, 5.8, 5.9, 6.0, 6.0, 6.0, 6.1, 6.2, 6.3, 6.4, 6.5, 6.6, 6.7, 6.9, 7.0, 7.2, 7.3, 7.4, 7.6, 7.8, 8.0, 8.2, 8.4, 8.6, 8.9, 9.1, 9.3, 9.6, 9.8, 10.1, 10.4, 10.7, 11.0, 13.0, 13.4, 13.7, 14.1, 14.5, 15.3, 15.7, 16.1, 16.5, 17.0, 17.4, 17.8, 18.3, 18.7, 19.2, 19.6, 20.1, 20.6, 21.0, 21.5, 22.0, 22.5, 23.0, 23.5, 24.1, 24.6, 25.2, 25.7, 26.3, 26.8, 27.4, 28.0, 28.6, 29.2, 29.8, 30.4, 31.0, 31.7, 32.3, 33.0, 33.6, 34.3, 35.0, 35.6, 36.3, 37.0, 37.7, 38.4, 39.1, 39.8, 40.5, 41.3, 42.0, 42.7, 43.4, 44.2, 44.9, 45.6, 46.3, 47.0, 47.7, 48.5, 49.2, 49.9, 50.6, 51.3, 52.0, 52.7, 53.4, 54.1, 54.8, 55.5, 56.2, 56.9, 57.6, 58.3, 59.0, 59.6, 60.3, 61.0, 61.7, 62.4, 63.1, 63.8, 64.5, 65.2, 65.9, 66.5, 67.2, 67.9, 68.6, 69.3, 70.0, 70.7, 71.4, 72.0, 72.7, 73.3, 74.0, 74.6, 75.2, 79.9, 80.4, 81.0, 82.1, 82.6, 83.1, 83.7, 84.2, 84.7, 85.2, 85.8, 86.3, 86.8, 87.3, 87.9, 88.4, 88.9, 89.5, 90.0, 90.5, 91.0, 91.4, 91.9, 92.3, 92.8, 93.2, 93.5, 93.9, 94.3, 94.6, 94.9, 95.3, 95.6, 95.9, 96.1, 96.3, 96.5, 96.7, 96.9, 97.0, 97.1, 97.3, 97.4, 97.5, 97.6, 97.7, 97.8, 98.0, 98.0, 98.0, 98.0, 98.0, 98.0, 98.0, 98.0, 98.0, 98.0, 98.0, 98.0, 98.0, 98.0, 98.0, 98.0, 98.0, 98.0, 98.0, 98.0, 98.0, 98.0]
  out "time":dbl[](graph)=[48611074.0, 48677187.0, 48743297.0, 48809408.0, 48875521.0, 48941632.0, 49007743.0, 49073858.0, 49139966.0, 49206079.0, 49272188.0, 49338302.0, 49404411.0, 49470522.0, 49536634.0, 49602745.0, 49668858.0, 49801080.0, 49867191.0, 50131636.0, 50197750.0, 50263866.0, 50329983.0, 50396092.0, 50462203.0, 50792762.0, 50858871.0, 50924983.0, 50991096.0, 51057206.0, 51123317.0, 51189428.0, 51255540.0, 51321651.0, 51387763.0, 51453874.0, 51519986.0, 51586097.0, 51652210.0, 51718320.0, 51784433.0, 51850543.0, 51916654.0, 51982767.0, 52048877.0, 52114990.0, 52181100.0, 52247211.0, 52313322.0, 52379434.0, 52445546.0, 52511660.0, 52577769.0, 52643879.0, 52709991.0, 52776103.0, 52842213.0, 52908325.0, 52974436.0, 53040550.0, 53106660.0, 53238882.0, 53304993.0, 53371105.0, 53635551.0, 53701662.0, 53767776.0, 53833885.0, 53899998.0, 53966107.0, 54032219.0, 54098330.0, 54164443.0, 54230553.0, 54296665.0, 54362776.0, 54428887.0, 54495000.0, 54561112.0, 54627233.0, 54693354.0, 54759468.0, 54825580.0, 54891687.0, 54957798.0, 55023910.0, 55090021.0, 55156133.0, 55222244.0, 55288355.0, 55354468.0, 55420578.0, 55486690.0, 55552801.0, 55618912.0, 55685025.0, 55751135.0, 55817246.0, 55883358.0, 55949470.0, 56015581.0, 56081693.0, 56147805.0, 56213915.0, 56280026.0, 56346138.0, 56412252.0, 56478360.0, 56544472.0, 56610583.0, 56676696.0, 56742810.0, 56808917.0, 56875029.0, 56941140.0, 57007252.0, 57073364.0, 57139474.0, 57205586.0, 57271697.0, 57337809.0, 57403920.0, 57470032.0, 57536143.0, 57602254.0, 57668366.0, 57734478.0, 57800590.0, 58197260.0, 58263372.0, 58329480.0, 58395591.0, 58461702.0, 58593925.0, 58660043.0, 58726158.0, 58792269.0, 58858382.0, 58924492.0, 58990604.0, 59056715.0, 59122826.0, 59188939.0, 59255051.0, 59321161.0, 59387272.0, 59453383.0, 59519495.0, 59585608.0, 59651718.0, 59717829.0, 59783941.0, 59850052.0, 59916164.0, 59982275.0, 60048387.0, 60114498.0, 60180609.0, 60246720.0, 60312838.0, 60378954.0, 60445064.0, 60511176.0, 60577287.0, 60643399.0, 60709515.0, 60775621.0, 60841734.0, 60907845.0, 60973957.0, 61040068.0, 61106181.0, 61172295.0, 61238408.0, 61304522.0, 61370635.0, 61436745.0, 61502857.0, 61568968.0, 61635079.0, 61701191.0, 61767302.0, 61833414.0, 61899525.0, 61965638.0, 62031748.0, 62097859.0, 62163971.0, 62230082.0, 62296194.0, 62362305.0, 62428416.0, 62494528.0, 62560640.0, 62626751.0, 62692862.0, 62758973.0, 62825085.0, 62891196.0, 62957312.0, 63023419.0, 63089530.0, 63155642.0, 63221755.0, 63287867.0, 63353976.0, 63420088.0, 63486199.0, 63552311.0, 63618422.0, 63684533.0, 63750646.0, 63816756.0, 63882867.0, 63948978.0, 64015090.0, 64081205.0, 64147314.0, 64213424.0, 64279536.0, 64345648.0, 64411762.0, 64477871.0, 64543981.0, 64610093.0, 64676204.0, 64742316.0, 64808430.0, 64874538.0, 65403429.0, 65469541.0, 65535653.0, 65667875.0, 65733988.0, 65800098.0, 65866209.0, 65932321.0, 65998434.0, 66064543.0, 66130655.0, 66196766.0, 66262877.0, 66328990.0, 66395100.0, 66461212.0, 66527323.0, 66593434.0, 66659546.0, 66725657.0, 66791769.0, 66857880.0, 66923991.0, 66990107.0, 67056214.0, 67122326.0, 67188437.0, 67254548.0, 67320660.0, 67386771.0, 67452885.0, 67518994.0, 67585105.0, 67651217.0, 67717328.0, 67783439.0, 67849551.0, 67915662.0, 67981774.0, 68047885.0, 68113997.0, 68180108.0, 68246221.0, 68312331.0, 68378442.0, 68444553.0, 68510665.0, 68576776.0, 68642887.0, 68709000.0, 68775110.0, 68841222.0, 68907333.0, 68973445.0, 69039556.0, 69105671.0, 69171781.0, 69237890.0, 69304001.0, 69370115.0, 69436224.0, 69502335.0, 69568447.0, 69634559.0, 69700672.0, 69766781.0, 69832892.0, 69899004.0, 69965115.0]
  out "rssi":dbl[](graph)=[-31.0, -28.0, -31.0, -30.0, -40.0, -40.0, -40.0, -40.0, -40.0, -40.0, -40.0, -40.0, -36.0, -40.0, -40.0, -36.0, -36.0, -36.0, -39.0, -36.0, -38.0, -36.0, -36.0, -36.0, -36.0, -35.0, -35.0, -35.0, -35.0, -35.0, -31.0, -31.0, -31.0, -30.0, -30.0, -31.0, -30.0, -30.0, -31.0, -31.0, -27.0, -26.0, -27.0, -25.0, -27.0, -25.0, -26.0, -25.0, -27.0, -27.0, -25.0, -26.0, -27.0, -27.0, -26.0, -25.0, -27.0, -27.0, -25.0, -27.0, -25.0, -25.0, -25.0, -25.0, -27.0, -27.0, -25.0, -26.0, -27.0, -26.0, -25.0, -25.0, -27.0, -27.0, -27.0, -25.0, -27.0, -27.0, -25.0, -27.0, -27.0, -25.0, -25.0, -25.0, -26.0, -25.0, -27.0, -25.0, -27.0, -26.0, -27.0, -25.0, -25.0, -27.0, -25.0, -26.0, -25.0, -25.0, -27.0, -26.0, -27.0, -27.0, -25.0, -27.0, -28.0, -27.0, -26.0, -27.0, -27.0, -27.0, -25.0, -27.0, -25.0, -25.0, -25.0, -27.0, -26.0, -26.0, -25.0, -26.0, -25.0, -25.0, -26.0, -25.0, -27.0, -26.0, -26.0, -27.0, -26.0, -25.0, -26.0, -26.0, -26.0, -26.0, -26.0, -26.0, -26.0, -25.0, -25.0, -25.0, -25.0, -24.0, -25.0, -26.0, -26.0, -25.0, -25.0, -26.0, -25.0, -26.0, -26.0, -26.0, -25.0, -26.0, -25.0, -26.0, -25.0, -25.0, -26.0, -25.0, -24.0, -25.0, -26.0, -25.0, -26.0, -25.0, -24.0, -26.0, -26.0, -25.0, -26.0, -26.0, -25.0, -26.0, -25.0, -26.0, -26.0, -25.0, -26.0, -24.0, -26.0, -26.0, -25.0, -26.0, -25.0, -26.0, -26.0, -26.0, -25.0, -24.0, -26.0, -26.0, -25.0, -25.0, -26.0, -25.0, -25.0, -26.0, -26.0, -26.0, -19.0, -20.0, -20.0, -20.0, -20.0, -18.0, -18.0, -19.0, -18.0, -18.0, -19.0, -19.0, -18.0, -19.0, -22.0, -21.0, -21.0, -20.0, -20.0, -20.0, -20.0, -20.0, -20.0, -20.0, -20.0, -20.0, -20.0, -20.0, -20.0, -20.0, -20.0, -20.0, -20.0, -20.0, -20.0, -20.0, -20.0, -20.0, -20.0, -20.0, -20.0, -20.0, -20.0, -20.0, -20.0, -20.0, -20.0, -20.0, -20.0, -20.0, -20.0, -20.0, -20.0, -20.0, -20.0, -20.0, -20.0, -20.0, -20.0, -20.0, -20.0, -20.0, -20.0, -20.0, -20.0, -20.0, -20.0, -20.0, -20.0, -20.0, -20.0, -20.0, -20.0, -20.0, -20.0, -20.0, -20.0, -20.0, -20.0, -20.0, -20.0, -20.0, -20.0, -20.0, -20.0, -20.0, -20.0, -20.0, -21.0, -20.0, -20.0, -20.0, -20.0, -20.0, -20.0, -20.0, -20.0, -21.0]
  in  "String":string="b'\\xe4\\xb3#\\xb5r\\x9c' bytearray(b'{\"topic\": \"/battery\", \"value\": 0.0}') {b'\\xe4\\xb3#\\xb5r\\x9c': [-31, 48611074]}\nb'\\xe4\\xb3#\\xb5r\\x9c' bytearray(b'{\"topic\": \"/battery\", \"value\": 0.2}') {b'\\xe4\\xb3#\\xb5r\\x9c': [-28, 48677187]}\nb'\\xe4\\xb3#\\xb5r\\x9c' bytearray(b'{\"topic\": \"/battery\", \"value\": 0.2}') {b'\\xe4\\xb3#\\xb5r\\x9c': [-31, 48743297]}\nb'\\xe4\\xb3#\\xb5r\\x9c' bytearray(b'{\"topic\": \"/battery\", \"value\": 0.7}') {b'\\xe4\\xb3#\\xb5r\\x9c': [-30, 48809408]}\nb'\\xe4\\xb3#\\xb5r\\x9c' bytearray(b'{\"topic\": \"/battery\", \"value\": 1.0}') {b'\\xe4\\xb3#\\xb5r\\x9c': [-40, 48875521]}\nb'\\xe4\\xb3#\\xb5r\\x9c' bytearray(b'{\"topic\": \"/battery\", \"value\": 1.1}') {b'\\xe4\\xb3#\\xb5r\\x9c': [-40, 48941632]}\nb'\\xe4\\xb3#\\xb5r\\x9c' bytearray(b'{\"topic\": \"/battery\", \"value\": 1.2}') {b'\\xe4\\xb3#\\xb5r\\x9c': [-40, 49007743]}\nb'\\xe4\\xb3#\\xb5r\\x9c' bytearray(b'{\"topic\": \"/battery\", \"value\": 1.4}') {b'\\xe4\\xb3#\\xb5r\\x9c': [-40, 49073858]}\nb'\\xe4\\xb3#\\xb5r\\x9c' bytearray(b'{\"topic\": \"/battery\", \"value\": 1.7}') {b'\\xe4\\xb3#\\xb5r\\x9c': [-40, 49139966]}\nb'\\xe4\\xb3#\\xb5r\\x9c' bytearray(b'{\"topic\": \"/battery\", \"value\": 2.0}') {b'\\xe4\\xb3#\\xb5r\\x9c': [-40, 49206079]}\nb'\\xe4\\xb3#\\xb5r\\x9c' bytearray(b'{\"topic\": \"/battery\", \"value\": 2.0}') {b'\\xe4\\xb3#\\xb5r\\x9c': [-40, 49272188]}\nb'\\xe4\\xb3#\\xb5r\\x9c' bytearray(b'{\"topic\": \"/battery\", \"value\": 2.0}') {b'\\xe4\\xb3#\\xb5r\\x9c': [-40, 49338302]}\nb'\\xe4\\xb3#\\xb5r\\x9c' bytearray(b'{\"topic\": \"/battery\", \"value\": 2.0}') {b'\\xe4\\xb3#\\xb5r\\x9c': [-36, 49404411]}\nb'\\xe4\\xb3#\\xb5r\\x9c' bytearray(b'{\"topic\": \"/battery\", \"value\": 2.0}') {b'\\xe4\\xb3#\\xb5r\\x9c': [-40, 49470522]}\nb'\\xe4\\xb3#\\xb5r\\x9c' bytearray(b'{\"topic\": \"/battery\", \"value\": 2.1}') {b'\\xe4\\xb3#\\xb5r\\x9c': [-40, 49536634]}\nb'\\xe4\\xb3#\\xb5r\\x9c' bytearray(b'{\"topic\": \"/battery\", \"value\": 2.1}') {b'\\xe4\\xb3#\\xb5r\\x9c': [-36, 49602745]}\nb'\\xe4\\xb3#\\xb5r\\x9c' bytearray(b'{\"topic\": \"/battery\", \"value\": 2.2}') {b'\\xe4\\xb3#\\xb5r\\x9c': [-36, 49668858]}\nb'\\xe4\\xb3#\\xb5r\\x9c' bytear}') {b'\\xe4\\xb3#\\xb5r\\x9c': [-36, 49734968]}\nb'\\xe4\\xb3#\\xb5r\\x9c' bytearray(b'{\"topic\": \"/battery\", \"value\": 2.3}') {b'\\xe4\\xb3#\\xb5r\\x9c': [-36, 49801080]}\nb'\\xe4\\xb3#\\xb5r\\x9c' bytearray(b'{\"topic\": \"/battery\", \"value\": 2.4}') {b'\\xe4\\xb3#\\xb5r\\x9c': [-39, 49867191]}\nb'\\xe4\\xb3#\\xb5r\\x9c' bytear': [-36, 50065525]}\nb'\\xe4\\xb3#\\xb5r\\x9c' bytearray(b'{\"topic\": \"/battery\", \"value\": 2.8}') {b'\\xe4\\xb3#\\xb5r\\x9c': [-36, 50131636]}\nb'\\xe4\\xb3#\\xb5r\\x9c' bytearray(b'{\"topic\": \"/battery\", \"value\": 2.8}') {b'\\xe4\\xb3#\\xb5r\\x9c': [-38, 50197750]}\nb'\\xe4\\xb3#\\xb5r\\x9c' bytearray(b'{\"topic\": \"/battery\", \"value\": 2.9}') {b'\\xe4\\xb3#\\xb5r\\x9c': [-36, 50263866]}\nb'\\xe4\\xb3#\\xb5r\\x9c' bytearray(b'{\"topic\": \"/battery\", \"value\": 2.9}') {b'\\xe4\\xb3#\\xb5r\\x9c': [-36, 50329983]}\nb'\\xe4\\xb3#\\xb5r\\x9c' bytearray(b'{\"topic\": \"/battery\", \"value\": 2.9}') {b'\\xe4\\xb3#\\xb5r\\x9c': [-36, 50396092]}\nb'\\xe4\\xb3#\\xb5r\\x9c' bytearray(b'{\"topic\": \"/battery\", \"value\": 3.0}') {b'\\xe4\\xb3#\\xb5r\\x9c': [-36, 50462203]}\nb'\\xe4\\xb3#\\xb5r\\x9c' bytearb'\\xe4\\xb3#\\xb5r\\x9c' bytearray(b'{\"topic\": \"/battery\", \"value\": 3.0}') {b'\\xe4\\xb3#\\xb5r\\x9c': [-35, 50792762]}\nb'\\xe4\\xb3#\\xb5r\\x9c' bytearray(b'{\"topic\": \"/battery\", \"value\": 2.9}') {b'\\xe4\\xb3#\\xb5r\\x9c': [-35, 50858871]}\nb'\\xe4\\xb3#\\xb5r\\x9c' bytearray(b'{\"topic\": \"/battery\", \"value\": 3.0}') {b'\\xe4\\xb3#\\xb5r\\x9c': [-35, 50924983]}\nb'\\xe4\\xb3#\\xb5r\\x9c' bytearray(b'{\"topic\": \"/battery\", \"value\": 3.0}') {b'\\xe4\\xb3#\\xb5r\\x9c': [-35, 50991096]}\nb'\\xe4\\xb3#\\xb5r\\x9c' bytearray(b'{\"topic\": \"/battery\", \"value\": 3.0}') {b'\\xe4\\xb3#\\xb5r\\x9c': [-35, 51057206]}\nb'\\xe4\\xb3#\\xb5r\\x9c' bytearray(b'{\"topic\": \"/battery\", \"value\": 3.0}') {b'\\xe4\\xb3#\\xb5r\\x9c': [-31, 51123317]}\nb'\\xe4\\xb3#\\xb5r\\x9c' bytearray(b'{\"topic\": \"/battery\", \"value\": 3.0}') {b'\\xe4\\xb3#\\xb5r\\x9c': [-31, 51189428]}\nb'\\xe4\\xb3#\\xb5r\\x9c' bytearray(b'{\"topic\": \"/battery\", \"value\": 3.0}') {b'\\xe4\\xb3#\\xb5r\\x9c': [-31, 51255540]}\nb'\\xe4\\xb3#\\xb5r\\x9c' bytearray(b'{\"topic\": \"/battery\", \"value\": 3.0}') {b'\\xe4\\xb3#\\xb5r\\x9c': [-30, 51321651]}\nb'\\xe4\\xb3#\\xb5r\\x9c' bytearray(b'{\"topic\": \"/battery\", \"value\": 3.0}') {b'\\xe4\\xb3#\\xb5r\\x9c': [-30, 51387763]}\nb'\\xe4\\xb3#\\xb5r\\x9c' bytearray(b'{\"topic\": \"/battery\", \"value\": 3.0}') {b'\\xe4\\xb3#\\xb5r\\x9c': [-31, 51453874]}\nb'\\xe4\\xb3#\\xb5r\\x9c' bytearray(b'{\"topic\": \"/battery\", \"value\": 3.0}') {b'\\xe4\\xb3#\\xb5r\\x9c': [-30, 51519986]}\nb'\\xe4\\xb3#\\xb5r\\x9c' bytearray(b'{\"topic\": \"/battery\", \"value\": 3.0}') {b'\\xe4\\xb3#\\xb5r\\x9c': [-30, 51586097]}\nb'\\xe4\\xb3#\\xb5r\\x9c' bytearray(b'{\"topic\": \"/battery\", \"value\": 3.1}') {b'\\xe4\\xb3#\\xb5r\\x9c': [-31, 51652210]}\nb'\\xe4\\xb3#\\xb5r\\x9c' bytearray(b'{\"topic\": \"/battery\", \"value\": 3.1}') {b'\\xe4\\xb3#\\xb5r\\x9c': [-31, 51718320]}\nb'\\xe4\\xb3#\\xb5r\\x9c' bytearray(b'{\"topic\": \"/battery\", \"value\": 3.2}') {b'\\xe4\\xb3#\\xb5r\\x9c': [-27, 51784433]}\nb'\\xe4\\xb3#\\xb5r\\x9c' bytearray(b'{\"topic\": \"/battery\", \"value\": 3.3}') {b'\\xe4\\xb3#\\xb5r\\x9c': [-26, 51850543]}\nb'\\xe4\\xb3#\\xb5r\\x9c' bytearray(b'{\"topic\": \"/battery\", \"value\": 3.5}') {b'\\xe4\\xb3#\\xb5r\\x9c': [-27, 51916654]}\nb'\\xe4\\xb3#\\xb5r\\x9c' bytearray(b'{\"topic\": \"/battery\", \"value\": 3.6}') {b'\\xe4\\xb3#\\xb5r\\x9c': [-25, 51982767]}\nb'\\xe4\\xb3#\\xb5r\\x9c' bytearray(b'{\"topic\": \"/battery\", \"value\": 3.7}') {b'\\xe4\\xb3#\\xb5r\\x9c': [-27, 52048877]}\nb'\\xe4\\xb3#\\xb5r\\x9c' bytearray(b'{\"topic\": \"/battery\", \"value\": 3.9}') {b'\\xe4\\xb3#\\xb5r\\x9c': [-25, 52114990]}\nb'\\xe4\\xb3#\\xb5r\\x9c' bytearray(b'{\"topic\": \"/battery\", \"value\": 4.0}') {b'\\xe4\\xb3#\\xb5r\\x9c': [-26, 52181100]}\nb'\\xe4\\xb3#\\xb5r\\x9c' bytearray(b'{\"topic\": \"/battery\", \"value\": 4.0}') {b'\\xe4\\xb3#\\xb5r\\x9c': [-25, 52247211]}\nb'\\xe4\\xb3#\\xb5r\\x9c' bytearray(b'{\"topic\": \"/battery\", \"value\": 4.0}') {b'\\xe4\\xb3#\\xb5r\\x9c': [-27, 52313322]}\nb'\\xe4\\xb3#\\xb5r\\x9c' bytearray(b'{\"topic\": \"/battery\", \"value\": 4.0}') {b'\\xe4\\xb3#\\xb5r\\x9c': [-27, 52379434]}\nb'\\xe4\\xb3#\\xb5r\\x9c' bytearray(b'{\"topic\": \"/battery\", \"value\": 4.0}') {b'\\xe4\\xb3#\\xb5r\\x9c': [-25, 52445546]}\nb'\\xe4\\xb3#\\xb5r\\x9c' bytearray(b'{\"topic\": \"/battery\", \"value\": 4.0}') {b'\\xe4\\xb3#\\xb5r\\x9c': [-26, 52511660]}\nb'\\xe4\\xb3#\\xb5r\\x9c' bytearray(b'{\"topic\": \"/battery\", \"value\": 4.0}') {b'\\xe4\\xb3#\\xb5r\\x9c': [-27, 52577769]}\nb'\\xe4\\xb3#\\xb5r\\x9c' bytearray(b'{\"topic\": \"/battery\", \"value\": 4.0}') {b'\\xe4\\xb3#\\xb5r\\x9c': [-27, 52643879]}\nb'\\xe4\\xb3#\\xb5r\\x9c' bytearray(b'{\"topic\": \"/battery\", \"value\": 4.0}') {b'\\xe4\\xb3#\\xb5r\\x9c': [-26, 52709991]}\nb'\\xe4\\xb3#\\xb5r\\x9c' bytearray(b'{\"topic\": \"/battery\", \"value\": 4.0}') {b'\\xe4\\xb3#\\xb5r\\x9c': [-25, 52776103]}\nb'\\xe4\\xb3#\\xb5r\\x9c' bytearray(b'{\"topic\": \"/battery\", \"value\": 4.0}') {b'\\xe4\\xb3#\\xb5r\\x9c': [-27, 52842213]}\nb'\\xe4\\xb3#\\xb5r\\x9c' bytearray(b'{\"topic\": \"/battery\", \"value\": 4.0}') {b'\\xe4\\xb3#\\xb5r\\x9c': [-27, 52908325]}\nb'\\xe4\\xb3#\\xb5r\\x9c' bytearray(b'{\"topic\": \"/battery\", \"value\": 4.0}') {b'\\xe4\\xb3#\\xb5r\\x9c': [-25, 52974436]}\nb'\\xe4\\xb3#\\xb5r\\x9c' bytearray(b'{\"topic\": \"/battery\", \"value\": 4.0}') {b'\\xe4\\xb3#\\xb5r\\x9c': [-27, 53040550]}\nb'\\xe4\\xb3#\\xb5r\\x9c' bytearray(b'{\"topic\": \"/battery\", \"value\": 4.0}') {b'\\xe4\\xb3#\\xb5r\\x9c': [-25, 53106660]}\nb'\\xe4\\xb3#\\xb5r\\x9c' bytearb'\\xe4\\xb3#\\xb5r\\x9c' bytearray(b'{\"topic\": \"/battery\", \"value\": 4.2}') {b'\\xe4\\xb3#\\xb5r\\x9c': [-25, 53238882]}\nb'\\xe4\\xb3#\\xb5r\\x9c' bytearray(b'{\"topic\": \"/battery\", \"value\": 4.3}') {b'\\xe4\\xb3#\\xb5r\\x9c': [-25, 53304993]}\nb'\\xe4\\xb3#\\xb5r\\x9c' bytearray(b'{\"topic\": \"/battery\", \"value\": 4.4}') {b'\\xe4\\xb3#\\xb5r\\x9c': [-25, 53371105]}\nb'\\xe4\\xb3#\\xb5r\\x9c' bytearpic\": \"/battery\", \"value\": 4.8}') {b'\\xe4\\xb3#\\xb5r\\x9c': [-27, 53635551]}\nb'\\xe4\\xb3#\\xb5r\\x9c' bytearray(b'{\"topic\": \"/battery\", \"value\": 4.9}') {b'\\xe4\\xb3#\\xb5r\\x9c': [-27, 53701662]}\nb'\\xe4\\xb3#\\xb5r\\x9c' bytearray(b'{\"topic\": \"/battery\", \"value\": 5.0}') {b'\\xe4\\xb3#\\xb5r\\x9c': [-25, 53767776]}\nb'\\xe4\\xb3#\\xb5r\\x9c' bytearray(b'{\"topic\": \"/battery\", \"value\": 5.0}') {b'\\xe4\\xb3#\\xb5r\\x9c': [-26, 53833885]}\nb'\\xe4\\xb3#\\xb5r\\x9c' bytearray(b'{\"topic\": \"/battery\", \"value\": 5.0}') {b'\\xe4\\xb3#\\xb5r\\x9c': [-27, 53899998]}\nb'\\xe4\\xb3#\\xb5r\\x9c' bytearray(b'{\"topic\": \"/battery\", \"value\": 5.0}') {b'\\xe4\\xb3#\\xb5r\\x9c': [-26, 53966107]}\nb'\\xe4\\xb3#\\xb5r\\x9c' bytearray(b'{\"topic\": \"/battery\", \"value\": 5.0}') {b'\\xe4\\xb3#\\xb5r\\x9c': [-25, 54032219]}\nb'\\xe4\\xb3#\\xb5r\\x9c' bytearray(b'{\"topic\": \"/battery\", \"value\": 5.0}') {b'\\xe4\\xb3#\\xb5r\\x9c': [-25, 54098330]}\nb'\\xe4\\xb3#\\xb5r\\x9c' bytearray(b'{\"topic\": \"/battery\", \"value\": 5.0}') {b'\\xe4\\xb3#\\xb5r\\x9c': [-27, 54164443]}\nb'\\xe4\\xb3#\\xb5r\\x9c' bytearray(b'{\"topic\": \"/battery\", \"value\": 5.0}') {b'\\xe4\\xb3#\\xb5r\\x9c': [-27, 54230553]}\nb'\\xe4\\xb3#\\xb5r\\x9c' bytearray(b'{\"topic\": \"/battery\", \"value\": 5.0}') {b'\\xe4\\xb3#\\xb5r\\x9c': [-27, 54296665]}\nb'\\xe4\\xb3#\\xb5r\\x9c' bytearray(b'{\"topic\": \"/battery\", \"value\": 5.0}') {b'\\xe4\\xb3#\\xb5r\\x9c': [-25, 54362776]}\nb'\\xe4\\xb3#\\xb5r\\x9c' bytearray(b'{\"topic\": \"/battery\", \"value\": 5.0}') {b'\\xe4\\xb3#\\xb5r\\x9c': [-27, 54428887]}\nb'\\xe4\\xb3#\\xb5r\\x9c' bytearray(b'{\"topic\": \"/battery\", \"value\": 5.0}') {b'\\xe4\\xb3#\\xb5r\\x9c': [-27, 54495000]}\nb'\\xe4\\xb3#\\xb5r\\x9c' bytearray(b'{\"topic\": \"/battery\", \"value\": 5.0}') {b'\\xe4\\xb3#\\xb5r\\x9c': [-25, 54561112]}\nb'\\xe4\\xb3#\\xb5r\\x9c' bytearray(b'{\"topic\": \"/battery\", \"value\": 5.0}') {b'\\xe4\\xb3#\\xb5r\\x9c': [-27, 54627233]}\nb'\\xe4\\xb3#\\xb5r\\x9c' bytearray(b'{\"topic\": \"/battery\", \"value\": 5.0}') {b'\\xe4\\xb3#\\xb5r\\x9c': [-27, 54693354]}\nb'\\xe4\\xb3#\\xb5r\\x9c' bytearray(b'{\"topic\": \"/battery\", \"value\": 5.0}') {b'\\xe4\\xb3#\\xb5r\\x9c': [-25, 54759468]}\nb'\\xe4\\xb3#\\xb5r\\x9c' bytearray(b'{\"topic\": \"/battery\", \"value\": 5.0}') {b'\\xe4\\xb3#\\xb5r\\x9c': [-25, 54825580]}\nb'\\xe4\\xb3#\\xb5r\\x9c' bytearray(b'{\"topic\": \"/battery\", \"value\": 5.0}') {b'\\xe4\\xb3#\\xb5r\\x9c': [-25, 54891687]}\nb'\\xe4\\xb3#\\xb5r\\x9c' bytearray(b'{\"topic\": \"/battery\", \"value\": 5.0}') {b'\\xe4\\xb3#\\xb5r\\x9c': [-26, 54957798]}\nb'\\xe4\\xb3#\\xb5r\\x9c' bytearray(b'{\"topic\": \"/battery\", \"value\": 5.0}') {b'\\xe4\\xb3#\\xb5r\\x9c': [-25, 55023910]}\nb'\\xe4\\xb3#\\xb5r\\x9c' bytearray(b'{\"topic\": \"/battery\", \"value\": 5.0}') {b'\\xe4\\xb3#\\xb5r\\x9c': [-27, 55090021]}\nb'\\xe4\\xb3#\\xb5r\\x9c' bytearray(b'{\"topic\": \"/battery\", \"value\": 5.0}') {b'\\xe4\\xb3#\\xb5r\\x9c': [-25, 55156133]}\nb'\\xe4\\xb3#\\xb5r\\x9c' bytearray(b'{\"topic\": \"/battery\", \"value\": 5.0}') {b'\\xe4\\xb3#\\xb5r\\x9c': [-27, 55222244]}\nb'\\xe4\\xb3#\\xb5r\\x9c' bytearray(b'{\"topic\": \"/battery\", \"value\": 5.1}') {b'\\xe4\\xb3#\\xb5r\\x9c': [-26, 55288355]}\nb'\\xe4\\xb3#\\xb5r\\x9c' bytearray(b'{\"topic\": \"/battery\", \"value\": 5.2}') {b'\\xe4\\xb3#\\xb5r\\x9c': [-27, 55354468]}\nb'\\xe4\\xb3#\\xb5r\\x9c' bytearray(b'{\"topic\": \"/battery\", \"value\": 5.2}') {b'\\xe4\\xb3#\\xb5r\\x9c': [-25, 55420578]}\nb'\\xe4\\xb3#\\xb5r\\x9c' bytearray(b'{\"topic\": \"/battery\", \"value\": 5.3}') {b'\\xe4\\xb3#\\xb5r\\x9c': [-25, 55486690]}\nb'\\xe4\\xb3#\\xb5r\\x9c' bytearray(b'{\"topic\": \"/battery\", \"value\": 5.4}') {b'\\xe4\\xb3#\\xb5r\\x9c': [-27, 55552801]}\nb'\\xe4\\xb3#\\xb5r\\x9c' bytearray(b'{\"topic\": \"/battery\", \"value\": 5.5}') {b'\\xe4\\xb3#\\xb5r\\x9c': [-25, 55618912]}\nb'\\xe4\\xb3#\\xb5r\\x9c' bytearray(b'{\"topic\": \"/battery\", \"value\": 5.6}') {b'\\xe4\\xb3#\\xb5r\\x9c': [-26, 55685025]}\nb'\\xe4\\xb3#\\xb5r\\x9c' bytearray(b'{\"topic\": \"/battery\", \"value\": 5.8}') {b'\\xe4\\xb3#\\xb5r\\x9c': [-25, 55751135]}\nb'\\xe4\\xb3#\\xb5r\\x9c' bytearray(b'{\"topic\": \"/battery\", \"value\": 5.9}') {b'\\xe4\\xb3#\\xb5r\\x9c': [-25, 55817246]}\nb'\\xe4\\xb3#\\xb5r\\x9c' bytearray(b'{\"topic\": \"/battery\", \"value\": 6.0}') {b'\\xe4\\xb3#\\xb5r\\x9c': [-27, 55883358]}\nb'\\xe4\\xb3#\\xb5r\\x9c' bytearray(b'{\"topic\": \"/battery\", \"value\": 6.0}') {b'\\xe4\\xb3#\\xb5r\\x9c': [-26, 55949470]}\nb'\\xe4\\xb3#\\xb5r\\x9c' bytearray(b'{\"topic\": \"/battery\", \"value\": 6.0}') {b'\\xe4\\xb3#\\xb5r\\x9c': [-27, 56015581]}\nb'\\xe4\\xb3#\\xb5r\\x9c' bytearray(b'{\"topic\": \"/battery\", \"value\": 6.1}') {b'\\xe4\\xb3#\\xb5r\\x9c': [-27, 56081693]}\nb'\\xe4\\xb3#\\xb5r\\x9c' bytearray(b'{\"topic\": \"/battery\", \"value\": 6.2}') {b'\\xe4\\xb3#\\xb5r\\x9c': [-25, 56147805]}\nb'\\xe4\\xb3#\\xb5r\\x9c' bytearray(b'{\"topic\": \"/battery\", \"value\": 6.3}') {b'\\xe4\\xb3#\\xb5r\\x9c': [-27, 56213915]}\nb'\\xe4\\xb3#\\xb5r\\x9c' bytearray(b'{\"topic\": \"/battery\", \"value\": 6.4}') {b'\\xe4\\xb3#\\xb5r\\x9c': [-28, 56280026]}\nb'\\xe4\\xb3#\\xb5r\\x9c' bytearray(b'{\"topic\": \"/battery\", \"value\": 6.5}') {b'\\xe4\\xb3#\\xb5r\\x9c': [-27, 56346138]}\nb'\\xe4\\xb3#\\xb5r\\x9c' bytearray(b'{\"topic\": \"/battery\", \"value\": 6.6}') {b'\\xe4\\xb3#\\xb5r\\x9c': [-26, 56412252]}\nb'\\xe4\\xb3#\\xb5r\\x9c' bytearray(b'{\"topic\": \"/battery\", \"value\": 6.7}') {b'\\xe4\\xb3#\\xb5r\\x9c': [-27, 56478360]}\nb'\\xe4\\xb3#\\xb5r\\x9c' bytearray(b'{\"topic\": \"/battery\", \"value\": 6.9}') {b'\\xe4\\xb3#\\xb5r\\x9c': [-27, 56544472]}\nb'\\xe4\\xb3#\\xb5r\\x9c' bytearray(b'{\"topic\": \"/battery\", \"value\": 7.0}') {b'\\xe4\\xb3#\\xb5r\\x9c': [-27, 56610583]}\nb'\\xe4\\xb3#\\xb5r\\x9c' bytearray(b'{\"topic\": \"/battery\", \"value\": 7.2}') {b'\\xe4\\xb3#\\xb5r\\x9c': [-25, 56676696]}\nb'\\xe4\\xb3#\\xb5r\\x9c' bytearray(b'{\"topic\": \"/battery\", \"value\": 7.3}') {b'\\xe4\\xb3#\\xb5r\\x9c': [-27, 56742810]}\nb'\\xe4\\xb3#\\xb5r\\x9c' bytearray(b'{\"topic\": \"/battery\", \"value\": 7.4}') {b'\\xe4\\xb3#\\xb5r\\x9c': [-25, 56808917]}\nb'\\xe4\\xb3#\\xb5r\\x9c' bytearray(b'{\"topic\": \"/battery\", \"value\": 7.6}') {b'\\xe4\\xb3#\\xb5r\\x9c': [-25, 56875029]}\nb'\\xe4\\xb3#\\xb5r\\x9c' bytearray(b'{\"topic\": \"/battery\", \"value\": 7.8}') {b'\\xe4\\xb3#\\xb5r\\x9c': [-25, 56941140]}\nb'\\xe4\\xb3#\\xb5r\\x9c' bytearray(b'{\"topic\": \"/battery\", \"value\": 8.0}') {b'\\xe4\\xb3#\\xb5r\\x9c': [-27, 57007252]}\nb'\\xe4\\xb3#\\xb5r\\x9c' bytearray(b'{\"topic\": \"/battery\", \"value\": 8.2}') {b'\\xe4\\xb3#\\xb5r\\x9c': [-26, 57073364]}\nb'\\xe4\\xb3#\\xb5r\\x9c' bytearray(b'{\"topic\": \"/battery\", \"value\": 8.4}') {b'\\xe4\\xb3#\\xb5r\\x9c': [-26, 57139474]}\nb'\\xe4\\xb3#\\xb5r\\x9c' bytearray(b'{\"topic\": \"/battery\", \"value\": 8.6}') {b'\\xe4\\xb3#\\xb5r\\x9c': [-25, 57205586]}\nb'\\xe4\\xb3#\\xb5r\\x9c' bytearray(b'{\"topic\": \"/battery\", \"value\": 8.9}') {b'\\xe4\\xb3#\\xb5r\\x9c': [-26, 57271697]}\nb'\\xe4\\xb3#\\xb5r\\x9c' bytearray(b'{\"topic\": \"/battery\", \"value\": 9.1}') {b'\\xe4\\xb3#\\xb5r\\x9c': [-25, 57337809]}\nb'\\xe4\\xb3#\\xb5r\\x9c' bytearray(b'{\"topic\": \"/battery\", \"value\": 9.3}') {b'\\xe4\\xb3#\\xb5r\\x9c': [-25, 57403920]}\nb'\\xe4\\xb3#\\xb5r\\x9c' bytearray(b'{\"topic\": \"/battery\", \"value\": 9.6}') {b'\\xe4\\xb3#\\xb5r\\x9c': [-26, 57470032]}\nb'\\xe4\\xb3#\\xb5r\\x9c' bytearray(b'{\"topic\": \"/battery\", \"value\": 9.8}') {b'\\xe4\\xb3#\\xb5r\\x9c': [-25, 57536143]}\nb'\\xe4\\xb3#\\xb5r\\x9c' bytearray(b'{\"topic\": \"/battery\", \"value\": 10.1}') {b'\\xe4\\xb3#\\xb5r\\x9c': [-27, 57602254]}\nb'\\xe4\\xb3#\\xb5r\\x9c' bytearray(b'{\"topic\": \"/battery\", \"value\": 10.4}') {b'\\xe4\\xb3#\\xb5r\\x9c': [-26, 57668366]}\nb'\\xe4\\xb3#\\xb5r\\x9c' bytearray(b'{\"topic\": \"/battery\", \"value\": 10.7}') {b'\\xe4\\xb3#\\xb5r\\x9c': [-26, 57734478]}\nb'\\xe4\\xb3#\\xb5r\\x9c' bytearray(b'{\"topic\": \"/battery\", \"value\": 11.0}') {b'\\xe4\\xb3#\\xb5r\\x9c': [-27, 57800590]}\nb'\\xe4\\xb3#\\xb5r\\x9c' byteb'\\xe4\\xb3#\\xb5r\\x9c' bytearray(b'{\"topic\": \"/battery\", \"value\": 13.0}') {b'\\xe4\\xb3#\\xb5r\\x9c': [-26, 58197260]}\nb'\\xe4\\xb3#\\xb5r\\x9c' bytearray(b'{\"topic\": \"/battery\", \"value\": 13.4}') {b'\\xe4\\xb3#\\xb5r\\x9c': [-25, 58263372]}\nb'\\xe4\\xb3#\\xb5r\\x9c' bytearray(b'{\"topic\": \"/battery\", \"value\": 13.7}') {b'\\xe4\\xb3#\\xb5r\\x9c': [-26, 58329480]}\nb'\\xe4\\xb3#\\xb5r\\x9c' bytearray(b'{\"topic\": \"/battery\", \"value\": 14.1}') {b'\\xe4\\xb3#\\xb5r\\x9c': [-26, 58395591]}\nb'\\xe4\\xb3#\\xb5r\\x9c' bytearray(b'{\"topic\": \"/battery\", \"value\": 14.5}') {b'\\xe4\\xb3#\\xb5r\\x9c': [-26, 58461702]}\nb'\\xe4\\xb3#\\xb5r\\x9c' byteb'\\xe4\\xb3#\\xb5r\\x9c' bytearray(b'{\"topic\": \"/battery\", \"value\": 15.3}') {b'\\xe4\\xb3#\\xb5r\\x9c': [-26, 58593925]}\nb'\\xe4\\xb3#\\xb5r\\x9c' bytearray(b'{\"topic\": \"/battery\", \"value\": 15.7}') {b'\\xe4\\xb3#\\xb5r\\x9c': [-26, 58660043]}\nb'\\xe4\\xb3#\\xb5r\\x9c' bytearray(b'{\"topic\": \"/battery\", \"value\": 16.1}') {b'\\xe4\\xb3#\\xb5r\\x9c': [-26, 58726158]}\nb'\\xe4\\xb3#\\xb5r\\x9c' bytearray(b'{\"topic\": \"/battery\", \"value\": 16.5}') {b'\\xe4\\xb3#\\xb5r\\x9c': [-26, 58792269]}\nb'\\xe4\\xb3#\\xb5r\\x9c' bytearray(b'{\"topic\": \"/battery\", \"value\": 17.0}') {b'\\xe4\\xb3#\\xb5r\\x9c': [-25, 58858382]}\nb'\\xe4\\xb3#\\xb5r\\x9c' bytearray(b'{\"topic\": \"/battery\", \"value\": 17.4}') {b'\\xe4\\xb3#\\xb5r\\x9c': [-25, 58924492]}\nb'\\xe4\\xb3#\\xb5r\\x9c' bytearray(b'{\"topic\": \"/battery\", \"value\": 17.8}') {b'\\xe4\\xb3#\\xb5r\\x9c': [-25, 58990604]}\nb'\\xe4\\xb3#\\xb5r\\x9c' bytearray(b'{\"topic\": \"/battery\", \"value\": 18.3}') {b'\\xe4\\xb3#\\xb5r\\x9c': [-25, 59056715]}\nb'\\xe4\\xb3#\\xb5r\\x9c' bytearray(b'{\"topic\": \"/battery\", \"value\": 18.7}') {b'\\xe4\\xb3#\\xb5r\\x9c': [-24, 59122826]}\nb'\\xe4\\xb3#\\xb5r\\x9c' bytearray(b'{\"topic\": \"/battery\", \"value\": 19.2}') {b'\\xe4\\xb3#\\xb5r\\x9c': [-25, 59188939]}\nb'\\xe4\\xb3#\\xb5r\\x9c' bytearray(b'{\"topic\": \"/battery\", \"value\": 19.6}') {b'\\xe4\\xb3#\\xb5r\\x9c': [-26, 59255051]}\nb'\\xe4\\xb3#\\xb5r\\x9c' bytearray(b'{\"topic\": \"/battery\", \"value\": 20.1}') {b'\\xe4\\xb3#\\xb5r\\x9c': [-26, 59321161]}\nb'\\xe4\\xb3#\\xb5r\\x9c' bytearray(b'{\"topic\": \"/battery\", \"value\": 20.6}') {b'\\xe4\\xb3#\\xb5r\\x9c': [-25, 59387272]}\nb'\\xe4\\xb3#\\xb5r\\x9c' bytearray(b'{\"topic\": \"/battery\", \"value\": 21.0}') {b'\\xe4\\xb3#\\xb5r\\x9c': [-25, 59453383]}\nb'\\xe4\\xb3#\\xb5r\\x9c' bytearray(b'{\"topic\": \"/battery\", \"value\": 21.5}') {b'\\xe4\\xb3#\\xb5r\\x9c': [-26, 59519495]}\nb'\\xe4\\xb3#\\xb5r\\x9c' bytearray(b'{\"topic\": \"/battery\", \"value\": 22.0}') {b'\\xe4\\xb3#\\xb5r\\x9c': [-25, 59585608]}\nb'\\xe4\\xb3#\\xb5r\\x9c' bytearray(b'{\"topic\": \"/battery\", \"value\": 22.5}') {b'\\xe4\\xb3#\\xb5r\\x9c': [-26, 59651718]}\nb'\\xe4\\xb3#\\xb5r\\x9c' bytearray(b'{\"topic\": \"/battery\", \"value\": 23.0}') {b'\\xe4\\xb3#\\xb5r\\x9c': [-26, 59717829]}\nb'\\xe4\\xb3#\\xb5r\\x9c' bytearray(b'{\"topic\": \"/battery\", \"value\": 23.5}') {b'\\xe4\\xb3#\\xb5r\\x9c': [-26, 59783941]}\nb'\\xe4\\xb3#\\xb5r\\x9c' bytearray(b'{\"topic\": \"/battery\", \"value\": 24.1}') {b'\\xe4\\xb3#\\xb5r\\x9c': [-25, 59850052]}\nb'\\xe4\\xb3#\\xb5r\\x9c' bytearray(b'{\"topic\": \"/battery\", \"value\": 24.6}') {b'\\xe4\\xb3#\\xb5r\\x9c': [-26, 59916164]}\nb'\\xe4\\xb3#\\xb5r\\x9c' bytearray(b'{\"topic\": \"/battery\", \"value\": 25.2}') {b'\\xe4\\xb3#\\xb5r\\x9c': [-25, 59982275]}\nb'\\xe4\\xb3#\\xb5r\\x9c' bytearray(b'{\"topic\": \"/battery\", \"value\": 25.7}') {b'\\xe4\\xb3#\\xb5r\\x9c': [-26, 60048387]}\nb'\\xe4\\xb3#\\xb5r\\x9c' bytearray(b'{\"topic\": \"/battery\", \"value\": 26.3}') {b'\\xe4\\xb3#\\xb5r\\x9c': [-25, 60114498]}\nb'\\xe4\\xb3#\\xb5r\\x9c' bytearray(b'{\"topic\": \"/battery\", \"value\": 26.8}') {b'\\xe4\\xb3#\\xb5r\\x9c': [-25, 60180609]}\nb'\\xe4\\xb3#\\xb5r\\x9c' bytearray(b'{\"topic\": \"/battery\", \"value\": 27.4}') {b'\\xe4\\xb3#\\xb5r\\x9c': [-26, 60246720]}\nb'\\xe4\\xb3#\\xb5r\\x9c' bytearray(b'{\"topic\": \"/battery\", \"value\": 28.0}') {b'\\xe4\\xb3#\\xb5r\\x9c': [-25, 60312838]}\nb'\\xe4\\xb3#\\xb5r\\x9c' bytearray(b'{\"topic\": \"/battery\", \"value\": 28.6}') {b'\\xe4\\xb3#\\xb5r\\x9c': [-24, 60378954]}\nb'\\xe4\\xb3#\\xb5r\\x9c' bytearray(b'{\"topic\": \"/battery\", \"value\": 29.2}') {b'\\xe4\\xb3#\\xb5r\\x9c': [-25, 60445064]}\nb'\\xe4\\xb3#\\xb5r\\x9c' bytearray(b'{\"topic\": \"/battery\", \"value\": 29.8}') {b'\\xe4\\xb3#\\xb5r\\x9c': [-26, 60511176]}\nb'\\xe4\\xb3#\\xb5r\\x9c' bytearray(b'{\"topic\": \"/battery\", \"value\": 30.4}') {b'\\xe4\\xb3#\\xb5r\\x9c': [-25, 60577287]}\nb'\\xe4\\xb3#\\xb5r\\x9c' bytearray(b'{\"topic\": \"/battery\", \"value\": 31.0}') {b'\\xe4\\xb3#\\xb5r\\x9c': [-26, 60643399]}\nb'\\xe4\\xb3#\\xb5r\\x9c' bytearray(b'{\"topic\": \"/battery\", \"value\": 31.7}') {b'\\xe4\\xb3#\\xb5r\\x9c': [-25, 60709515]}\nb'\\xe4\\xb3#\\xb5r\\x9c' bytearray(b'{\"topic\": \"/battery\", \"value\": 32.3}') {b'\\xe4\\xb3#\\xb5r\\x9c': [-24, 60775621]}\nb'\\xe4\\xb3#\\xb5r\\x9c' bytearray(b'{\"topic\": \"/battery\", \"value\": 33.0}') {b'\\xe4\\xb3#\\xb5r\\x9c': [-26, 60841734]}\nb'\\xe4\\xb3#\\xb5r\\x9c' bytearray(b'{\"topic\": \"/battery\", \"value\": 33.6}') {b'\\xe4\\xb3#\\xb5r\\x9c': [-26, 60907845]}\nb'\\xe4\\xb3#\\xb5r\\x9c' bytearray(b'{\"topic\": \"/battery\", \"value\": 34.3}') {b'\\xe4\\xb3#\\xb5r\\x9c': [-25, 60973957]}\nb'\\xe4\\xb3#\\xb5r\\x9c' bytearray(b'{\"topic\": \"/battery\", \"value\": 35.0}') {b'\\xe4\\xb3#\\xb5r\\x9c': [-26, 61040068]}\nb'\\xe4\\xb3#\\xb5r\\x9c' bytearray(b'{\"topic\": \"/battery\", \"value\": 35.6}') {b'\\xe4\\xb3#\\xb5r\\x9c': [-26, 61106181]}\nb'\\xe4\\xb3#\\xb5r\\x9c' bytearray(b'{\"topic\": \"/battery\", \"value\": 36.3}') {b'\\xe4\\xb3#\\xb5r\\x9c': [-25, 61172295]}\nb'\\xe4\\xb3#\\xb5r\\x9c' bytearray(b'{\"topic\": \"/battery\", \"value\": 37.0}') {b'\\xe4\\xb3#\\xb5r\\x9c': [-26, 61238408]}\nb'\\xe4\\xb3#\\xb5r\\x9c' bytearray(b'{\"topic\": \"/battery\", \"value\": 37.7}') {b'\\xe4\\xb3#\\xb5r\\x9c': [-25, 61304522]}\nb'\\xe4\\xb3#\\xb5r\\x9c' bytearray(b'{\"topic\": \"/battery\", \"value\": 38.4}') {b'\\xe4\\xb3#\\xb5r\\x9c': [-26, 61370635]}\nb'\\xe4\\xb3#\\xb5r\\x9c' bytearray(b'{\"topic\": \"/battery\", \"value\": 39.1}') {b'\\xe4\\xb3#\\xb5r\\x9c': [-26, 61436745]}\nb'\\xe4\\xb3#\\xb5r\\x9c' bytearray(b'{\"topic\": \"/battery\", \"value\": 39.8}') {b'\\xe4\\xb3#\\xb5r\\x9c': [-25, 61502857]}\nb'\\xe4\\xb3#\\xb5r\\x9c' bytearray(b'{\"topic\": \"/battery\", \"value\": 40.5}') {b'\\xe4\\xb3#\\xb5r\\x9c': [-26, 61568968]}\nb'\\xe4\\xb3#\\xb5r\\x9c' bytearray(b'{\"topic\": \"/battery\", \"value\": 41.3}') {b'\\xe4\\xb3#\\xb5r\\x9c': [-24, 61635079]}\nb'\\xe4\\xb3#\\xb5r\\x9c' bytearray(b'{\"topic\": \"/battery\", \"value\": 42.0}') {b'\\xe4\\xb3#\\xb5r\\x9c': [-26, 61701191]}\nb'\\xe4\\xb3#\\xb5r\\x9c' bytearray(b'{\"topic\": \"/battery\", \"value\": 42.7}') {b'\\xe4\\xb3#\\xb5r\\x9c': [-26, 61767302]}\nb'\\xe4\\xb3#\\xb5r\\x9c' bytearray(b'{\"topic\": \"/battery\", \"value\": 43.4}') {b'\\xe4\\xb3#\\xb5r\\x9c': [-25, 61833414]}\nb'\\xe4\\xb3#\\xb5r\\x9c' bytearray(b'{\"topic\": \"/battery\", \"value\": 44.2}') {b'\\xe4\\xb3#\\xb5r\\x9c': [-26, 61899525]}\nb'\\xe4\\xb3#\\xb5r\\x9c' bytearray(b'{\"topic\": \"/battery\", \"value\": 44.9}') {b'\\xe4\\xb3#\\xb5r\\x9c': [-25, 61965638]}\nb'\\xe4\\xb3#\\xb5r\\x9c' bytearray(b'{\"topic\": \"/battery\", \"value\": 45.6}') {b'\\xe4\\xb3#\\xb5r\\x9c': [-26, 62031748]}\nb'\\xe4\\xb3#\\xb5r\\x9c' bytearray(b'{\"topic\": \"/battery\", \"value\": 46.3}') {b'\\xe4\\xb3#\\xb5r\\x9c': [-26, 62097859]}\nb'\\xe4\\xb3#\\xb5r\\x9c' bytearray(b'{\"topic\": \"/battery\", \"value\": 47.0}') {b'\\xe4\\xb3#\\xb5r\\x9c': [-26, 62163971]}\nb'\\xe4\\xb3#\\xb5r\\x9c' bytearray(b'{\"topic\": \"/battery\", \"value\": 47.7}') {b'\\xe4\\xb3#\\xb5r\\x9c': [-25, 62230082]}\nb'\\xe4\\xb3#\\xb5r\\x9c' bytearray(b'{\"topic\": \"/battery\", \"value\": 48.5}') {b'\\xe4\\xb3#\\xb5r\\x9c': [-24, 62296194]}\nb'\\xe4\\xb3#\\xb5r\\x9c' bytearray(b'{\"topic\": \"/battery\", \"value\": 49.2}') {b'\\xe4\\xb3#\\xb5r\\x9c': [-26, 62362305]}\nb'\\xe4\\xb3#\\xb5r\\x9c' bytearray(b'{\"topic\": \"/battery\", \"value\": 49.9}') {b'\\xe4\\xb3#\\xb5r\\x9c': [-26, 62428416]}\nb'\\xe4\\xb3#\\xb5r\\x9c' bytearray(b'{\"topic\": \"/battery\", \"value\": 50.6}') {b'\\xe4\\xb3#\\xb5r\\x9c': [-25, 62494528]}\nb'\\xe4\\xb3#\\xb5r\\x9c' bytearray(b'{\"topic\": \"/battery\", \"value\": 51.3}') {b'\\xe4\\xb3#\\xb5r\\x9c': [-25, 62560640]}\nb'\\xe4\\xb3#\\xb5r\\x9c' bytearray(b'{\"topic\": \"/battery\", \"value\": 52.0}') {b'\\xe4\\xb3#\\xb5r\\x9c': [-26, 62626751]}\nb'\\xe4\\xb3#\\xb5r\\x9c' bytearray(b'{\"topic\": \"/battery\", \"value\": 52.7}') {b'\\xe4\\xb3#\\xb5r\\x9c': [-25, 62692862]}\nb'\\xe4\\xb3#\\xb5r\\x9c' bytearray(b'{\"topic\": \"/battery\", \"value\": 53.4}') {b'\\xe4\\xb3#\\xb5r\\x9c': [-25, 62758973]}\nb'\\xe4\\xb3#\\xb5r\\x9c' bytearray(b'{\"topic\": \"/battery\", \"value\": 54.1}') {b'\\xe4\\xb3#\\xb5r\\x9c': [-26, 62825085]}\nb'\\xe4\\xb3#\\xb5r\\x9c' bytearray(b'{\"topic\": \"/battery\", \"value\": 54.8}') {b'\\xe4\\xb3#\\xb5r\\x9c': [-26, 62891196]}\nb'\\xe4\\xb3#\\xb5r\\x9c' bytearray(b'{\"topic\": \"/battery\", \"value\": 55.5}') {b'\\xe4\\xb3#\\xb5r\\x9c': [-26, 62957312]}\nb'\\xe4\\xb3#\\xb5r\\x9c' bytearray(b'{\"topic\": \"/battery\", \"value\": 56.2}') {b'\\xe4\\xb3#\\xb5r\\x9c': [-19, 63023419]}\nb'\\xe4\\xb3#\\xb5r\\x9c' bytearray(b'{\"topic\": \"/battery\", \"value\": 56.9}') {b'\\xe4\\xb3#\\xb5r\\x9c': [-20, 63089530]}\nb'\\xe4\\xb3#\\xb5r\\x9c' bytearray(b'{\"topic\": \"/battery\", \"value\": 57.6}') {b'\\xe4\\xb3#\\xb5r\\x9c': [-20, 63155642]}\nb'\\xe4\\xb3#\\xb5r\\x9c' bytearray(b'{\"topic\": \"/battery\", \"value\": 58.3}') {b'\\xe4\\xb3#\\xb5r\\x9c': [-20, 63221755]}\nb'\\xe4\\xb3#\\xb5r\\x9c' bytearray(b'{\"topic\": \"/battery\", \"value\": 59.0}') {b'\\xe4\\xb3#\\xb5r\\x9c': [-20, 63287867]}\nb'\\xe4\\xb3#\\xb5r\\x9c' bytearray(b'{\"topic\": \"/battery\", \"value\": 59.6}') {b'\\xe4\\xb3#\\xb5r\\x9c': [-18, 63353976]}\nb'\\xe4\\xb3#\\xb5r\\x9c' bytearray(b'{\"topic\": \"/battery\", \"value\": 60.3}') {b'\\xe4\\xb3#\\xb5r\\x9c': [-18, 63420088]}\nb'\\xe4\\xb3#\\xb5r\\x9c' bytearray(b'{\"topic\": \"/battery\", \"value\": 61.0}') {b'\\xe4\\xb3#\\xb5r\\x9c': [-19, 63486199]}\nb'\\xe4\\xb3#\\xb5r\\x9c' bytearray(b'{\"topic\": \"/battery\", \"value\": 61.7}') {b'\\xe4\\xb3#\\xb5r\\x9c': [-18, 63552311]}\nb'\\xe4\\xb3#\\xb5r\\x9c' bytearray(b'{\"topic\": \"/battery\", \"value\": 62.4}') {b'\\xe4\\xb3#\\xb5r\\x9c': [-18, 63618422]}\nb'\\xe4\\xb3#\\xb5r\\x9c' bytearray(b'{\"topic\": \"/battery\", \"value\": 63.1}') {b'\\xe4\\xb3#\\xb5r\\x9c': [-19, 63684533]}\nb'\\xe4\\xb3#\\xb5r\\x9c' bytearray(b'{\"topic\": \"/battery\", \"value\": 63.8}') {b'\\xe4\\xb3#\\xb5r\\x9c': [-19, 63750646]}\nb'\\xe4\\xb3#\\xb5r\\x9c' bytearray(b'{\"topic\": \"/battery\", \"value\": 64.5}') {b'\\xe4\\xb3#\\xb5r\\x9c': [-18, 63816756]}\nb'\\xe4\\xb3#\\xb5r\\x9c' bytearray(b'{\"topic\": \"/battery\", \"value\": 65.2}') {b'\\xe4\\xb3#\\xb5r\\x9c': [-19, 63882867]}\nb'\\xe4\\xb3#\\xb5r\\x9c' bytearray(b'{\"topic\": \"/battery\", \"value\": 65.9}') {b'\\xe4\\xb3#\\xb5r\\x9c': [-22, 63948978]}\nb'\\xe4\\xb3#\\xb5r\\x9c' bytearray(b'{\"topic\": \"/battery\", \"value\": 66.5}') {b'\\xe4\\xb3#\\xb5r\\x9c': [-21, 64015090]}\nb'\\xe4\\xb3#\\xb5r\\x9c' bytearray(b'{\"topic\": \"/battery\", \"value\": 67.2}') {b'\\xe4\\xb3#\\xb5r\\x9c': [-21, 64081205]}\nb'\\xe4\\xb3#\\xb5r\\x9c' bytearray(b'{\"topic\": \"/battery\", \"value\": 67.9}') {b'\\xe4\\xb3#\\xb5r\\x9c': [-20, 64147314]}\nb'\\xe4\\xb3#\\xb5r\\x9c' bytearray(b'{\"topic\": \"/battery\", \"value\": 68.6}') {b'\\xe4\\xb3#\\xb5r\\x9c': [-20, 64213424]}\nb'\\xe4\\xb3#\\xb5r\\x9c' bytearray(b'{\"topic\": \"/battery\", \"value\": 69.3}') {b'\\xe4\\xb3#\\xb5r\\x9c': [-20, 64279536]}\nb'\\xe4\\xb3#\\xb5r\\x9c' bytearray(b'{\"topic\": \"/battery\", \"value\": 70.0}') {b'\\xe4\\xb3#\\xb5r\\x9c': [-20, 64345648]}\nb'\\xe4\\xb3#\\xb5r\\x9c' bytearray(b'{\"topic\": \"/battery\", \"value\": 70.7}') {b'\\xe4\\xb3#\\xb5r\\x9c': [-20, 64411762]}\nb'\\xe4\\xb3#\\xb5r\\x9c' bytearray(b'{\"topic\": \"/battery\", \"value\": 71.4}') {b'\\xe4\\xb3#\\xb5r\\x9c': [-20, 64477871]}\nb'\\xe4\\xb3#\\xb5r\\x9c' bytearray(b'{\"topic\": \"/battery\", \"value\": 72.0}') {b'\\xe4\\xb3#\\xb5r\\x9c': [-20, 64543981]}\nb'\\xe4\\xb3#\\xb5r\\x9c' bytearray(b'{\"topic\": \"/battery\", \"value\": 72.7}') {b'\\xe4\\xb3#\\xb5r\\x9c': [-20, 64610093]}\nb'\\xe4\\xb3#\\xb5r\\x9c' bytearray(b'{\"topic\": \"/battery\", \"value\": 73.3}') {b'\\xe4\\xb3#\\xb5r\\x9c': [-20, 64676204]}\nb'\\xe4\\xb3#\\xb5r\\x9c' bytearray(b'{\"topic\": \"/battery\", \"value\": 74.0}') {b'\\xe4\\xb3#\\xb5r\\x9c': [-20, 64742316]}\nb'\\xe4\\xb3#\\xb5r\\x9c' bytearray(b'{\"topic\": \"/battery\", \"value\": 74.6}') {b'\\xe4\\xb3#\\xb5r\\x9c': [-20, 64808430]}\nb'\\xe4\\xb3#\\xb5r\\x9c' bytearray(b'{\"topic\": \"/battery\", \"value\": 75.2}') {b'\\xe4\\xb3#\\xb5r\\x9c': [-20, 64874538]}\nb'\\xe4\\xb3#\\xb5r\\x9c' byteb3#\\xb5r\\x9c' bytearray(b'{\"topic\": \"/battery\", \"value\": 79.9}') {b'\\xe4\\xb3#\\xb5r\\x9c': [-20, 65403429]}\nb'\\xe4\\xb3#\\xb5r\\x9c' bytearray(b'{\"topic\": \"/battery\", \"value\": 80.4}') {b'\\xe4\\xb3#\\xb5r\\x9c': [-20, 65469541]}\nb'\\xe4\\xb3#\\xb5r\\x9c' bytearray(b'{\"topic\": \"/battery\", \"value\": 81.0}') {b'\\xe4\\xb3#\\xb5r\\x9c': [-20, 65535653]}\nb'\\xe4\\xb3#\\xb5r\\x9c' byte\", \"value\": 81.5}') {b'\\xe4\\xb3#\\xb5r\\x9c': [-20, 65601763]}\nb'\\xe4\\xb3#\\xb5r\\x9c' bytearray(b'{\"topic\": \"/battery\", \"value\": 82.1}') {b'\\xe4\\xb3#\\xb5r\\x9c': [-20, 65667875]}\nb'\\xe4\\xb3#\\xb5r\\x9c' bytearray(b'{\"topic\": \"/battery\", \"value\": 82.6}') {b'\\xe4\\xb3#\\xb5r\\x9c': [-20, 65733988]}\nb'\\xe4\\xb3#\\xb5r\\x9c' bytearray(b'{\"topic\": \"/battery\", \"value\": 83.1}') {b'\\xe4\\xb3#\\xb5r\\x9c': [-20, 65800098]}\nb'\\xe4\\xb3#\\xb5r\\x9c' bytearray(b'{\"topic\": \"/battery\", \"value\": 83.7}') {b'\\xe4\\xb3#\\xb5r\\x9c': [-20, 65866209]}\nb'\\xe4\\xb3#\\xb5r\\x9c' bytearray(b'{\"topic\": \"/battery\", \"value\": 84.2}') {b'\\xe4\\xb3#\\xb5r\\x9c': [-20, 65932321]}\nb'\\xe4\\xb3#\\xb5r\\x9c' bytearray(b'{\"topic\": \"/battery\", \"value\": 84.7}') {b'\\xe4\\xb3#\\xb5r\\x9c': [-20, 65998434]}\nb'\\xe4\\xb3#\\xb5r\\x9c' bytearray(b'{\"topic\": \"/battery\", \"value\": 85.2}') {b'\\xe4\\xb3#\\xb5r\\x9c': [-20, 66064543]}\nb'\\xe4\\xb3#\\xb5r\\x9c' bytearray(b'{\"topic\": \"/battery\", \"value\": 85.8}') {b'\\xe4\\xb3#\\xb5r\\x9c': [-20, 66130655]}\nb'\\xe4\\xb3#\\xb5r\\x9c' bytearray(b'{\"topic\": \"/battery\", \"value\": 86.3}') {b'\\xe4\\xb3#\\xb5r\\x9c': [-20, 66196766]}\nb'\\xe4\\xb3#\\xb5r\\x9c' bytearray(b'{\"topic\": \"/battery\", \"value\": 86.8}') {b'\\xe4\\xb3#\\xb5r\\x9c': [-20, 66262877]}\nb'\\xe4\\xb3#\\xb5r\\x9c' bytearray(b'{\"topic\": \"/battery\", \"value\": 87.3}') {b'\\xe4\\xb3#\\xb5r\\x9c': [-20, 66328990]}\nb'\\xe4\\xb3#\\xb5r\\x9c' bytearray(b'{\"topic\": \"/battery\", \"value\": 87.9}') {b'\\xe4\\xb3#\\xb5r\\x9c': [-20, 66395100]}\nb'\\xe4\\xb3#\\xb5r\\x9c' bytearray(b'{\"topic\": \"/battery\", \"value\": 88.4}') {b'\\xe4\\xb3#\\xb5r\\x9c': [-20, 66461212]}\nb'\\xe4\\xb3#\\xb5r\\x9c' bytearray(b'{\"topic\": \"/battery\", \"value\": 88.9}') {b'\\xe4\\xb3#\\xb5r\\x9c': [-20, 66527323]}\nb'\\xe4\\xb3#\\xb5r\\x9c' bytearray(b'{\"topic\": \"/battery\", \"value\": 89.5}') {b'\\xe4\\xb3#\\xb5r\\x9c': [-20, 66593434]}\nb'\\xe4\\xb3#\\xb5r\\x9c' bytearray(b'{\"topic\": \"/battery\", \"value\": 90.0}') {b'\\xe4\\xb3#\\xb5r\\x9c': [-20, 66659546]}\nb'\\xe4\\xb3#\\xb5r\\x9c' bytearray(b'{\"topic\": \"/battery\", \"value\": 90.5}') {b'\\xe4\\xb3#\\xb5r\\x9c': [-20, 66725657]}\nb'\\xe4\\xb3#\\xb5r\\x9c' bytearray(b'{\"topic\": \"/battery\", \"value\": 91.0}') {b'\\xe4\\xb3#\\xb5r\\x9c': [-20, 66791769]}\nb'\\xe4\\xb3#\\xb5r\\x9c' bytearray(b'{\"topic\": \"/battery\", \"value\": 91.4}') {b'\\xe4\\xb3#\\xb5r\\x9c': [-20, 66857880]}\nb'\\xe4\\xb3#\\xb5r\\x9c' bytearray(b'{\"topic\": \"/battery\", \"value\": 91.9}') {b'\\xe4\\xb3#\\xb5r\\x9c': [-20, 66923991]}\nb'\\xe4\\xb3#\\xb5r\\x9c' bytearray(b'{\"topic\": \"/battery\", \"value\": 92.3}') {b'\\xe4\\xb3#\\xb5r\\x9c': [-20, 66990107]}\nb'\\xe4\\xb3#\\xb5r\\x9c' bytearray(b'{\"topic\": \"/battery\", \"value\": 92.8}') {b'\\xe4\\xb3#\\xb5r\\x9c': [-20, 67056214]}\nb'\\xe4\\xb3#\\xb5r\\x9c' bytearray(b'{\"topic\": \"/battery\", \"value\": 93.2}') {b'\\xe4\\xb3#\\xb5r\\x9c': [-20, 67122326]}\nb'\\xe4\\xb3#\\xb5r\\x9c' bytearray(b'{\"topic\": \"/battery\", \"value\": 93.5}') {b'\\xe4\\xb3#\\xb5r\\x9c': [-20, 67188437]}\nb'\\xe4\\xb3#\\xb5r\\x9c' bytearray(b'{\"topic\": \"/battery\", \"value\": 93.9}') {b'\\xe4\\xb3#\\xb5r\\x9c': [-20, 67254548]}\nb'\\xe4\\xb3#\\xb5r\\x9c' bytearray(b'{\"topic\": \"/battery\", \"value\": 94.3}') {b'\\xe4\\xb3#\\xb5r\\x9c': [-20, 67320660]}\nb'\\xe4\\xb3#\\xb5r\\x9c' bytearray(b'{\"topic\": \"/battery\", \"value\": 94.6}') {b'\\xe4\\xb3#\\xb5r\\x9c': [-20, 67386771]}\nb'\\xe4\\xb3#\\xb5r\\x9c' bytearray(b'{\"topic\": \"/battery\", \"value\": 94.9}') {b'\\xe4\\xb3#\\xb5r\\x9c': [-20, 67452885]}\nb'\\xe4\\xb3#\\xb5r\\x9c' bytearray(b'{\"topic\": \"/battery\", \"value\": 95.3}') {b'\\xe4\\xb3#\\xb5r\\x9c': [-20, 67518994]}\nb'\\xe4\\xb3#\\xb5r\\x9c' bytearray(b'{\"topic\": \"/battery\", \"value\": 95.6}') {b'\\xe4\\xb3#\\xb5r\\x9c': [-20, 67585105]}\nb'\\xe4\\xb3#\\xb5r\\x9c' bytearray(b'{\"topic\": \"/battery\", \"value\": 95.9}') {b'\\xe4\\xb3#\\xb5r\\x9c': [-20, 67651217]}\nb'\\xe4\\xb3#\\xb5r\\x9c' bytearray(b'{\"topic\": \"/battery\", \"value\": 96.1}') {b'\\xe4\\xb3#\\xb5r\\x9c': [-20, 67717328]}\nb'\\xe4\\xb3#\\xb5r\\x9c' bytearray(b'{\"topic\": \"/battery\", \"value\": 96.3}') {b'\\xe4\\xb3#\\xb5r\\x9c': [-20, 67783439]}\nb'\\xe4\\xb3#\\xb5r\\x9c' bytearray(b'{\"topic\": \"/battery\", \"value\": 96.5}') {b'\\xe4\\xb3#\\xb5r\\x9c': [-20, 67849551]}\nb'\\xe4\\xb3#\\xb5r\\x9c' bytearray(b'{\"topic\": \"/battery\", \"value\": 96.7}') {b'\\xe4\\xb3#\\xb5r\\x9c': [-20, 67915662]}\nb'\\xe4\\xb3#\\xb5r\\x9c' bytearray(b'{\"topic\": \"/battery\", \"value\": 96.9}') {b'\\xe4\\xb3#\\xb5r\\x9c': [-20, 67981774]}\nb'\\xe4\\xb3#\\xb5r\\x9c' bytearray(b'{\"topic\": \"/battery\", \"value\": 97.0}') {b'\\xe4\\xb3#\\xb5r\\x9c': [-20, 68047885]}\nb'\\xe4\\xb3#\\xb5r\\x9c' bytearray(b'{\"topic\": \"/battery\", \"value\": 97.1}') {b'\\xe4\\xb3#\\xb5r\\x9c': [-20, 68113997]}\nb'\\xe4\\xb3#\\xb5r\\x9c' bytearray(b'{\"topic\": \"/battery\", \"value\": 97.3}') {b'\\xe4\\xb3#\\xb5r\\x9c': [-20, 68180108]}\nb'\\xe4\\xb3#\\xb5r\\x9c' bytearray(b'{\"topic\": \"/battery\", \"value\": 97.4}') {b'\\xe4\\xb3#\\xb5r\\x9c': [-20, 68246221]}\nb'\\xe4\\xb3#\\xb5r\\x9c' bytearray(b'{\"topic\": \"/battery\", \"value\": 97.5}') {b'\\xe4\\xb3#\\xb5r\\x9c': [-20, 68312331]}\nb'\\xe4\\xb3#\\xb5r\\x9c' bytearray(b'{\"topic\": \"/battery\", \"value\": 97.6}') {b'\\xe4\\xb3#\\xb5r\\x9c': [-20, 68378442]}\nb'\\xe4\\xb3#\\xb5r\\x9c' bytearray(b'{\"topic\": \"/battery\", \"value\": 97.7}') {b'\\xe4\\xb3#\\xb5r\\x9c': [-20, 68444553]}\nb'\\xe4\\xb3#\\xb5r\\x9c' bytearray(b'{\"topic\": \"/battery\", \"value\": 97.8}') {b'\\xe4\\xb3#\\xb5r\\x9c': [-20, 68510665]}\nb'\\xe4\\xb3#\\xb5r\\x9c' bytearray(b'{\"topic\": \"/battery\", \"value\": 98.0}') {b'\\xe4\\xb3#\\xb5r\\x9c': [-20, 68576776]}\nb'\\xe4\\xb3#\\xb5r\\x9c' bytearray(b'{\"topic\": \"/battery\", \"value\": 98.0}') {b'\\xe4\\xb3#\\xb5r\\x9c': [-20, 68642887]}\nb'\\xe4\\xb3#\\xb5r\\x9c' bytearray(b'{\"topic\": \"/battery\", \"value\": 98.0}') {b'\\xe4\\xb3#\\xb5r\\x9c': [-20, 68709000]}\nb'\\xe4\\xb3#\\xb5r\\x9c' bytearray(b'{\"topic\": \"/battery\", \"value\": 98.0}') {b'\\xe4\\xb3#\\xb5r\\x9c': [-20, 68775110]}\nb'\\xe4\\xb3#\\xb5r\\x9c' bytearray(b'{\"topic\": \"/battery\", \"value\": 98.0}') {b'\\xe4\\xb3#\\xb5r\\x9c': [-20, 68841222]}\nb'\\xe4\\xb3#\\xb5r\\x9c' bytearray(b'{\"topic\": \"/battery\", \"value\": 98.0}') {b'\\xe4\\xb3#\\xb5r\\x9c': [-20, 68907333]}\nb'\\xe4\\xb3#\\xb5r\\x9c' bytearray(b'{\"topic\": \"/battery\", \"value\": 98.0}') {b'\\xe4\\xb3#\\xb5r\\x9c': [-20, 68973445]}\nb'\\xe4\\xb3#\\xb5r\\x9c' bytearray(b'{\"topic\": \"/battery\", \"value\": 98.0}') {b'\\xe4\\xb3#\\xb5r\\x9c': [-20, 69039556]}\nb'\\xe4\\xb3#\\xb5r\\x9c' bytearray(b'{\"topic\": \"/battery\", \"value\": 98.0}') {b'\\xe4\\xb3#\\xb5r\\x9c': [-20, 69105671]}\nb'\\xe4\\xb3#\\xb5r\\x9c' bytearray(b'{\"topic\": \"/battery\", \"value\": 98.0}') {b'\\xe4\\xb3#\\xb5r\\x9c': [-20, 69171781]}\nb'\\xe4\\xb3#\\xb5r\\x9c' bytearray(b'{\"topic\": \"/battery\", \"value\": 98.0}') {b'\\xe4\\xb3#\\xb5r\\x9c': [-20, 69237890]}\nb'\\xe4\\xb3#\\xb5r\\x9c' bytearray(b'{\"topic\": \"/battery\", \"value\": 98.0}') {b'\\xe4\\xb3#\\xb5r\\x9c': [-20, 69304001]}\nb'\\xe4\\xb3#\\xb5r\\x9c' bytearray(b'{\"topic\": \"/battery\", \"value\": 98.0}') {b'\\xe4\\xb3#\\xb5r\\x9c': [-21, 69370115]}\nb'\\xe4\\xb3#\\xb5r\\x9c' bytearray(b'{\"topic\": \"/battery\", \"value\": 98.0}') {b'\\xe4\\xb3#\\xb5r\\x9c': [-20, 69436224]}\nb'\\xe4\\xb3#\\xb5r\\x9c' bytearray(b'{\"topic\": \"/battery\", \"value\": 98.0}') {b'\\xe4\\xb3#\\xb5r\\x9c': [-20, 69502335]}\nb'\\xe4\\xb3#\\xb5r\\x9c' bytearray(b'{\"topic\": \"/battery\", \"value\": 98.0}') {b'\\xe4\\xb3#\\xb5r\\x9c': [-20, 69568447]}\nb'\\xe4\\xb3#\\xb5r\\x9c' bytearray(b'{\"topic\": \"/battery\", \"value\": 98.0}') {b'\\xe4\\xb3#\\xb5r\\x9c': [-20, 69634559]}\nb'\\xe4\\xb3#\\xb5r\\x9c' bytearray(b'{\"topic\": \"/battery\", \"value\": 98.0}') {b'\\xe4\\xb3#\\xb5r\\x9c': [-20, 69700672]}\nb'\\xe4\\xb3#\\xb5r\\x9c' bytearray(b'{\"topic\": \"/battery\", \"value\": 98.0}') {b'\\xe4\\xb3#\\xb5r\\x9c': [-20, 69766781]}\nb'\\xe4\\xb3#\\xb5r\\x9c' bytearray(b'{\"topic\": \"/battery\", \"value\": 98.0}') {b'\\xe4\\xb3#\\xb5r\\x9c': [-20, 69832892]}\nb'\\xe4\\xb3#\\xb5r\\x9c' bytearray(b'{\"topic\": \"/battery\", \"value\": 98.0}') {b'\\xe4\\xb3#\\xb5r\\x9c': [-20, 69899004]}\nb'\\xe4\\xb3#\\xb5r\\x9c' bytearray(b'{\"topic\": \"/battery\", \"value\": 98.0}') {b'\\xe4\\xb3#\\xb5r\\x9c': [-21, 69965115]}\n"
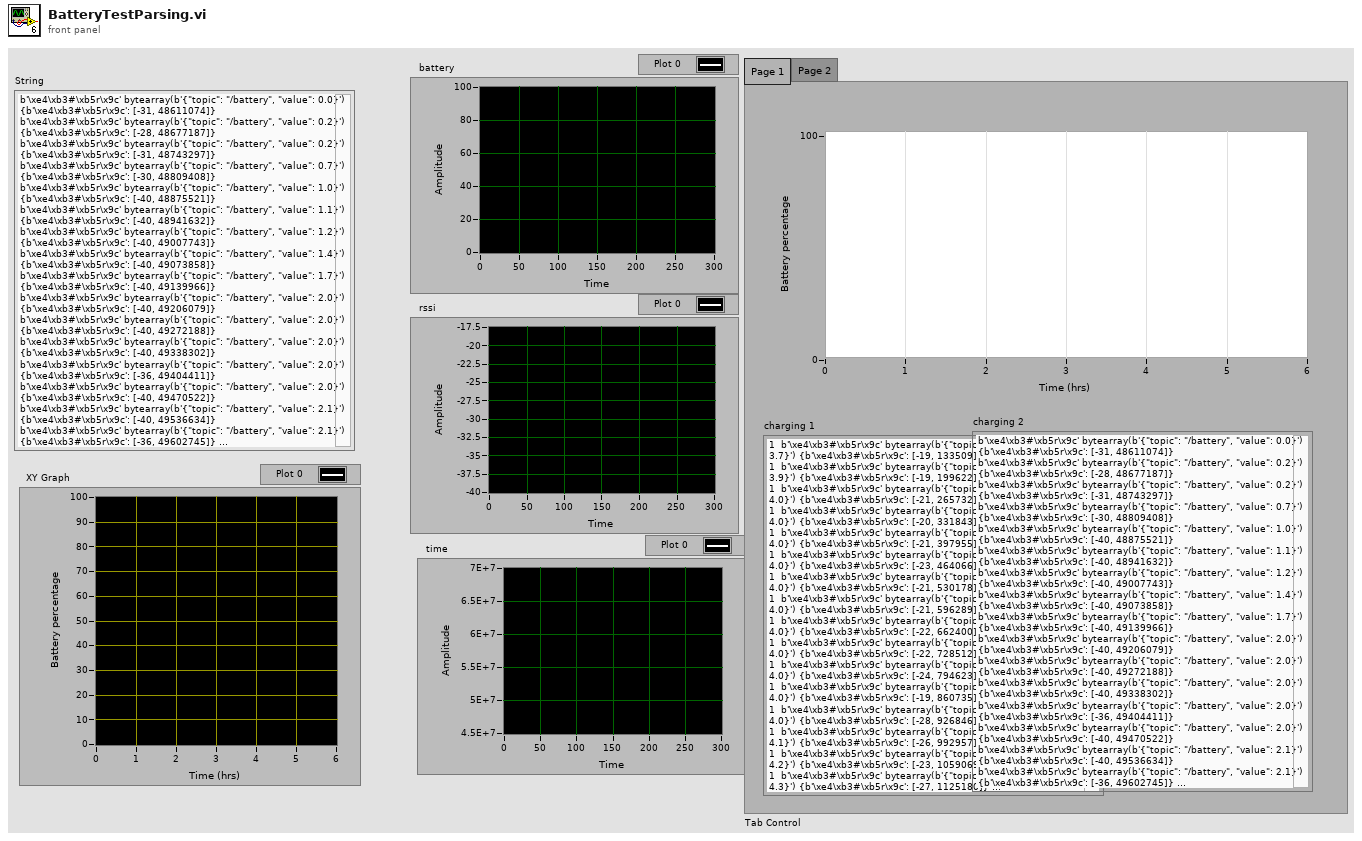
[diagram p1: front panel]
types:
  T1 = cluster{"XY Graph":cluster{"X":dbl, "Y":dbl}[]}[]
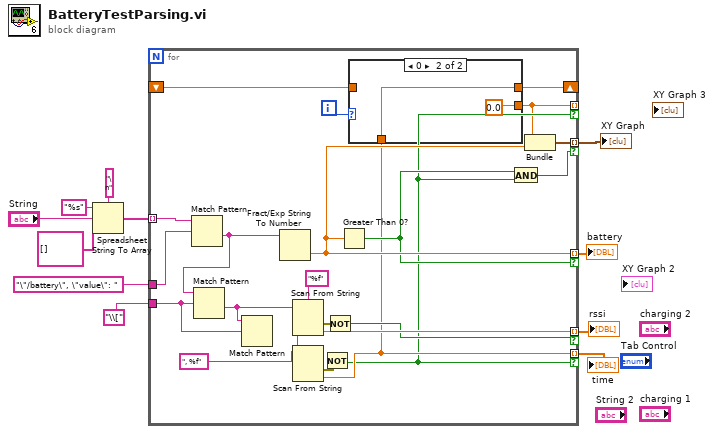
[diagram p0: block diagram]
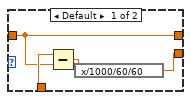
[diagram p2: hidden frame]
diagram:
  n1 = Spreadsheet String To Array(delimiter (Tab)="\n", format string="%s", spreadsheet string="String", array type (2D Dbl)=string[] []) -> (array=w7:string[])
  n2 = for {
    tunnel: w7 -> [w33] mode=indexing
    tunnel: "\"/battery\", \"value\": " ("delimiter (Tab)") -> [w32]
    tunnel: "\\[" ("delimiter (Tab)") -> [w16]
    tunnel: [w30] -> w4 mode=indexing if=w28
    tunnel: [w18] -> w3 mode=indexing if=w13
    tunnel: [w23] -> w2 mode=indexing if=w22
    tunnel: [w21] -> w1 mode=indexing if=w20
    shift-right: [w14] -> _
    shift-left: _ -> [w17]
    tunnel: [w12] -> _ mode=indexing if=w13
    i -> [w19]
    n3 = Match Pattern(string=w33, regular expression=w32) -> (after substring=w31:string)  [unwired: 1 in, 3 out]
    n4 = Match Pattern(string=w31, regular expression=w16) -> (after substring=w15:string)  [unwired: 1 in, 3 out]
    n5 = Match Pattern(string=w15, regular expression=w16) -> ()  [unwired: 1 in, 4 out]
    n6 = Fract/Exp String To Number(string=w31) -> (number=w23:dbl)  [unwired: 3 in, 1 out]
    n7 = Scan From String(format string="%f", input string=w15) -> (remaining string=w27:string, error out=w29:errorcluster, output 1=w30:dbl)  [unwired: 3 in, 1 out]
    n8 = Scan From String(format string=", %f", input string=w27) -> (error out=w25:errorcluster, output 1=w18:dbl)  [unwired: 3 in, 2 out]
    n9 = Not(x=w25) -> (.not. x?=w13:bool)
    n10 = Not(x=w29) -> (.not. x?=w28:bool)
    n11 = Greater Than 0?(x=w23) -> (x > 0?=w22:bool)
    n12 = case shown="0" w19 {
      tunnel: [w34 0.0] -> w12
      tunnel: w18 -> [w37 w39]
      tunnel: [w36 w39] -> w14
      tunnel: w17 -> [w36 _]
      frame Default {
        n13 = Subtract(x=w37, y=w36) -> (x-y=w35:dbl)
        n14 = expression code="x/1000/60/60"(w35) -> (w34:dbl)
      }
      frame 0 {
      }
    }
    n15 = And(x=w22, y=w13) -> (x .and. y?=w20:bool)
    n16 = Bundle(w12, w23) -> (w21:cluster{dbl, dbl})  [unwired: 1 in]
  }
  "rssi" <- w4
  "time" <- w3
  "battery" <- w2
  "XY Graph" <- w1
